vi "Beampointing_Multi_Pico2_upstairs02.vi"() -> ()   [LabVIEW 2013]
uses:
  GUI_Template/GUI_master/tcp_new_data_event.ctl
  GUI_Template/GUI_master/tcp new data cluster.ctl
  Ctrs/beam detection.ctl
  GUI_Beampointing_single_TRA/Ctrs/move.ctl
  <vilib>/Utility/error.llb/DialogType.ctl
  <vilib>/Utility/file.llb/Read From Spreadsheet File (string).vi
  <userlib>/_OpenG.lib/array/array.llb/Filter 1D Array with Scalar (String)__ogtk.vi
  <userlib>/_OpenG.lib/array/array.llb/Filter 1D Array (String)__ogtk.vi
  <vilib>/Utility/file.llb/Write To Spreadsheet File (string).vi
  <vilib>/Analysis/NI_AALBase.lvlib
panel:
  out "x-y*floor(x/y)":dbl
  out "error out":errorcluster
  out "config path":string
  out "Array 3":bool[](array[boolean])
  out "Array 2":u16[](array[numeric])
  out "Array":u16[](array[numeric])
  out "Moving Y":string
  out "Moving X":string
  out "particles":T1(array[cluster])
  out "millisecond timer value":u32
  out "appended path":path
  out "millisecond timer 2":u32
  in  "GUIdevice 98":string="PicoPad4"
  in  "Position.Axis 111::98":dbl=77.0 caption="Motor Axis 1" min=-30000.0 max=30000.0 format="%#_6f"
  in  "Position.Axis 112::98":dbl=77.0 caption="Motor Axis 1" min=-20000.0 max=20000.0 format="%#_6f"
  in  "Position.Axis 113::98":dbl=77.0 caption="Motor Axis 1" min=-20000.0 max=20000.0 format="%#_6f"
  in  "Position.Axis 121::98":dbl=77.0 caption="Motor Axis 1" min=-999999.0 max=999999.0 format="%#_6f"
  in  "Position.Axis 122::98":dbl=77.0 caption="Motor Axis 1" min=-999999.0 max=999999.0 format="%#_6f"
  in  "Position.Axis 123::98":dbl=77.0 caption="Motor Axis 1" min=-999999.0 max=999999.0 format="%#_6f"
  in  "Position.Axis 131::98":dbl=77.0 caption="Motor Axis 1" min=-999999.0 max=999999.0 format="%#_6f"
  in  "Position.Axis 132::98":dbl=77.0 caption="Motor Axis 1" min=-999999.0 max=999999.0 format="%#_6f"
  in  "Position.Axis 133::98":dbl=77.0 caption="Motor Axis 1" min=-999999.0 max=999999.0 format="%#_6f"
  in  "Position.Axis 141::98":dbl=77.0 caption="Motor Axis 1" min=-999999.0 max=999999.0 format="%#_6f"
  in  "Position.Axis 142::98":dbl=77.0 caption="Motor Axis 1" min=-999999.0 max=999999.0 format="%#_6f"
  in  "Position.Axis 143::98":dbl=77.0 caption="Motor Axis 1" min=-999999.0 max=999999.0 format="%#_6f"
  in  "Position.Axis 211::98":dbl=77.0 caption="Motor Axis 1" min=-999999.0 max=999999.0 format="%#_6f"
  in  "Position.Axis 212::98":dbl=77.0 caption="Motor Axis 1" min=-999999.0 max=999999.0 format="%#_6f"
  in  "Position.Axis 213::98":dbl=77.0 caption="Motor Axis 1" min=-999999.0 max=999999.0 format="%#_6f"
  in  "Position.Axis 221::98":dbl=77.0 caption="Motor Axis 1" min=-999999.0 max=999999.0 format="%#_6f"
  in  "Position.Axis 222::98":dbl=77.0 caption="Motor Axis 1" min=-999999.0 max=999999.0 format="%#_6f"
  in  "Position.Axis 223::98":dbl=77.0 caption="Motor Axis 1" min=-999999.0 max=999999.0 format="%#_6f"
  in  "Position.Axis 231::98":dbl=77.0 caption="Motor Axis 1" min=-999999.0 max=999999.0 format="%#_6f"
  in  "Position.Axis 232::98":dbl=77.0 caption="Motor Axis 1" min=-999999.0 max=999999.0 format="%#_6f"
  in  "Position.Axis 233::98":dbl=77.0 caption="Motor Axis 1" min=-999999.0 max=999999.0 format="%#_6f"
  in  "Position.Axis 241::98":dbl=77.0 caption="Motor Axis 1" min=-999999.0 max=999999.0 format="%#_6f"
  in  "Position.Axis 242::98":dbl=77.0 caption="Motor Axis 1" min=-999999.0 max=999999.0 format="%#_6f"
  in  "Position.Axis 243::98":dbl=77.0 caption="Motor Axis 1" min=-999999.0 max=999999.0 format="%#_6f"
  in  "Position.Axis 311::98":dbl=77.0 caption="Motor Axis 1" min=-999999.0 max=999999.0 format="%#_6f"
  in  "Position.Axis 312::98":dbl=77.0 caption="Motor Axis 1" min=-999999.0 max=999999.0 format="%#_6f"
  in  "Position.Axis 313::98":dbl=77.0 caption="Motor Axis 1" min=-999999.0 max=999999.0 format="%#_6f"
  in  "Position.Axis 321::98":dbl=77.0 caption="Motor Axis 1" min=-999999.0 max=999999.0 format="%#_6f"
  in  "Position.Axis 322::98":dbl=77.0 caption="Motor Axis 1" min=-999999.0 max=999999.0 format="%#_6f"
  in  "Position.Axis 323::98":dbl=77.0 caption="Motor Axis 1" min=-999999.0 max=999999.0 format="%#_6f"
  in  "Position.Axis 331::98":dbl=77.0 caption="Motor Axis 1" min=-999999.0 max=999999.0 format="%#_6f"
  in  "Position.Axis 332::98":dbl=77.0 caption="Motor Axis 1" min=-999999.0 max=999999.0 format="%#_6f"
  in  "Position.Axis 333::98":dbl=77.0 caption="Motor Axis 1" min=-999999.0 max=999999.0 format="%#_6f"
  in  "Position.Axis 341::98":dbl=77.0 caption="Motor Axis 1" min=-999999.0 max=999999.0 format="%#_6f"
  in  "Position.Axis 342::98":dbl=77.0 caption="Motor Axis 1" min=-999999.0 max=999999.0 format="%#_6f"
  in  "Position.Axis 343::98":dbl=77.0 caption="Motor Axis 1" min=-999999.0 max=999999.0 format="%#_6f"
  in  "Position.Axis 411::98":dbl=77.0 caption="Motor Axis 1" min=-999999.0 max=999999.0 format="%#_6f"
  in  "Position.Axis 412::98":dbl=77.0 caption="Motor Axis 1" min=-999999.0 max=999999.0 format="%#_6f"
  in  "Position.Axis 413::98":dbl=77.0 caption="Motor Axis 1" min=-999999.0 max=999999.0 format="%#_6f"
  in  "Position.Axis 421::98":dbl=77.0 caption="Motor Axis 1" min=-999999.0 max=999999.0 format="%#_6f"
  in  "Position.Axis 422::98":dbl=77.0 caption="Motor Axis 1" min=-999999.0 max=999999.0 format="%#_6f"
  in  "Position.Axis 423::98":dbl=77.0 caption="Motor Axis 1" min=-999999.0 max=999999.0 format="%#_6f"
  in  "Position.Axis 431::98":dbl=77.0 caption="Motor Axis 1" min=-999999.0 max=999999.0 format="%#_6f"
  in  "Position.Axis 432::98":dbl=77.0 caption="Motor Axis 1" min=-999999.0 max=999999.0 format="%#_6f"
  in  "Position.Axis 433::98":dbl=77.0 caption="Motor Axis 1" min=-999999.0 max=999999.0 format="%#_6f"
  in  "Position.Axis 441::98":dbl=77.0 caption="Motor Axis 1" min=-999999.0 max=999999.0 format="%#_6f"
  in  "Position.Axis 442::98":dbl=77.0 caption="Motor Axis 1" min=-999999.0 max=999999.0 format="%#_6f"
  in  "Position.Axis 443::98":dbl=77.0 caption="Motor Axis 1" min=-999999.0 max=999999.0 format="%#_6f"
  in  "Position.Axis 511::98":dbl=77.0 caption="Motor Axis 1" min=-999999.0 max=999999.0 format="%#_6f"
  in  "Position.Axis 512::98":dbl=77.0 caption="Motor Axis 1" min=-999999.0 max=999999.0 format="%#_6f"
  in  "Position.Axis 513::98":dbl=77.0 caption="Motor Axis 1" min=-999999.0 max=999999.0 format="%#_6f"
  in  "Position.Axis 521::98":dbl=77.0 caption="Motor Axis 1" min=-999999.0 max=999999.0 format="%#_6f"
  in  "Position.Axis 522::98":dbl=77.0 caption="Motor Axis 1" min=-999999.0 max=999999.0 format="%#_6f"
  in  "Position.Axis 523::98":dbl=77.0 caption="Motor Axis 1" min=-999999.0 max=999999.0 format="%#_6f"
  in  "Position.Axis 531::98":dbl=77.0 caption="Motor Axis 1" min=-999999.0 max=999999.0 format="%#_6f"
  in  "Position.Axis 532::98":dbl=77.0 caption="Motor Axis 1" min=-999999.0 max=999999.0 format="%#_6f"
  in  "Position.Axis 533::98":dbl=77.0 caption="Motor Axis 1" min=-999999.0 max=999999.0 format="%#_6f"
  in  "Position.Axis 541::98":dbl=77.0 caption="Motor Axis 1" min=-999999.0 max=999999.0 format="%#_6f"
  in  "Position.Axis 542::98":dbl=77.0 caption="Motor Axis 1" min=-999999.0 max=999999.0 format="%#_6f"
  in  "Position.Axis 543::98":dbl=77.0 caption="Motor Axis 1" min=-999999.0 max=999999.0 format="%#_6f"
  in  "Numeric":dbl
  out "Current State":string
  in  "output cluster 2":T5 {"detection para"."smal para"."Measurement Parameter" items=["Center of Mass X", "Center of Mass Y", "First Pixel X", "First Pixel Y", "Bounding Rect Left", "Bounding Rect Top", "Bounding Rect Right", "Bounding Rect Bottom", "Max Feret Diameter Start X", "Max Feret Diameter Start Y", "Max Feret Diameter End X", "Max Feret Diameter End Y", "Max Horiz. Segment Length Left", "Max Horiz. Segment Length Right", "Max Horiz. Segment Length Row", "-", "Bounding Rect Width", "Bounding Rect Height", "Bounding Rect Diagonal", "Perimeter", "Convex Hull Perimeter", "Holes' Perimeter", "Max Feret Diameter", "Equivalent Ellipse Major Axis", "Equivalent Ellipse Minor Axis", "Equivalent Ellipse Minor Axis (Feret)", "Equivalent Rect Long Side", "Equivalent Rect Short Side", "Equivalent Rect Diagonal", "Equivalent Rect Short Side (Feret)", "Average Horiz. Segment Length", "Average Vert. Segment Length", "Hydraulic Radius", "Waddel Disk Diameter", "-", "Area", "Holes' Area", "Particle & Holes' Area", "Convex Hull Area", "Image Area", "-", "Number of Holes", "Number of Horiz. Segments", "Number of Vert. Segments", "-", "Orientation", "Max Feret Diameter Orientation", "-", "% Area/Image Area", "% Area/(Particle & Holes' Area)", "Ratio of Equivalent Ellipse Axes", "Ratio of Equivalent Rect Sides", "-", "Elongation Factor", "Compactness Factor", "Heywood Circularity Factor", "Type Factor", "-", "Sum X", "Sum Y", "Sum XX", "Sum XY", "Sum YY", "Sum XXX", "Sum XXY", "Sum XYY", "Sum YYY", "-", "Moment of Inertia XX", "Moment of Inertia XY", "Moment of Inertia YY", "Moment of Inertia XXX", "Moment of Inertia XXY", "Moment of Inertia XYY", "Moment of Inertia YYY", "Norm. Moment of Inertia XX", "Norm. Moment of Inertia XY", "Norm. Moment of Inertia YY", "Norm. Moment of Inertia XXX", "Norm. Moment of Inertia XXY", "Norm. Moment of Inertia XYY", "Norm. Moment of Inertia YYY", "Hu Moment 1", "Hu Moment 2", "Hu Moment 3", "Hu Moment 4", "Hu Moment 5", "Hu Moment 6", "Hu Moment 7"]; "detection para"."smal para"."Range Lower Value" format="%.2f"; "detection para"."smal para"."Range Upper Value" format="%.2f"; "detection para"."detection method" items=["clustering", "entropy", "metric", "moments", "inter-class variance"]; "detection para"."Filter" items=["No Filter", "Median Filter", "Low Pass Filter"]}
  out "CCDs":string[](array[string])
  in  "GUIdevice 12":string
  in  "GUIdevice 11":string
  in  "GUIdevice 10":string
  in  "GUIdevice 9":string
  out "error out 2":errorcluster
  in  "active cams":string[](array[string])
  in  "Motor Y":dbl[][](array[numeric])
  in  "Motor X":dbl[][](array[numeric])
  out "Names":string[](array[string])
  in  "Offset X stats":dbl[][](array[numeric])
  in  "Offset Y stats":dbl[][](array[numeric])
  out "Box":T6(array[cluster])
  in  "Tab Control 2":enum32{"Config ", "Main", "History"}(tab)=enum."Main"
  out "Waveform Chart":u32(graph)
  in  "associated motors":T7
  out "Cameras":T8
  out "Status":cluster{i32, i32, "Centroid X":dbl[][]}(graph)
  in  "Exposure:12":dbl=0.095 min=0.0001 max=1.0 format="%#_6f"
  in  "Triggerdelay::12":dbl=0.003 min=0.0 max=0.09 format="%#_6f"
  in  "Exposure::11":dbl=0.095 min=0.0001 max=1.0 format="%#_6f"
  in  "Triggerdelay::11":dbl=0.003 min=0.0 max=0.09 format="%#_6f"
  in  "Exposure::10":dbl=0.095 min=0.0001 max=1.0 format="%#_6f"
  in  "Triggerdelay::10":dbl=0.003 min=0.0 max=0.09 format="%#_6f"
  in  "Exposure::9":dbl=0.095 min=0.0001 max=1.0 format="%#_6f"
  in  "Triggerdelay::9":dbl=0.003 min=0.0 max=0.09 format="%#_6f"
  in  "Trigger::9":bool
  in  "Trigger::10":bool caption="Trigger:10"
  in  "Trigger::11":bool
  in  "Trigger::12":bool
  in  "Target.Y::9":dbl=45.0 caption="T9y" min=0.0 max=2000.0 format="%#_6f"
  in  "Target.X::9":dbl=47.0 caption="Tx9" min=0.0 max=2000.0 format="%#_6f"
  in  "Target.Y::10":dbl=45.0 caption="T10y" min=0.0 max=2000.0 format="%#_6f"
  in  "Target.X::10":dbl=47.0 caption="T10x" min=0.0 max=2000.0 format="%#_6f"
  in  "Target.Y::11":dbl=45.0 caption="T11y" min=0.0 max=2000.0 format="%#_6f"
  in  "Target.X::11":dbl=47.0 caption="T11x" min=0.0 max=2000.0 format="%#_6f"
  in  "Target.Y::12":dbl=45.0 caption="T12y" min=0.0 max=2000.0 format="%#_6f"
  in  "Target.X::12":dbl=47.0 caption="T12x" min=0.0 max=2000.0 format="%#_6f"
  in  "Exposure::8":dbl=0.095 min=0.01 max=1.0 format="%#_6f"
  in  "Triggerdelay::8":dbl=0.003 min=0.0 max=0.09 format="%#_6f"
  in  "Trigger::8":bool
  in  "Target.Y::8":dbl=45.0 caption="T8y" min=0.0 max=2000.0 format="%#_6f"
  in  "Target.X::8":dbl=47.0 caption="T8x" min=0.0 max=2000.0 format="%#_6f"
  in  "Target.Y::7":dbl=45.0 caption="T7x" min=0.0 max=2000.0 format="%#_6f"
  in  "Target.X::7":dbl=47.0 caption="T7y" min=0.0 max=2000.0 format="%#_6f"
  in  "Target.Y::6":dbl=45.0 caption="T6y" min=0.0 max=2000.0 format="%#_6f"
  in  "Target.X::6":dbl=47.0 caption="T6x" min=0.0 max=2000.0 format="%#_6f"
  in  "Target.Y::5":dbl=45.0 caption="T5y" min=0.0 max=2000.0 format="%#_6f"
  in  "Target.X::5":dbl=47.0 caption="T5x" min=0.0 max=2000.0 format="%#_6f"
  in  "Target.Y::4":dbl=45.0 caption="T4y" min=0.0 max=2000.0 format="%#_6f"
  in  "Target.X::4":dbl=47.0 caption="T4x" min=0.0 max=2000.0 format="%#_6f"
  in  "Target.Y::3":dbl=163.0 caption="T3y" min=0.0 max=2000.0 format="%#_6f"
  in  "Target.X::3":dbl=152.0 caption="T3x" min=0.0 max=2000.0 format="%#_6f"
  in  "Target.Y::2":dbl=74.0 caption="T2y" min=0.0 max=2000.0 format="%#_6f"
  in  "Target.X::2":dbl=75.0 caption="T2x" min=0.0 max=2000.0 format="%#_6f"
  in  "Target.Y::1":dbl=61.0 caption="T1y" min=1.0 max=600.0 format="%#_6f"
  in  "Target.X::1":dbl=77.0 caption="T1x" min=1.0 max=800.0 format="%#_6f"
  in  "Exposure::7":dbl=0.095 min=0.0001 max=1.0 format="%#_6f"
  in  "Triggerdelay::7":dbl=0.003 min=0.0 max=0.09 format="%#_6f"
  in  "Trigger::7":bool
  in  "Exposure::6":dbl=0.095 min=0.0001 max=1.0 format="%#_6f"
  in  "Triggerdelay::6":dbl=0.003 min=0.0 max=0.09 format="%#_6f"
  in  "Trigger::6":bool
  in  "Exposure::5":dbl=0.095 min=0.0001 max=1.0 format="%#_6f"
  in  "Triggerdelay::5":dbl=0.003 min=0.0 max=0.09 format="%#_6f"
  in  "Trigger::5":bool
  in  "Exposure::4":dbl=0.095 min=0.0001 max=1.0 format="%#_6f"
  in  "Triggerdelay::4":dbl=0.003 min=0.0 max=0.09 format="%#_6f"
  in  "Trigger::4":bool
  in  "Exposure::3":dbl=0.095 min=0.0001 max=1.0 format="%#_6f"
  in  "Triggerdelay::3":dbl=0.003 min=0.0 max=0.09 format="%#_6f"
  in  "Trigger::3":bool
  in  "Exposure::2":dbl=0.095 min=0.0001 max=1.0 format="%#_6f"
  in  "Triggerdelay::2":dbl=0.003 min=0.0 max=0.09 format="%#_6f"
  in  "Trigger::2":bool
  out "image::1":T9(plugin-control) caption="XPW_cam"
  out "image::2":T9(plugin-control) caption="LM_Mirrorcam"
  out "image::3":T9(plugin-control) caption="LM_Focuscam"
  out "image::4":T9(plugin-control) caption="TS-253a_in"
  out "image::5":T9(plugin-control) caption="LM_Stagecam"
  out "image::6":T9(plugin-control)
  out "image::7":T9(plugin-control)
  out "image::8":T9(plugin-control)
  in  "Exposure::1":dbl=0.095 min=0.0001 max=1.0 format="%#_6f"
  in  "Triggerdelay::1":dbl=0.003 min=0.0 max=0.09 format="%#_6f"
  in  "Trigger::1":bool
  in  "UDP error message":string
  out "required Y":bool[](array[boolean])
  out "required X":bool[](array[boolean])
  out "detected":bool[](array[boolean])
  out "name array":string[](array[string])
  out "image::9":T9(plugin-control)
  out "image::10":T9(plugin-control)
  out "image::11":T9(plugin-control)
  out "image::12":T9(plugin-control)
  out "speedmode X":bool[](array[boolean])
  out "speedmode Y":bool[](array[boolean])
  out "CCD 9":cluster{timestamp[], dbl[]}[](graph)
  out "CCD 10":cluster{timestamp[], dbl[]}[](graph)
  out "CCD 11":cluster{timestamp[], dbl[]}[](graph)
  out "CCD 12":cluster{timestamp[], dbl[]}[](graph)
  out "CCD 5":cluster{timestamp[], dbl[]}[](graph)
  out "CCD 6":cluster{timestamp[], dbl[]}[](graph)
  out "CCD 7":cluster{timestamp[], dbl[]}[](graph)
  out "CCD 8":cluster{timestamp[], dbl[]}[](graph)
  out "CCD 2":cluster{timestamp[], dbl[]}[](graph)
  out "CCD 1":cluster{timestamp[], dbl[]}[](graph)
  out "CCD 3":cluster{timestamp[], dbl[]}[](graph)
  out "CCD 4":cluster{timestamp[], dbl[]}[](graph)
  out "History index":i32
  in  "History Size":i32=500
  out "Particle Reports (Pixels)":T10(array[cluster])
  in  "Feedback Global":bool
  in  "detection para":T3[](array[typedef])=[{"Filter"=1, "Filter Para"={"X Size"=5, "Y Size"=5, "% Tolerance"=1}, "detection method"=4, "smal para"=[{"Measurement Parameter"=35, "Range Lower Value"=0.0, "Range Upper Value"=0.0, "Range"=TRUE, "Measurement Type"=FALSE}], "Remove small Objects"=TRUE, "Restrict to round Objects"=FALSE}, {"Filter"=1, "Filter Para"={"X Size"=5, "Y Size"=5, "% Tolerance"=1}, "detection method"=4, "smal para"=[{"Measurement Parameter"=35, "Range Lower Value"=0.0, "Range Upper Value"=500.0, "Range"=FALSE, "Measurement Type"=FALSE}], "Remove small Objects"=TRUE, "Restrict to round Objects"=FALSE}, {"Filter"=1, "Filter Para"={"X Size"=5, "Y Size"=5, "% Tolerance"=1}, "detection method"=4, "smal para"=[{"Measurement Parameter"=35, "Range Lower Value"=0.0, "Range Upper Value"=500.0, "Range"=TRUE, "Measurement Type"=FALSE}], "Remove small Objects"=TRUE, "Restrict to round Objects"=FALSE}, {"Filter"=1, "Filter Para"={"X Size"=5, "Y Size"=5, "% Tolerance"=1}, "detection method"=4, "smal para"=[{"Measurement Parameter"=35, "Range Lower Value"=0.0, "Range Upper Value"=500.0, "Range"=TRUE, "Measurement Type"=FALSE}], "Remove small Objects"=TRUE, "Restrict to round Objects"=FALSE}, {"Filter"=1, "Filter Para"={"X Size"=5, "Y Size"=5, "% Tolerance"=1}, "detection method"=4, "smal para"=[{"Measurement Parameter"=35, "Range Lower Value"=0.0, "Range Upper Value"=500.0, "Range"=TRUE, "Measurement Type"=FALSE}], "Remove small Objects"=TRUE, "Restrict to round Objects"=FALSE}, {"Filter"=1, "Filter Para"={"X Size"=5, "Y Size"=5, "% Tolerance"=1}, "detection method"=4, "smal para"=[{"Measurement Parameter"=35, "Range Lower Value"=0.0, "Range Upper Value"=500.0, "Range"=TRUE, "Measurement Type"=FALSE}], "Remove small Objects"=TRUE, "Restrict to round Objects"=FALSE}, {"Filter"=1, "Filter Para"={"X Size"=5, "Y Size"=5, "% Tolerance"=1}, "detection method"=4, "smal para"=[{"Measurement Parameter"=35, "Range Lower Value"=0.0, "Range Upper Value"=500.0, "Range"=TRUE, "Measurement Type"=FALSE}], "Remove small Objects"=TRUE, "Restrict to round Objects"=FALSE}, {"Filter"=1, "Filter Para"={"X Size"=5, "Y Size"=5, "% Tolerance"=1}, "detection method"=3, "smal para"=[{"Measurement Parameter"=35, "Range Lower Value"=0.0, "Range Upper Value"=0.0, "Range"=FALSE, "Measurement Type"=FALSE}], "Remove small Objects"=TRUE, "Restrict to round Objects"=FALSE}, {"Filter"=1, "Filter Para"={"X Size"=5, "Y Size"=5, "% Tolerance"=1}, "detection method"=4, "smal para"=[{"Measurement Parameter"=35, "Range Lower Value"=0.0, "Range Upper Value"=0.0, "Range"=FALSE, "Measurement Type"=FALSE}], "Remove small Objects"=TRUE, "Restrict to round Objects"=FALSE}, {"Filter"=1, "Filter Para"={"X Size"=5, "Y Size"=5, "% Tolerance"=1}, "detection method"=4, "smal para"=[{"Measurement Parameter"=35, "Range Lower Value"=0.0, "Range Upper Value"=500.0, "Range"=TRUE, "Measurement Type"=FALSE}], "Remove small Objects"=TRUE, "Restrict to round Objects"=FALSE}, {"Filter"=1, "Filter Para"={"X Size"=5, "Y Size"=5, "% Tolerance"=1}, "detection method"=4, "smal para"=[{"Measurement Parameter"=35, "Range Lower Value"=0.0, "Range Upper Value"=500.0, "Range"=TRUE, "Measurement Type"=FALSE}], "Remove small Objects"=TRUE, "Restrict to round Objects"=FALSE}, {"Filter"=1, "Filter Para"={"X Size"=5, "Y Size"=5, "% Tolerance"=1}, "detection method"=4, "smal para"=[{"Measurement Parameter"=35, "Range Lower Value"=0.0, "Range Upper Value"=500.0, "Range"=TRUE, "Measurement Type"=FALSE}], "Remove small Objects"=TRUE, "Restrict to round Objects"=FALSE}] {"smal para"."Measurement Parameter" items=["Center of Mass X", "Center of Mass Y", "First Pixel X", "First Pixel Y", "Bounding Rect Left", "Bounding Rect Top", "Bounding Rect Right", "Bounding Rect Bottom", "Max Feret Diameter Start X", "Max Feret Diameter Start Y", "Max Feret Diameter End X", "Max Feret Diameter End Y", "Max Horiz. Segment Length Left", "Max Horiz. Segment Length Right", "Max Horiz. Segment Length Row", "-", "Bounding Rect Width", "Bounding Rect Height", "Bounding Rect Diagonal", "Perimeter", "Convex Hull Perimeter", "Holes' Perimeter", "Max Feret Diameter", "Equivalent Ellipse Major Axis", "Equivalent Ellipse Minor Axis", "Equivalent Ellipse Minor Axis (Feret)", "Equivalent Rect Long Side", "Equivalent Rect Short Side", "Equivalent Rect Diagonal", "Equivalent Rect Short Side (Feret)", "Average Horiz. Segment Length", "Average Vert. Segment Length", "Hydraulic Radius", "Waddel Disk Diameter", "-", "Area", "Holes' Area", "Particle & Holes' Area", "Convex Hull Area", "Image Area", "-", "Number of Holes", "Number of Horiz. Segments", "Number of Vert. Segments", "-", "Orientation", "Max Feret Diameter Orientation", "-", "% Area/Image Area", "% Area/(Particle & Holes' Area)", "Ratio of Equivalent Ellipse Axes", "Ratio of Equivalent Rect Sides", "-", "Elongation Factor", "Compactness Factor", "Heywood Circularity Factor", "Type Factor", "-", "Sum X", "Sum Y", "Sum XX", "Sum XY", "Sum YY", "Sum XXX", "Sum XXY", "Sum XYY", "Sum YYY", "-", "Moment of Inertia XX", "Moment of Inertia XY", "Moment of Inertia YY", "Moment of Inertia XXX", "Moment of Inertia XXY", "Moment of Inertia XYY", "Moment of Inertia YYY", "Norm. Moment of Inertia XX", "Norm. Moment of Inertia XY", "Norm. Moment of Inertia YY", "Norm. Moment of Inertia XXX", "Norm. Moment of Inertia XXY", "Norm. Moment of Inertia XYY", "Norm. Moment of Inertia YYY", "Hu Moment 1", "Hu Moment 2", "Hu Moment 3", "Hu Moment 4", "Hu Moment 5", "Hu Moment 6", "Hu Moment 7"]; "smal para"."Range Lower Value" format="%.2f"; "smal para"."Range Upper Value" format="%.2f"; "detection method" items=["clustering", "entropy", "metric", "moments", "inter-class variance"]; "Filter" items=["No Filter", "Median Filter", "Low Pass Filter"]}
  in  "GUIdevice 8":string="B5_CompressorOut"
  in  "Tab Control":T11(tab)
  in  "Center":bool
  in  "Save Stats":bool
  in  "Save Config":bool
  in  "Load Config":bool
  in  "update speed [ms]":i32=200
  in  "Img to avg":i32=20 min=3 max=200
  in  "Reset History":bool
  in  "save path":path=path "W:/BP_DATA"
  in  "autodetect":bool
  in  "Detection Rate":dbl=0.8 min=0.001 max=1.0
  in  "new tdms":bool
  in  "Speedmode @":dbl=3.0 min=1.0 max=20.0
  in  "Align":bool
  in  "deivice ini":bool
  in  "beam detection para":T3={"Filter"=1, "Filter Para"={"X Size"=5, "Y Size"=5, "% Tolerance"=1}, "detection method"=4, "smal para"=[{"Measurement Parameter"=35, "Range Lower Value"=0.0, "Range Upper Value"=500.0, "Range"=FALSE, "Measurement Type"=FALSE}], "Remove small Objects"=TRUE, "Restrict to round Objects"=FALSE} {"smal para"."Measurement Parameter" items=["Center of Mass X", "Center of Mass Y", "First Pixel X", "First Pixel Y", "Bounding Rect Left", "Bounding Rect Top", "Bounding Rect Right", "Bounding Rect Bottom", "Max Feret Diameter Start X", "Max Feret Diameter Start Y", "Max Feret Diameter End X", "Max Feret Diameter End Y", "Max Horiz. Segment Length Left", "Max Horiz. Segment Length Right", "Max Horiz. Segment Length Row", "-", "Bounding Rect Width", "Bounding Rect Height", "Bounding Rect Diagonal", "Perimeter", "Convex Hull Perimeter", "Holes' Perimeter", "Max Feret Diameter", "Equivalent Ellipse Major Axis", "Equivalent Ellipse Minor Axis", "Equivalent Ellipse Minor Axis (Feret)", "Equivalent Rect Long Side", "Equivalent Rect Short Side", "Equivalent Rect Diagonal", "Equivalent Rect Short Side (Feret)", "Average Horiz. Segment Length", "Average Vert. Segment Length", "Hydraulic Radius", "Waddel Disk Diameter", "-", "Area", "Holes' Area", "Particle & Holes' Area", "Convex Hull Area", "Image Area", "-", "Number of Holes", "Number of Horiz. Segments", "Number of Vert. Segments", "-", "Orientation", "Max Feret Diameter Orientation", "-", "% Area/Image Area", "% Area/(Particle & Holes' Area)", "Ratio of Equivalent Ellipse Axes", "Ratio of Equivalent Rect Sides", "-", "Elongation Factor", "Compactness Factor", "Heywood Circularity Factor", "Type Factor", "-", "Sum X", "Sum Y", "Sum XX", "Sum XY", "Sum YY", "Sum XXX", "Sum XXY", "Sum XYY", "Sum YYY", "-", "Moment of Inertia XX", "Moment of Inertia XY", "Moment of Inertia YY", "Moment of Inertia XXX", "Moment of Inertia XXY", "Moment of Inertia XYY", "Moment of Inertia YYY", "Norm. Moment of Inertia XX", "Norm. Moment of Inertia XY", "Norm. Moment of Inertia YY", "Norm. Moment of Inertia XXX", "Norm. Moment of Inertia XXY", "Norm. Moment of Inertia XYY", "Norm. Moment of Inertia YYY", "Hu Moment 1", "Hu Moment 2", "Hu Moment 3", "Hu Moment 4", "Hu Moment 5", "Hu Moment 6", "Hu Moment 7"]; "smal para"."Range Lower Value" format="%.2f"; "smal para"."Range Upper Value" format="%.2f"; "detection method" items=["clustering", "entropy", "metric", "moments", "inter-class variance"]; "Filter" items=["No Filter", "Median Filter", "Low Pass Filter"]}
  in  "move config":T2={"Tolerance [%]"=0.1, "Stepsize"=0.0001, "Invert Axis"=TRUE, "Invert Direction X"=FALSE, "Invert Direction Y"=TRUE, "enable feedback"=FALSE, "Set Centriod Target"=FALSE}
  in  "ActiveMotor":u16(ring)=7 items=["XPW OUT SAL", "Pre-IN-SAL", "XPW_cam", "L1_TelInpNear", "A", "B", "a", "D", "PRE-3RD-OUT", "TSa", "", "", "Focuscam", "Mirrorcam", "", "", "", "", "", ""]
  in  "ActiveMotorName::99":string
  in  "RelativeMove.Axis 1.CCW::99":bool caption="RelativeMove.Axis 1.CCW::1"
  in  "RelativeMove.Axis 1.CW::99":bool caption="RelativeMove.Axis 1.CW::1"
  in  "RelativeMove.Axis 2.CCW::99":bool caption="RelativeMove.Axis. 2.CCW::1"
  in  "RelativeMove.Axis 2.CW::99":bool caption="RelativeMove.Axis 2.CW::1"
  in  "RelativeSettings.Axis 1.Position::99":dbl caption="Axis 1 Position" min=-999999.0 max=999999.0 format="%_4p"
  in  "RelativeSettings.Axis 2.Position::99":dbl caption="Axis 2 Position" min=-999999.0 max=999999.0 format="%_4p"
  in  "RelativeSettings.Axis 2.StepSize::99":dbl=50.0 caption="Axis 2 StepSize" min=0.0 max=999999.0 format="%_4p"
  in  "RelativeSettings.Axis 1.StepSize::99":dbl=50.0 caption="Axis 1 Stepsize" min=0.0 max=999999.0 format="%_4p"
  out "Arguments Y":string
  in  "active axis refs 2":T12(array[cluster])
  in  "active Axis ref":cluster{"Ref X":refnum<vi>, "Ref Y":refnum<vi>}
  in  "CCDs":u16(ring) items=["XPW_cam", "LM_Mirrorcam", "LM_Focuscam", "TS-253a_in", "LM_Stagecam", "", "", "", "", "", "", ""]
  out "motor refs":refnum<vi>[](array[refnum])
  in  "Position.Axis 511::99":dbl=77.0 caption="Motor Axis 1" min=-999999.0 max=999999.0 format="%#_6f"
  in  "Position.Axis 512::99":dbl=77.0 caption="Motor Axis 1" min=-999999.0 max=999999.0 format="%#_6f"
  in  "Position.Axis 513::99":dbl=77.0 caption="Motor Axis 1" min=-999999.0 max=999999.0 format="%#_6f"
  in  "Position.Axis 521::99":dbl=77.0 caption="Motor Axis 1" min=-999999.0 max=999999.0 format="%#_6f"
  in  "Position.Axis 522::99":dbl=77.0 caption="Motor Axis 1" min=-999999.0 max=999999.0 format="%#_6f"
  in  "Position.Axis 523::99":dbl=77.0 caption="Motor Axis 1" min=-999999.0 max=999999.0 format="%#_6f"
  in  "Position.Axis 531::99":dbl=77.0 caption="Motor Axis 1" min=-999999.0 max=999999.0 format="%#_6f"
  in  "Position.Axis 532::99":dbl=77.0 caption="Motor Axis 1" min=-999999.0 max=999999.0 format="%#_6f"
  in  "Position.Axis 533::99":dbl=77.0 caption="Motor Axis 1" min=-999999.0 max=999999.0 format="%#_6f"
  in  "Position.Axis 541::99":dbl=77.0 caption="Motor Axis 1" min=-999999.0 max=999999.0 format="%#_6f"
  in  "Position.Axis 542::99":dbl=77.0 caption="Motor Axis 1" min=-999999.0 max=999999.0 format="%#_6f"
  in  "Position.Axis 543::99":dbl=77.0 caption="Motor Axis 1" min=-999999.0 max=999999.0 format="%#_6f"
  in  "Position.Axis 411::99":dbl=77.0 caption="Motor Axis 1" min=-999999.0 max=999999.0 format="%#_6f"
  in  "Position.Axis 412::99":dbl=77.0 caption="Motor Axis 1" min=-999999.0 max=999999.0 format="%#_6f"
  in  "Position.Axis 413::99":dbl=77.0 caption="Motor Axis 1" min=-999999.0 max=999999.0 format="%#_6f"
  in  "Position.Axis 421::99":dbl=77.0 caption="Motor Axis 1" min=-999999.0 max=999999.0 format="%#_6f"
  in  "Position.Axis 422::99":dbl=77.0 caption="Motor Axis 1" min=-999999.0 max=999999.0 format="%#_6f"
  in  "Position.Axis 423::99":dbl=77.0 caption="Motor Axis 1" min=-999999.0 max=999999.0 format="%#_6f"
  in  "Position.Axis 431::99":dbl=77.0 caption="Motor Axis 1" min=-999999.0 max=999999.0 format="%#_6f"
  in  "Position.Axis 432::99":dbl=77.0 caption="Motor Axis 1" min=-999999.0 max=999999.0 format="%#_6f"
  in  "Position.Axis 433::99":dbl=77.0 caption="Motor Axis 1" min=-999999.0 max=999999.0 format="%#_6f"
  in  "Position.Axis 441::99":dbl=77.0 caption="Motor Axis 1" min=-999999.0 max=999999.0 format="%#_6f"
  in  "Position.Axis 442::99":dbl=77.0 caption="Motor Axis 1" min=-999999.0 max=999999.0 format="%#_6f"
  in  "Position.Axis 443::99":dbl=77.0 caption="Motor Axis 1" min=-999999.0 max=999999.0 format="%#_6f"
  in  "Position.Axis 311::99":dbl=77.0 caption="Motor Axis 1" min=-999999.0 max=999999.0 format="%#_6f"
  in  "Position.Axis 312::99":dbl=77.0 caption="Motor Axis 1" min=-999999.0 max=999999.0 format="%#_6f"
  in  "Position.Axis 313::99":dbl=77.0 caption="Motor Axis 1" min=-999999.0 max=999999.0 format="%#_6f"
  in  "Position.Axis 321::99":dbl=77.0 caption="Motor Axis 1" min=-999999.0 max=999999.0 format="%#_6f"
  in  "Position.Axis 322::99":dbl=77.0 caption="Motor Axis 1" min=-999999.0 max=999999.0 format="%#_6f"
  in  "Position.Axis 323::99":dbl=77.0 caption="Motor Axis 1" min=-999999.0 max=999999.0 format="%#_6f"
  in  "Position.Axis 331::99":dbl=77.0 caption="Motor Axis 1" min=-999999.0 max=999999.0 format="%#_6f"
  in  "Position.Axis 332::99":dbl=77.0 caption="Motor Axis 1" min=-999999.0 max=999999.0 format="%#_6f"
  in  "Position.Axis 333::99":dbl=77.0 caption="Motor Axis 1" min=-999999.0 max=999999.0 format="%#_6f"
  in  "Position.Axis 341::99":dbl=77.0 caption="Motor Axis 1" min=-999999.0 max=999999.0 format="%#_6f"
  in  "Position.Axis 342::99":dbl=77.0 caption="Motor Axis 1" min=-999999.0 max=999999.0 format="%#_6f"
  in  "Position.Axis 343::99":dbl=77.0 caption="Motor Axis 1" min=-999999.0 max=999999.0 format="%#_6f"
  in  "Position.Axis 241::99":dbl=77.0 caption="Motor Axis 1" min=-999999.0 max=999999.0 format="%#_6f"
  in  "Position.Axis 242::99":dbl=77.0 caption="Motor Axis 1" min=-999999.0 max=999999.0 format="%#_6f"
  in  "Position.Axis 243::99":dbl=77.0 caption="Motor Axis 1" min=-999999.0 max=999999.0 format="%#_6f"
  in  "Position.Axis 231::99":dbl=77.0 caption="Motor Axis 1" min=-999999.0 max=999999.0 format="%#_6f"
  in  "Position.Axis 232::99":dbl=77.0 caption="Motor Axis 1" min=-999999.0 max=999999.0 format="%#_6f"
  in  "Position.Axis 233::99":dbl=77.0 caption="Motor Axis 1" min=-999999.0 max=999999.0 format="%#_6f"
  in  "Position.Axis 221::99":dbl=77.0 caption="Motor Axis 1" min=-999999.0 max=999999.0 format="%#_6f"
  in  "Position.Axis 222::99":dbl=77.0 caption="Motor Axis 1" min=-999999.0 max=999999.0 format="%#_6f"
  in  "Position.Axis 223::99":dbl=77.0 caption="Motor Axis 1" min=-999999.0 max=999999.0 format="%#_6f"
  in  "Position.Axis 211::99":dbl=77.0 caption="Motor Axis 1" min=-999999.0 max=999999.0 format="%#_6f"
  in  "Position.Axis 212::99":dbl=77.0 caption="Motor Axis 1" min=-999999.0 max=999999.0 format="%#_6f"
  in  "Position.Axis 213::99":dbl=77.0 caption="Motor Axis 1" min=-999999.0 max=999999.0 format="%#_6f"
  in  "Position.Axis 141::99":dbl=77.0 caption="Motor Axis 1" min=-999999.0 max=999999.0 format="%#_6f"
  in  "Position.Axis 142::99":dbl=77.0 caption="Motor Axis 1" min=-999999.0 max=999999.0 format="%#_6f"
  in  "Position.Axis 143::99":dbl=77.0 caption="Motor Axis 1" min=-999999.0 max=999999.0 format="%#_6f"
  in  "Position.Axis 131::99":dbl=77.0 caption="Motor Axis 1" min=-999999.0 max=999999.0 format="%#_6f"
  in  "Position.Axis 132::99":dbl=77.0 caption="Motor Axis 1" min=-999999.0 max=999999.0 format="%#_6f"
  in  "Position.Axis 133::99":dbl=77.0 caption="Motor Axis 1" min=-999999.0 max=999999.0 format="%#_6f"
  in  "Position.Axis 121::99":dbl=77.0 caption="Motor Axis 1" min=-999999.0 max=999999.0 format="%#_6f"
  in  "Position.Axis 122::99":dbl=77.0 caption="Motor Axis 1" min=-999999.0 max=999999.0 format="%#_6f"
  in  "Position.Axis 123::99":dbl=77.0 caption="Motor Axis 1" min=-999999.0 max=999999.0 format="%#_6f"
  in  "Position.Axis 113::99":dbl=77.0 caption="Motor Axis 1" min=-999999.0 max=999999.0 format="%#_6f"
  in  "Position.Axis 112::99":dbl=77.0 caption="Motor Axis 1" min=-999999.0 max=999999.0 format="%#_6f"
  in  "Position.Axis 111::99":dbl=77.0 caption="Motor Axis 1" min=-999999.0 max=999999.0 format="%#_6f"
  out "Arguments X":string
  in  "GUIdevice 99":string="Picopad23"
  in  "move properties":T2[](array[typedef])=[{"Tolerance [%]"=0.1, "Stepsize"=0.0001, "Invert Axis"=TRUE, "Invert Direction X"=FALSE, "Invert Direction Y"=TRUE, "enable feedback"=FALSE, "Set Centriod Target"=FALSE}, {"Tolerance [%]"=0.1, "Stepsize"=0.0001, "Invert Axis"=TRUE, "Invert Direction X"=FALSE, "Invert Direction Y"=TRUE, "enable feedback"=FALSE, "Set Centriod Target"=FALSE}, {"Tolerance [%]"=0.1, "Stepsize"=0.0001, "Invert Axis"=TRUE, "Invert Direction X"=FALSE, "Invert Direction Y"=TRUE, "enable feedback"=FALSE, "Set Centriod Target"=FALSE}, {"Tolerance [%]"=0.1, "Stepsize"=0.0001, "Invert Axis"=TRUE, "Invert Direction X"=FALSE, "Invert Direction Y"=TRUE, "enable feedback"=FALSE, "Set Centriod Target"=FALSE}, {"Tolerance [%]"=0.1, "Stepsize"=0.0001, "Invert Axis"=TRUE, "Invert Direction X"=FALSE, "Invert Direction Y"=TRUE, "enable feedback"=FALSE, "Set Centriod Target"=FALSE}, {"Tolerance [%]"=0.1, "Stepsize"=0.0001, "Invert Axis"=TRUE, "Invert Direction X"=FALSE, "Invert Direction Y"=TRUE, "enable feedback"=FALSE, "Set Centriod Target"=FALSE}, {"Tolerance [%]"=0.1, "Stepsize"=0.0001, "Invert Axis"=TRUE, "Invert Direction X"=FALSE, "Invert Direction Y"=TRUE, "enable feedback"=FALSE, "Set Centriod Target"=FALSE}, {"Tolerance [%]"=0.1, "Stepsize"=0.0001, "Invert Axis"=TRUE, "Invert Direction X"=FALSE, "Invert Direction Y"=TRUE, "enable feedback"=FALSE, "Set Centriod Target"=FALSE}, {"Tolerance [%]"=0.1, "Stepsize"=0.0001, "Invert Axis"=TRUE, "Invert Direction X"=FALSE, "Invert Direction Y"=TRUE, "enable feedback"=FALSE, "Set Centriod Target"=FALSE}, {"Tolerance [%]"=0.1, "Stepsize"=0.0001, "Invert Axis"=TRUE, "Invert Direction X"=FALSE, "Invert Direction Y"=TRUE, "enable feedback"=FALSE, "Set Centriod Target"=FALSE}, {"Tolerance [%]"=0.1, "Stepsize"=0.0001, "Invert Axis"=TRUE, "Invert Direction X"=FALSE, "Invert Direction Y"=TRUE, "enable feedback"=FALSE, "Set Centriod Target"=FALSE}, {"Tolerance [%]"=0.1, "Stepsize"=0.0001, "Invert Axis"=TRUE, "Invert Direction X"=FALSE, "Invert Direction Y"=TRUE, "enable feedback"=FALSE, "Set Centriod Target"=FALSE}, {"Tolerance [%]"=0.1, "Stepsize"=0.0001, "Invert Axis"=TRUE, "Invert Direction X"=FALSE, "Invert Direction Y"=TRUE, "enable feedback"=FALSE, "Set Centriod Target"=FALSE}]
  in  "Time":timestamp[][](array[timestamp])
  in  "Mean Size":dbl[][](array[numeric])
  in  "Size":dbl[][](array[numeric])
  in  "active CCDs":i32(listbox)=1
  in  "Offset Y":dbl[][](array[numeric])
  in  "Offset X":dbl[][](array[numeric])
  in  "Mean Centroid X":dbl[][](array[numeric])
  in  "Mean Centroid Y":dbl[][](array[numeric])
  in  "Centroid Y":dbl[][](array[numeric])
  in  "Centroid X":dbl[][](array[numeric])
  in  "GUIdevice 7":string="B2_TelLens1"
  in  "GUIdevice 6":string="B1_TelInput"
  in  "GUIdevice 5":string="L8_M10Leak"
  in  "GUIdevice 4":string="L7_TREXPass4"
  in  "GUIdevice 3":string="L6_TREXpass3"
  in  "GUIdevice 2":string="L5_TREXPass2"
  in  "insert tag":bool=TRUE
  in  "stop":bool
  in  "GUIdevice 1":string="L4_TREXpass1"
  out "tcp data event":T13
  out "error IO 2":errorcluster
  # "x [Tolerance]"
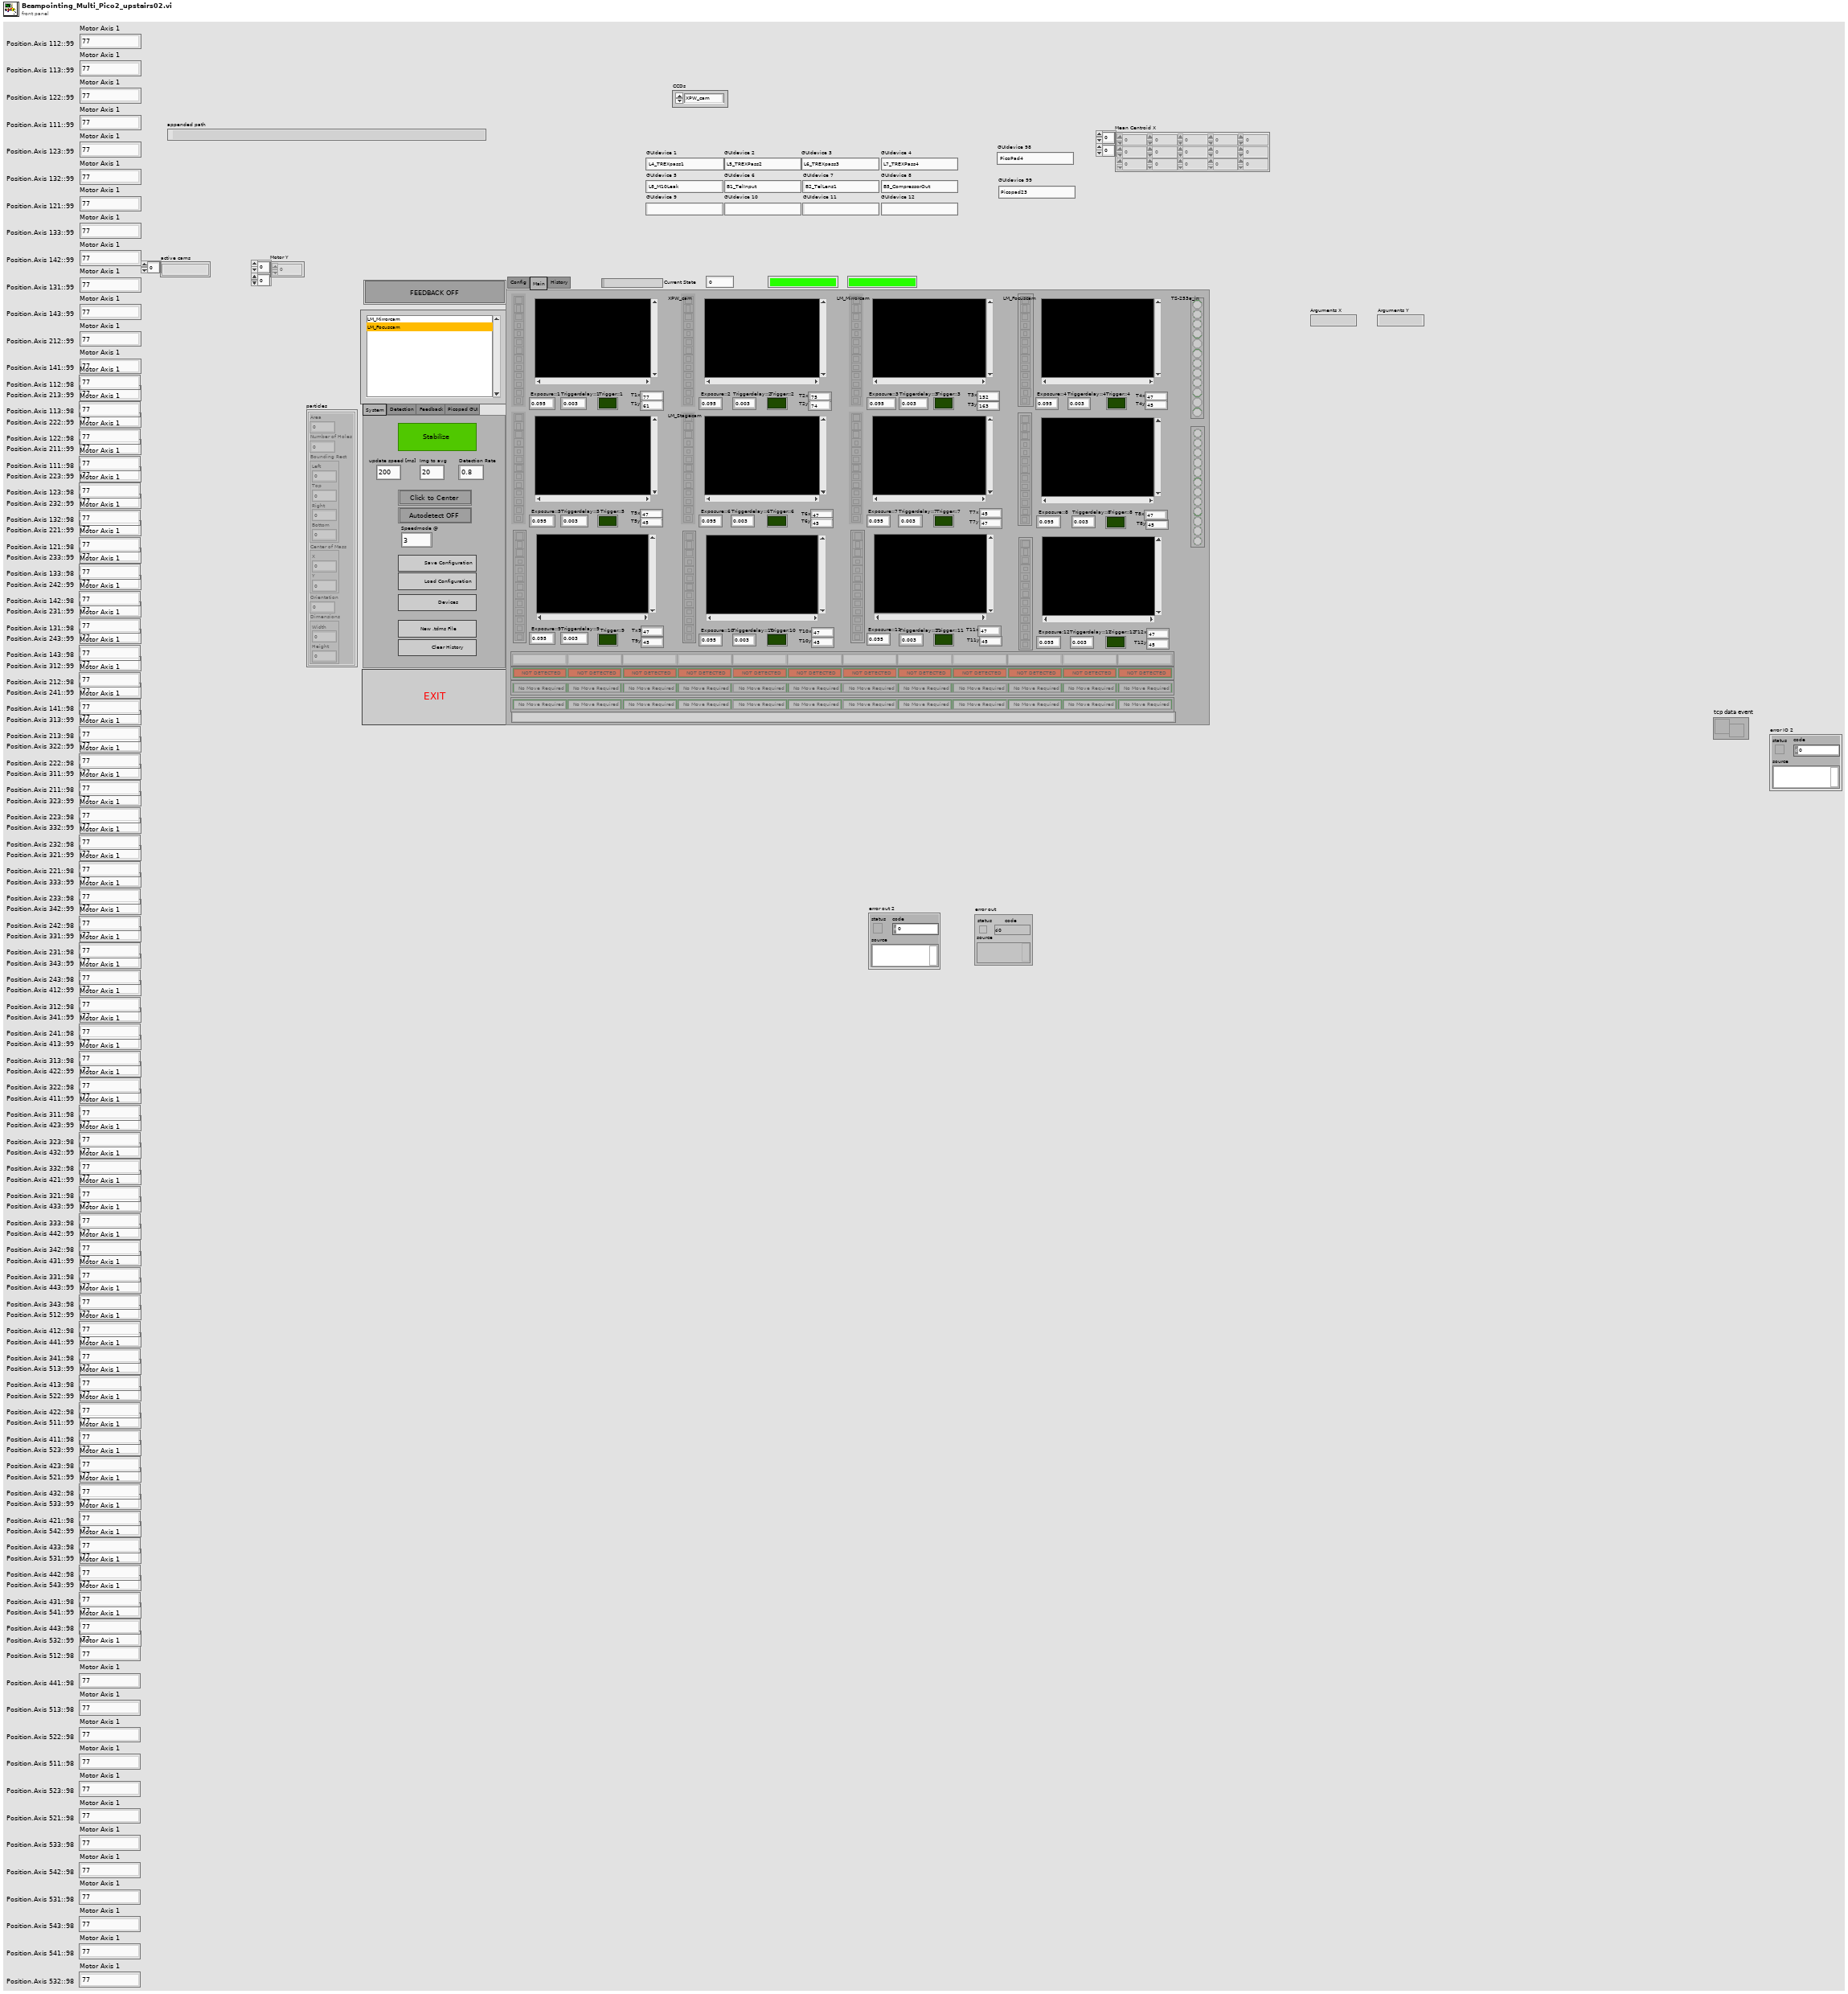
[diagram p1: front panel]
types:
  T1 = cluster{"Area":dbl, "Number of Holes":dbl, "Bounding Rect":cluster{"Left":dbl, "Top":dbl, "Right":dbl, "Bottom":dbl}, "Center of Mass":cluster{"X":dbl, "Y":dbl}, "Orientation":dbl, "Dimensions":cluster{"Width":dbl, "Height":dbl}}[]
  T2 = typedef "move.ctl" = cluster{"Tolerance [%]":dbl, "Stepsize":dbl, "Invert Axis":bool, "Invert Direction X":bool, "Invert Direction Y":bool, "enable feedback":bool, "Set Centriod Target":bool}
  T3 = typedef "beam detection.ctl" = cluster{"Filter":u16, "Filter Para":cluster{"X Size":i32, "Y Size":i32, "% Tolerance":i32}, "detection method":i32, "smal para":cluster{"Measurement Parameter":T4, "Range Lower Value":dbl, "Range Upper Value":dbl, "Range":bool, "Measurement Type":bool}[], "Remove small Objects":bool, "Restrict to round Objects":bool}
  T4 = typedef "Particle Parameters" = i32
  T5 = cluster{"CCDs":string[], "move properties":T2[], "detection para":T3[], "thresholds":cluster{"Lower value":sgl, "Upper value":sgl}[], "Value":cluster{"Motor CCD 1":u16, "Motor CCD 2":u16, "Motor CCD 3":u16, "Motor CCD 4":u16, "Motor CCD 5":u16, "Motor CCD 6":u16, "Motor CCD 7":u16, "Motor CCD 8":u16, "Motor CCD 9":u16, "Motor CCD 10":u16, "Motor CCD 11":u16, "Motor CCD 12":u16}}
  T6 = cluster{"Left":dbl, "Top":dbl, "Right":dbl, "Bottom":dbl}[]
  T7 = cluster{"Motor CCD 1":u16, "Motor CCD 2":u16, "Motor CCD 3":u16, "Motor CCD 4":u16, "Motor CCD 5":u16, "Motor CCD 6":u16, "Motor CCD 7":u16, "Motor CCD 8":u16, "Motor CCD 9":u16, "Motor CCD 10":u16, "Motor CCD 11":u16, "Motor CCD 12":u16}
  T8 = cluster{"[0]":string, "[1]":string, "[2]":string, "[3]":string, "[4]":string, "[5]":string, "[6]":string, "[7]":string, "[8]":string, "[8] 2":string, "[8] 3":string, "[8] 4":string}
  T9 = typedef "IMAQ Image.ctl" = refnum<image>
  T10 = cluster{"Area":dbl, "Number of Holes":dbl, "Bounding Rect":cluster{"Left":dbl, "Top":dbl, "Right":dbl, "Bottom":dbl}, "Center of Mass":cluster{"X":dbl, "Y":dbl}, "Orientation":dbl, "Dimensions":cluster{"Width":dbl, "Height":dbl}}[][]
  T11 = enum32{"System", "Detection", "Feedback", "Picopad GUI"}
  T12 = cluster{"Ref X":refnum<vi>, "Ref Y":refnum<vi>}[]
  T13 = typedef "tcp_new_data_event.ctl" = refnum<user-event>
  T14 = typedef "tcp new data cluster.ctl" = cluster{"EventEnum":enum16{"new data", "connection status update"}, "Device name":string}
  T15 = cluster{"Left":i32, "Top":i32, "Right":i32, "Bottom":i32}
  T16 = enum32{"invalid app kind", "Development System", "Run Time System", "Student Edition", "Embedded LabVIEW", "Evaluation", "Custom"}
  T17 = enum16{"open", "open or create", "create or replace", "create", "open (read-only)"}
  T18 = enum32{"Invalid", "Standard", "Closed", "Hidden", "Minimized", "Maximized"}
  T19 = enum16{"open", "replace", "create", "open or create", "replace or create", "replace or create with confirmation"}
  T20 = typedef "Image Type" = u32
  T21 = cluster{"[0]":string, "[1]":string, "[2]":string, "[3]":string, "[4]":string, "[5]":string, "[6]":string, "[7]":string, "[8]":string, "[9]":string, "[10]":string, "[11]":string}
  T22 = cluster{"Target.X::1":refnum<vi>, "Target.Y::1":refnum<vi>}
  T23 = cluster{"Target.X::2":refnum<vi>, "Target.Y::2":refnum<vi>}
  T24 = cluster{"Target.X::3":refnum<vi>, "Target.Y::3":refnum<vi>}
  T25 = cluster{"Target.X::4":refnum<vi>, "Target.Y::4":refnum<vi>}
  T26 = cluster{"Target.X::5":refnum<vi>, "Target.Y::5":refnum<vi>}
  T27 = cluster{"Target.X::6":refnum<vi>, "Target.Y::6":refnum<vi>}
  T28 = cluster{"Target.X::7":refnum<vi>, "Target.Y::7":refnum<vi>}
  T29 = cluster{"Target.X::8":refnum<vi>, "Target.Y::8":refnum<vi>}
  T30 = cluster{"Target.X::12":refnum<vi>, "Target.Y::12":refnum<vi>}
  T31 = cluster{"Target.X::9":refnum<vi>, "Target.Y::9":refnum<vi>}
  T32 = cluster{"Target.X::10":refnum<vi>, "Target.Y::10":refnum<vi>}
  T33 = cluster{"Target.X::11":refnum<vi>, "Target.Y::11":refnum<vi>}
  T34 = cluster{"Target.X::12":refnum<vi>, "Target.Y::12":refnum<vi>}[]
  T35 = cluster{"Left":dbl, "Top":dbl, "Right":dbl, "Bottom":dbl}
  T36 = cluster{"Core":cluster{"Current VI Reference":refnum<vi>, "Close Panel on Exit?":bool}, "detection para":T3[], "thresholds":cluster{"Lower value":sgl, "Upper value":sgl}[], "Centroid X":dbl[][], "Centroid Y":dbl[][], "img to avg":i32, "Mean Centroid X":dbl[][], "Mean Centroid Y":dbl[][], "Offset X":dbl[][], "Offset Y":dbl[][], "Offset X stats ":dbl[][], "Offset Y stats ":dbl[][], "Size":dbl[][], "Mean Size":dbl[][], "Time":timestamp[][], "move properties":T2[], "active axis refs 2":cluster{"Ref X":refnum<vi>, "Ref Y":refnum<vi>}[], "active ccd":i32, "Feedback global":bool, "Motor X":dbl[][], "Motor Y":dbl[][], "active cams":string[], "Data Value Reference out":refnum<k34>, "detected":bool[], "speedmode X":bool[], "speedmode Y":bool[]}
  T37 = typedef "DialogType.ctl" = u16
  T38 = cluster{"Current VI Reference":refnum<vi>, "Close Panel on Exit?":bool}
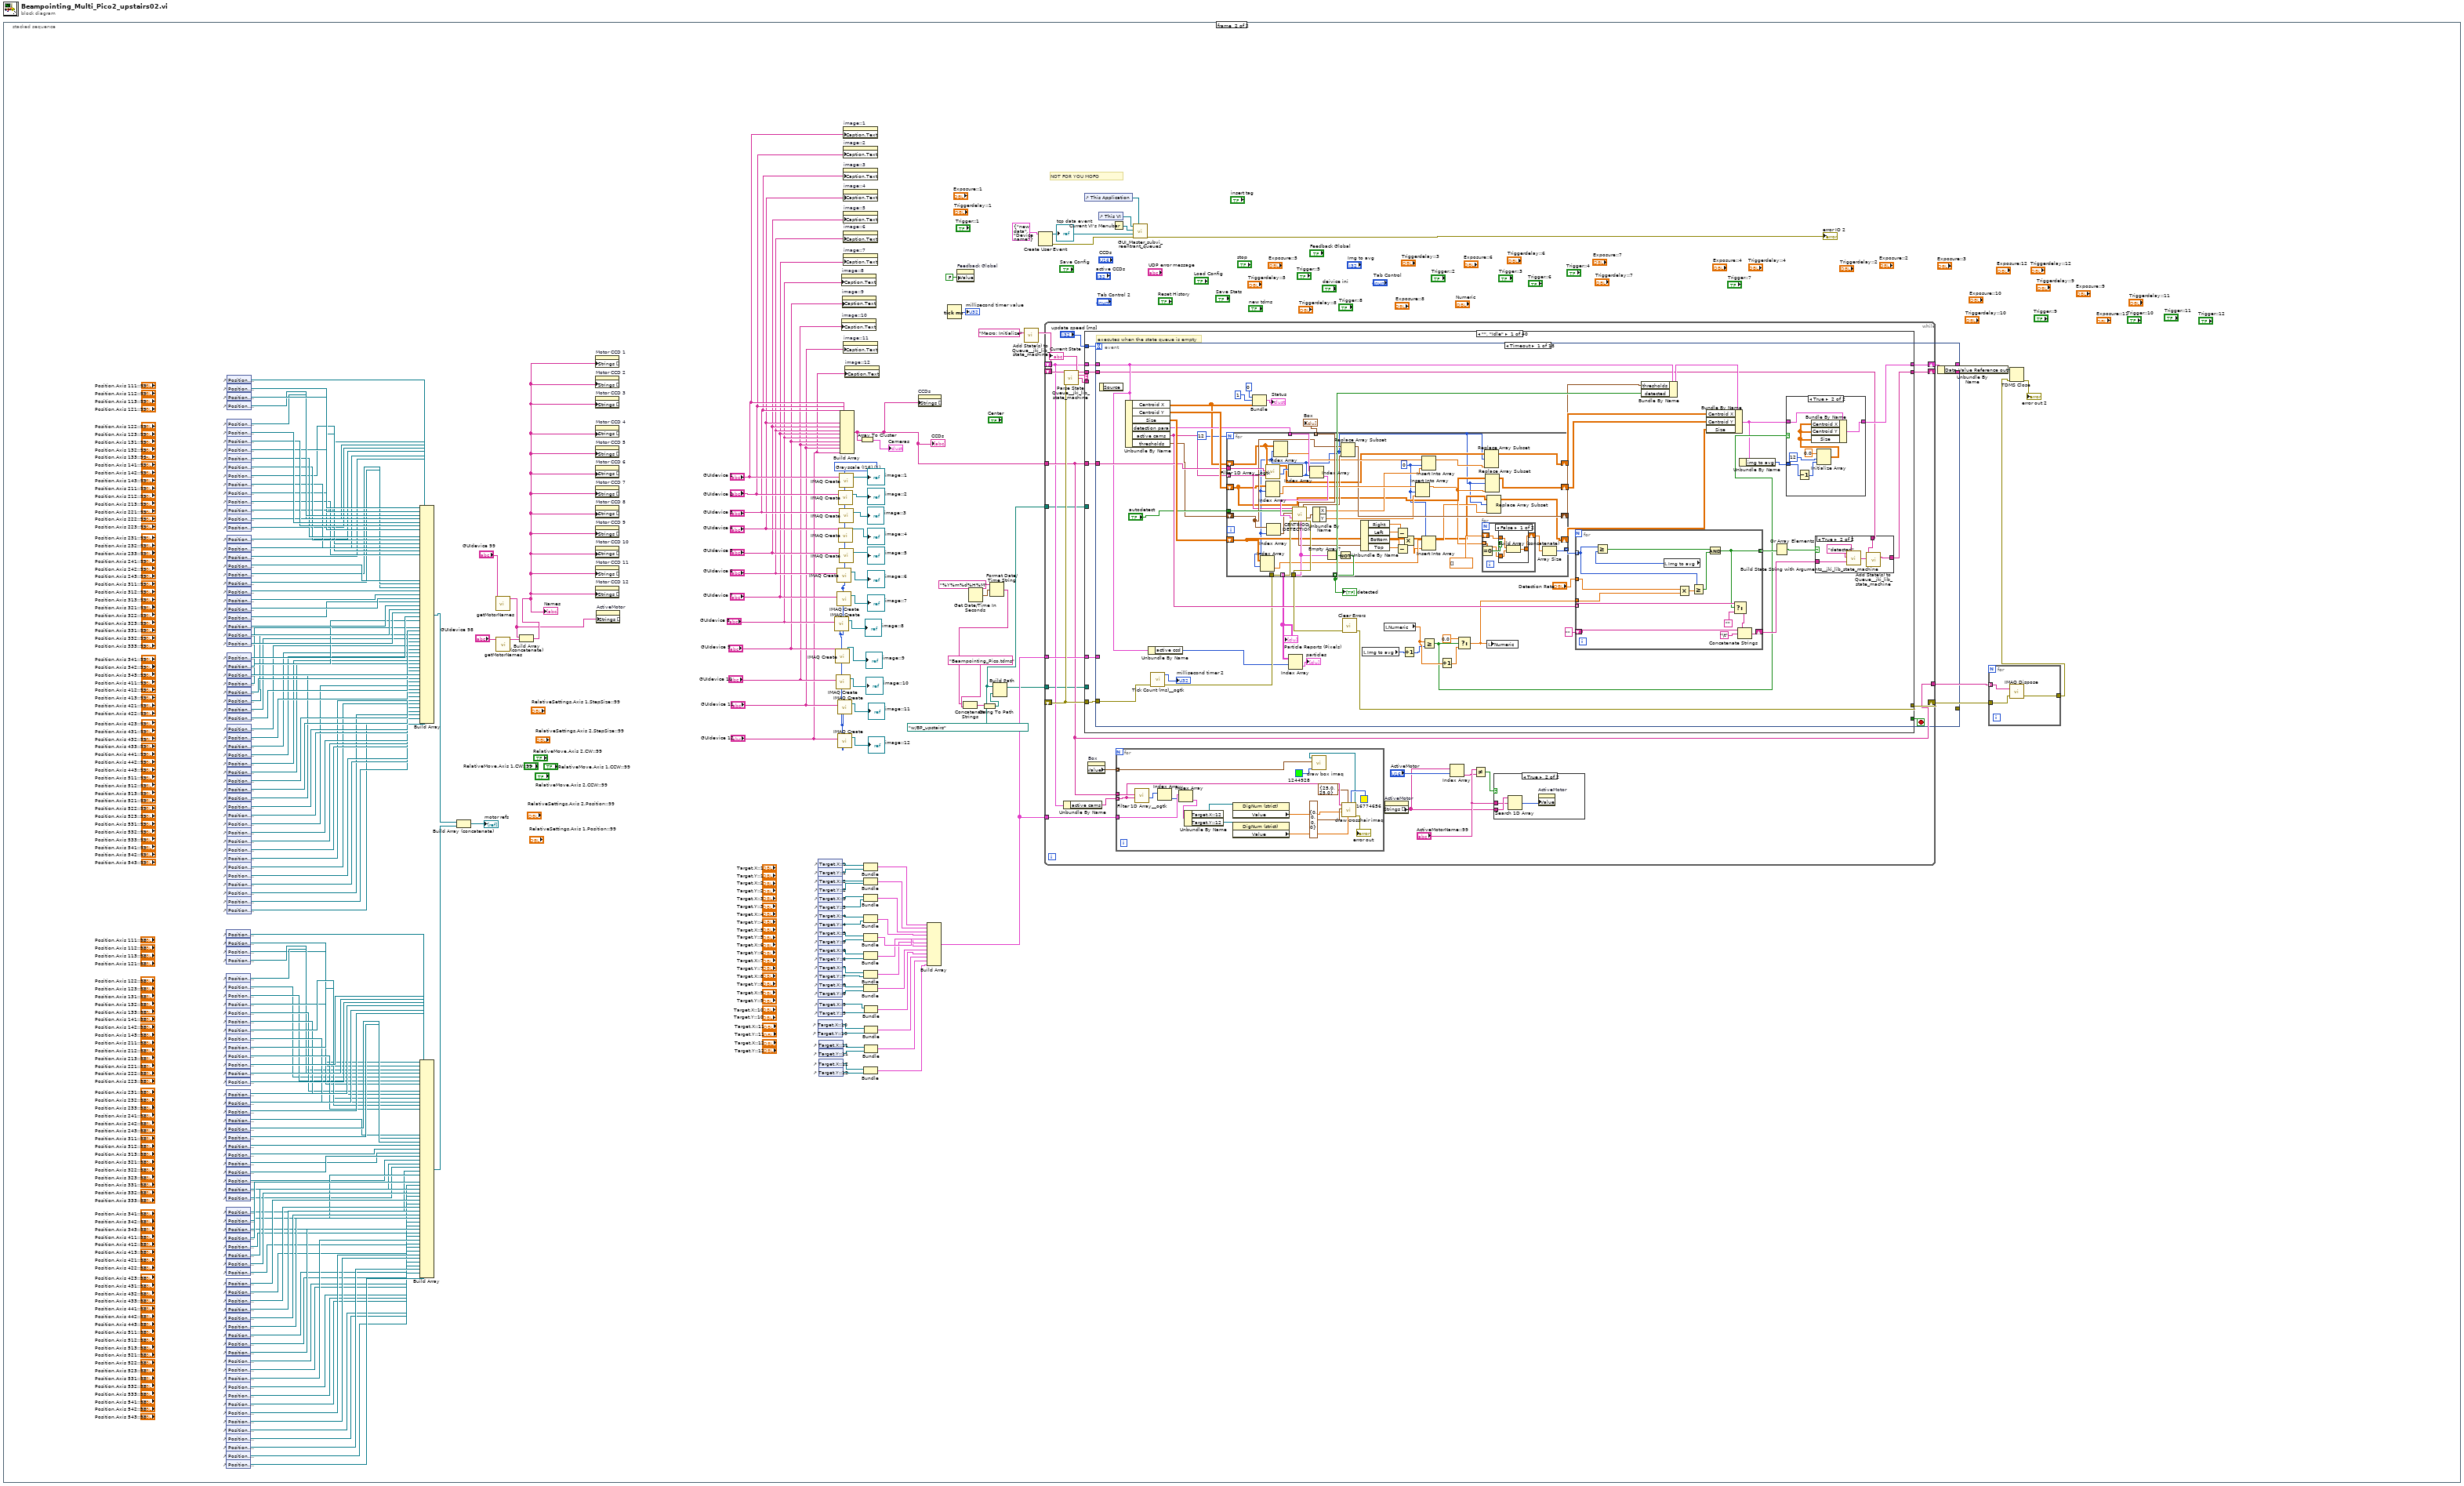
[diagram p0: block diagram]
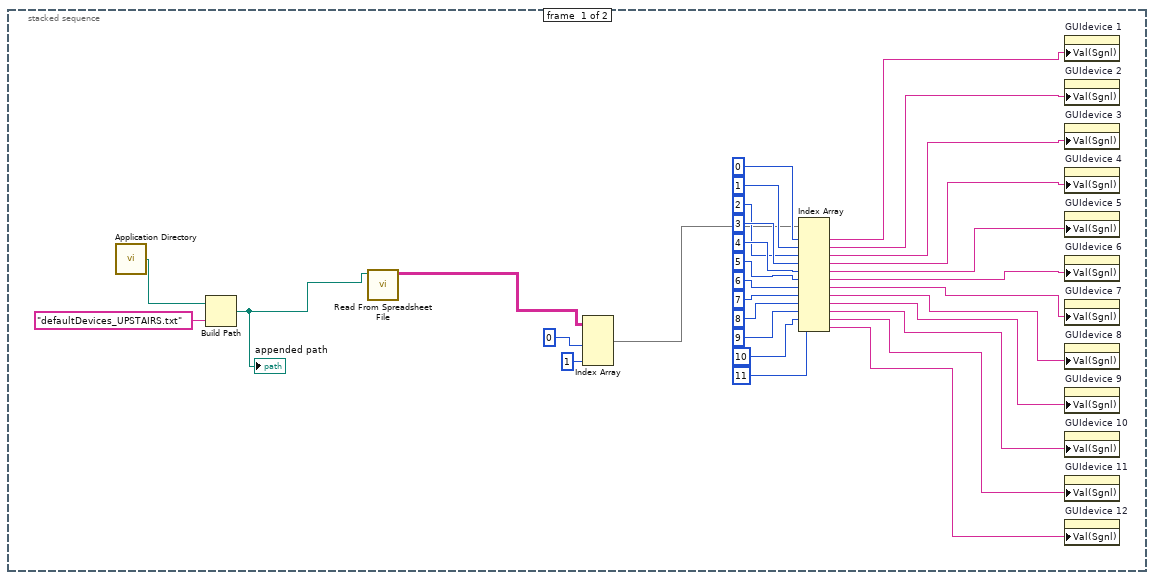
[diagram p2: hidden frame]
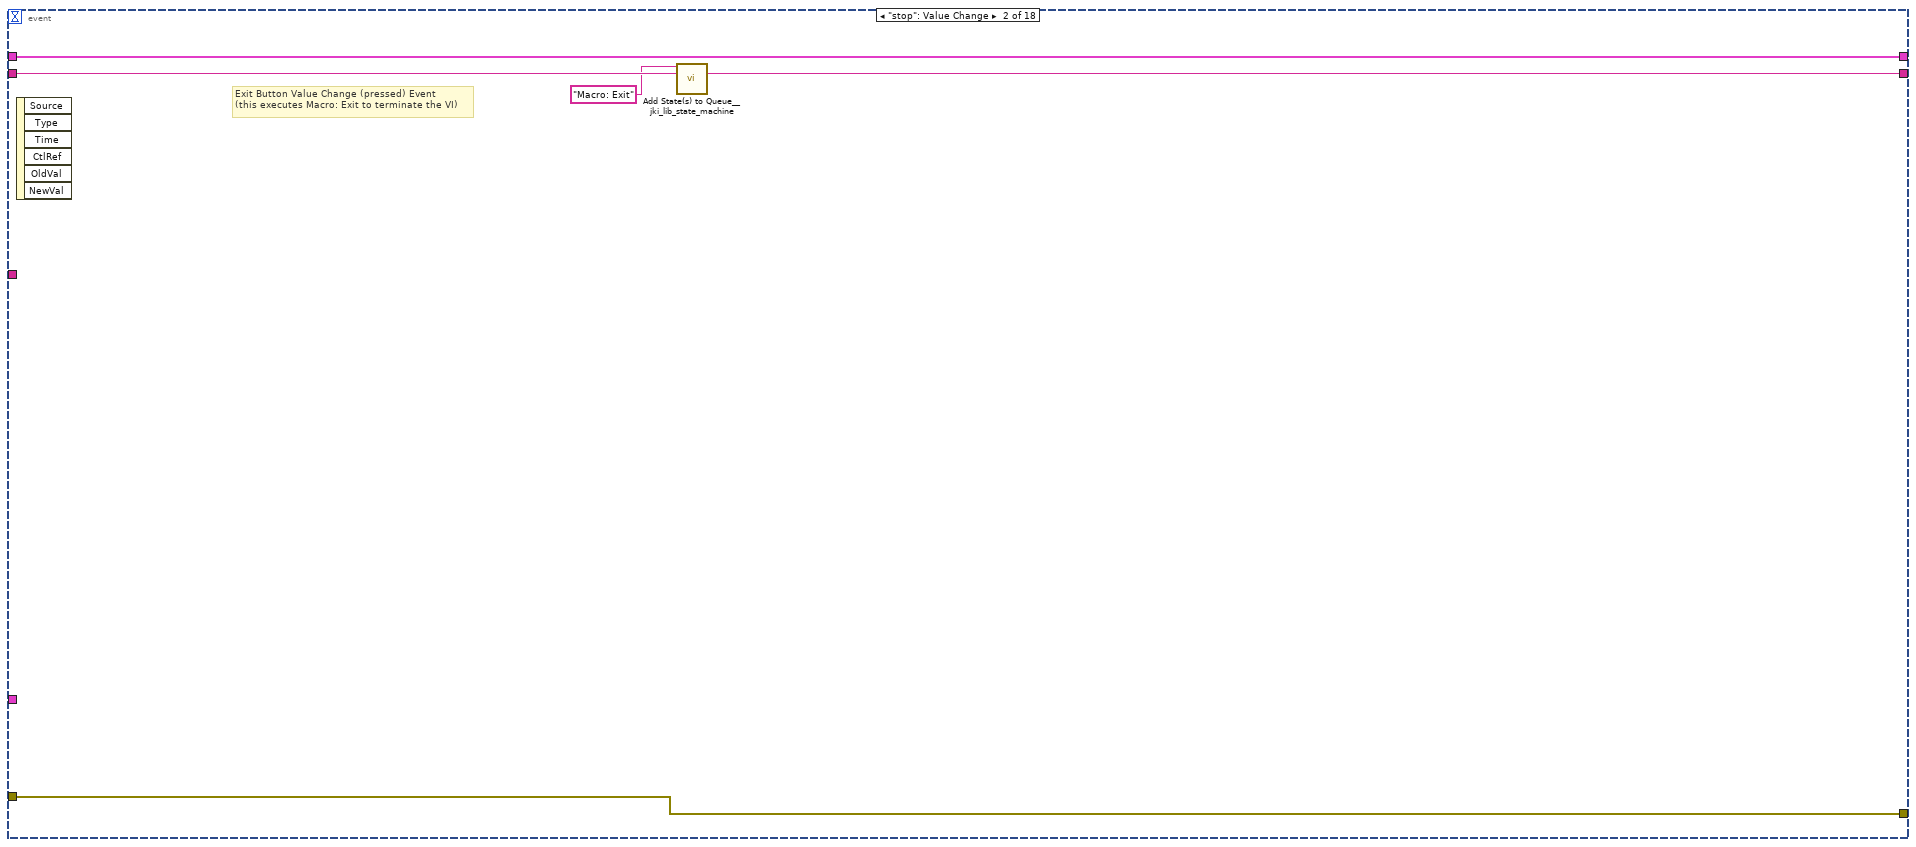
[diagram p7: hidden frame]
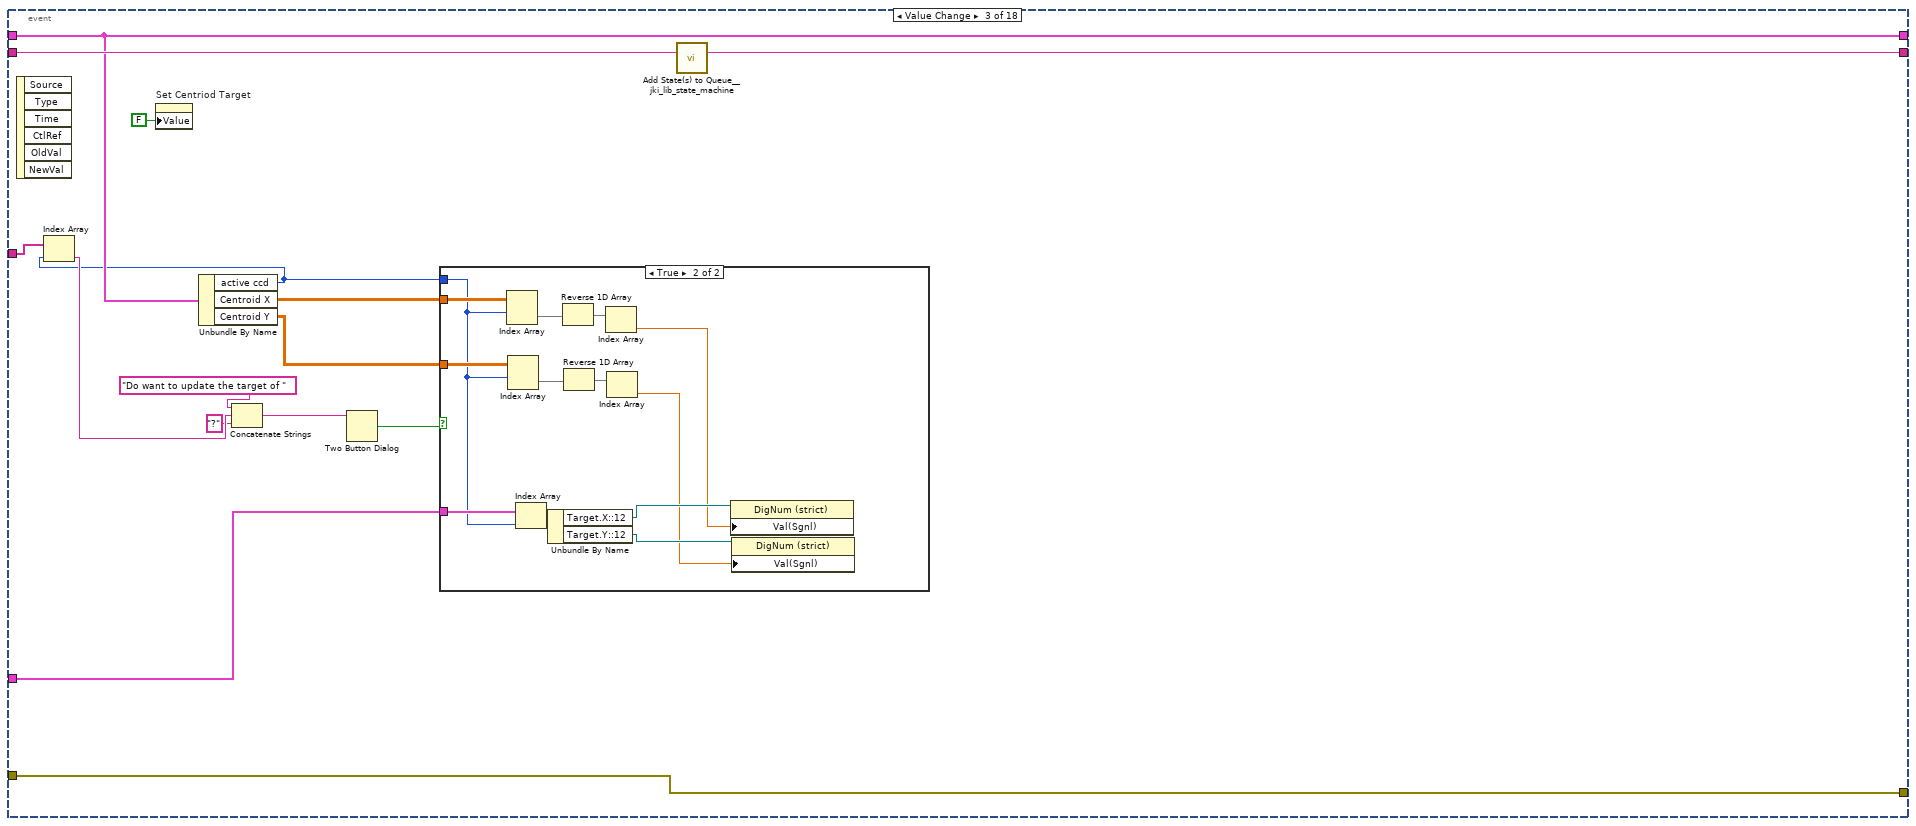
[diagram p8: hidden frame]
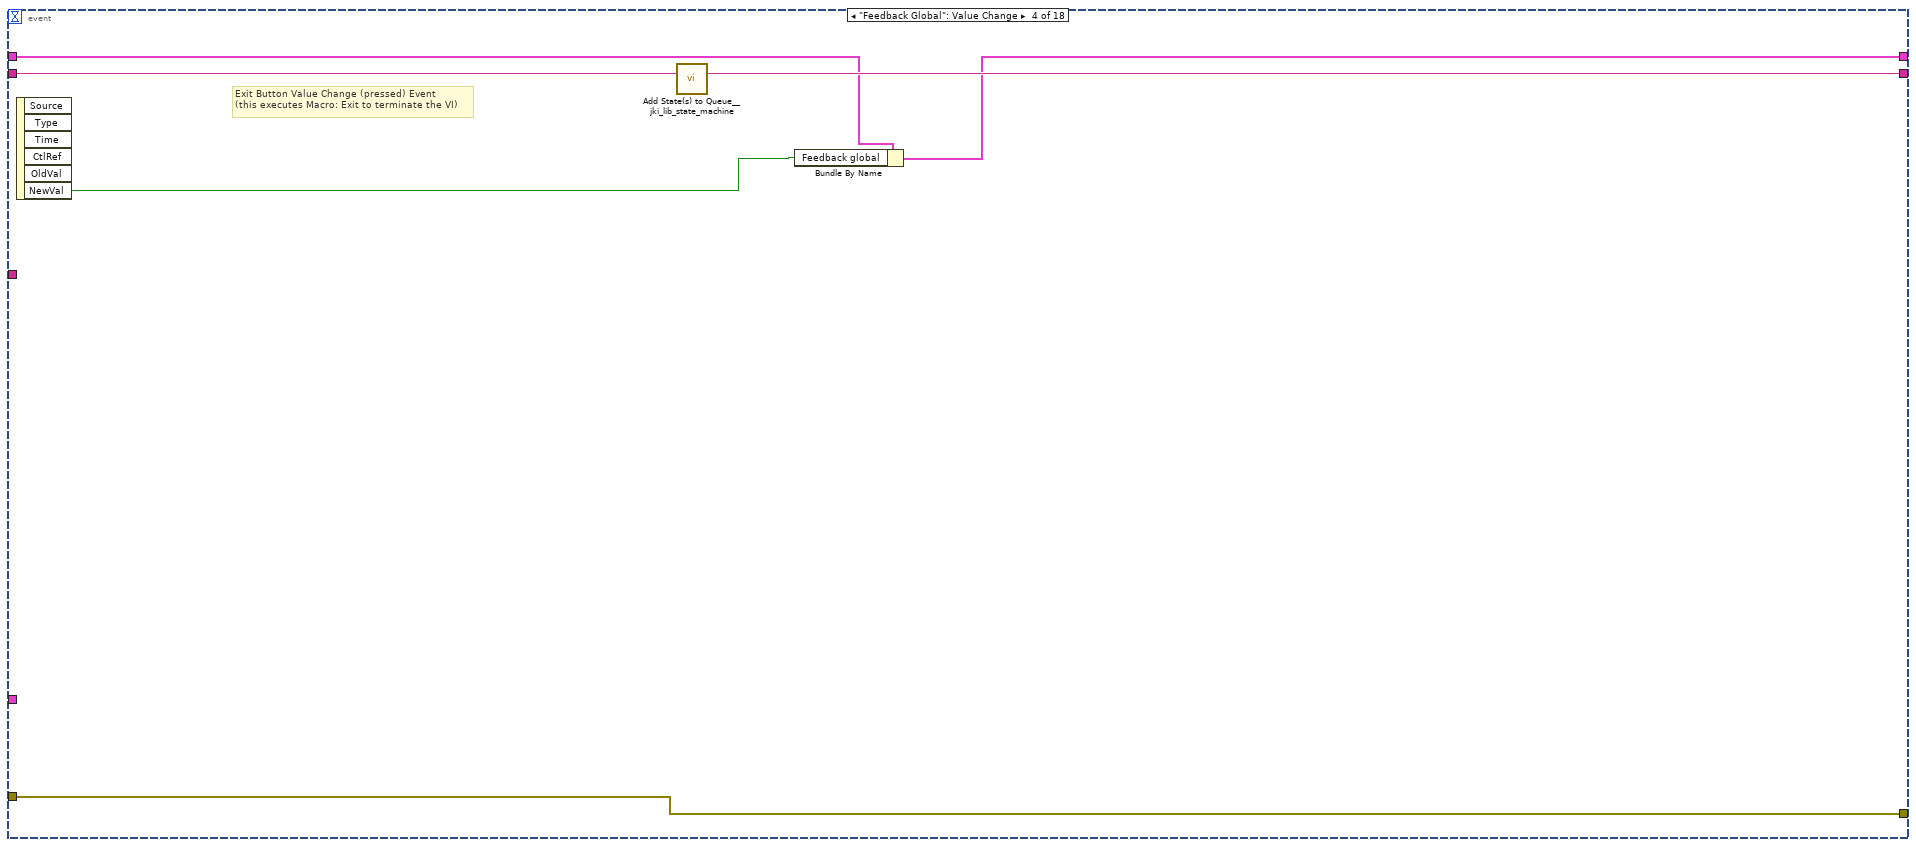
[diagram p10: hidden frame]
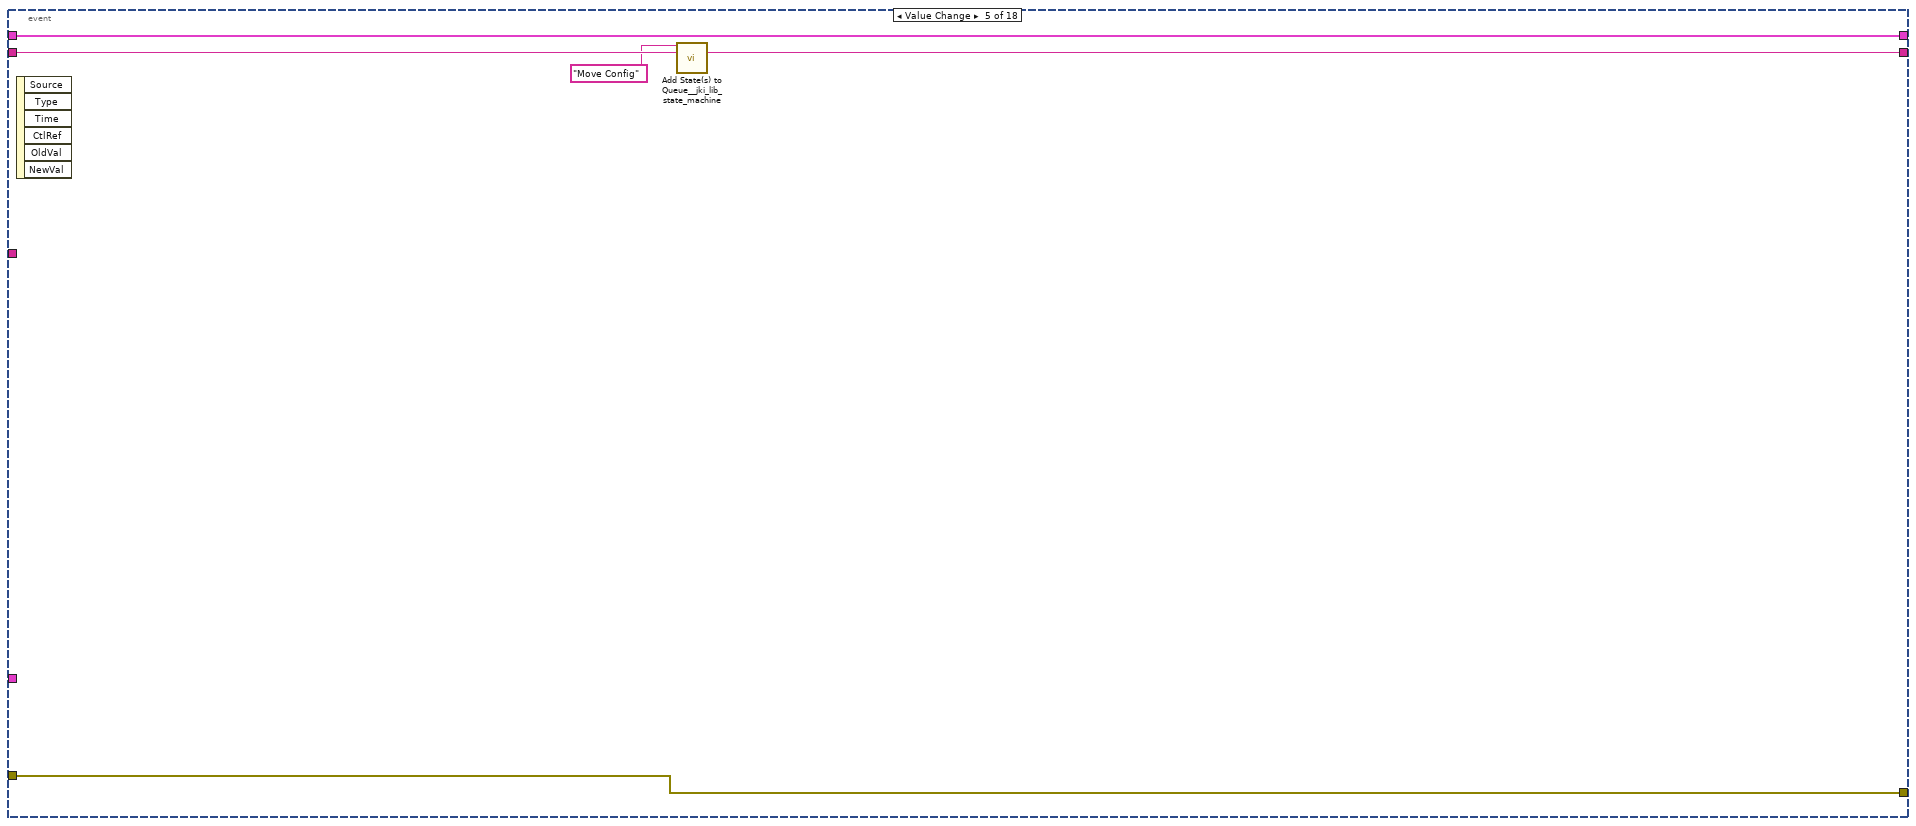
[diagram p11: hidden frame]
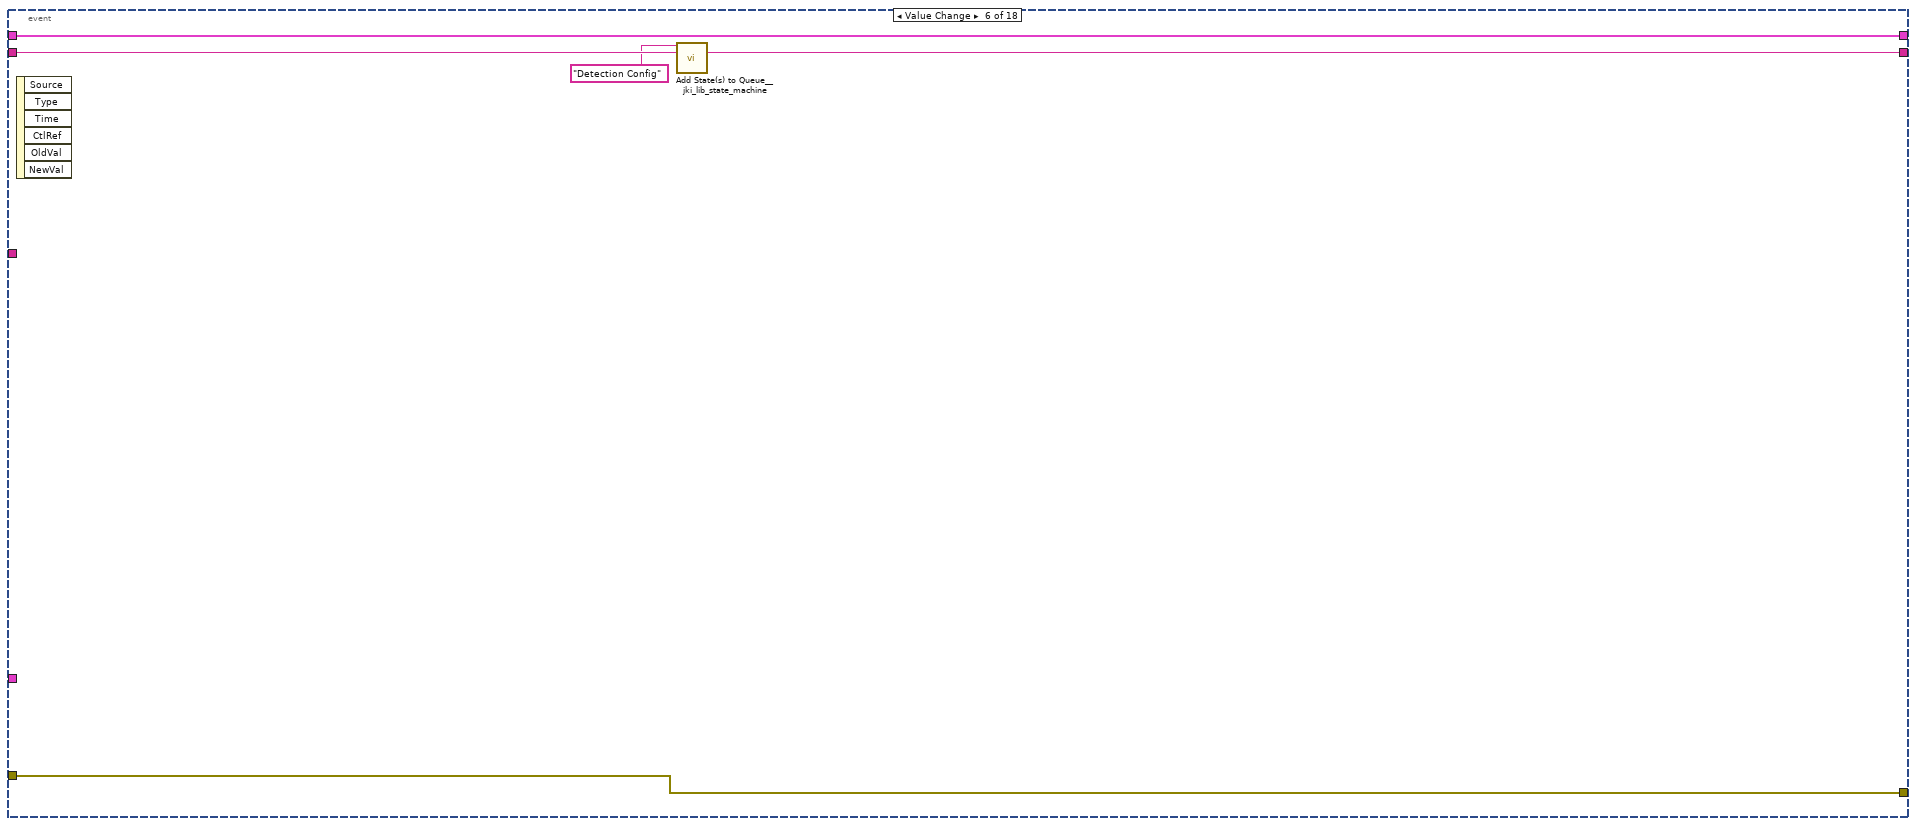
[diagram p12: hidden frame]
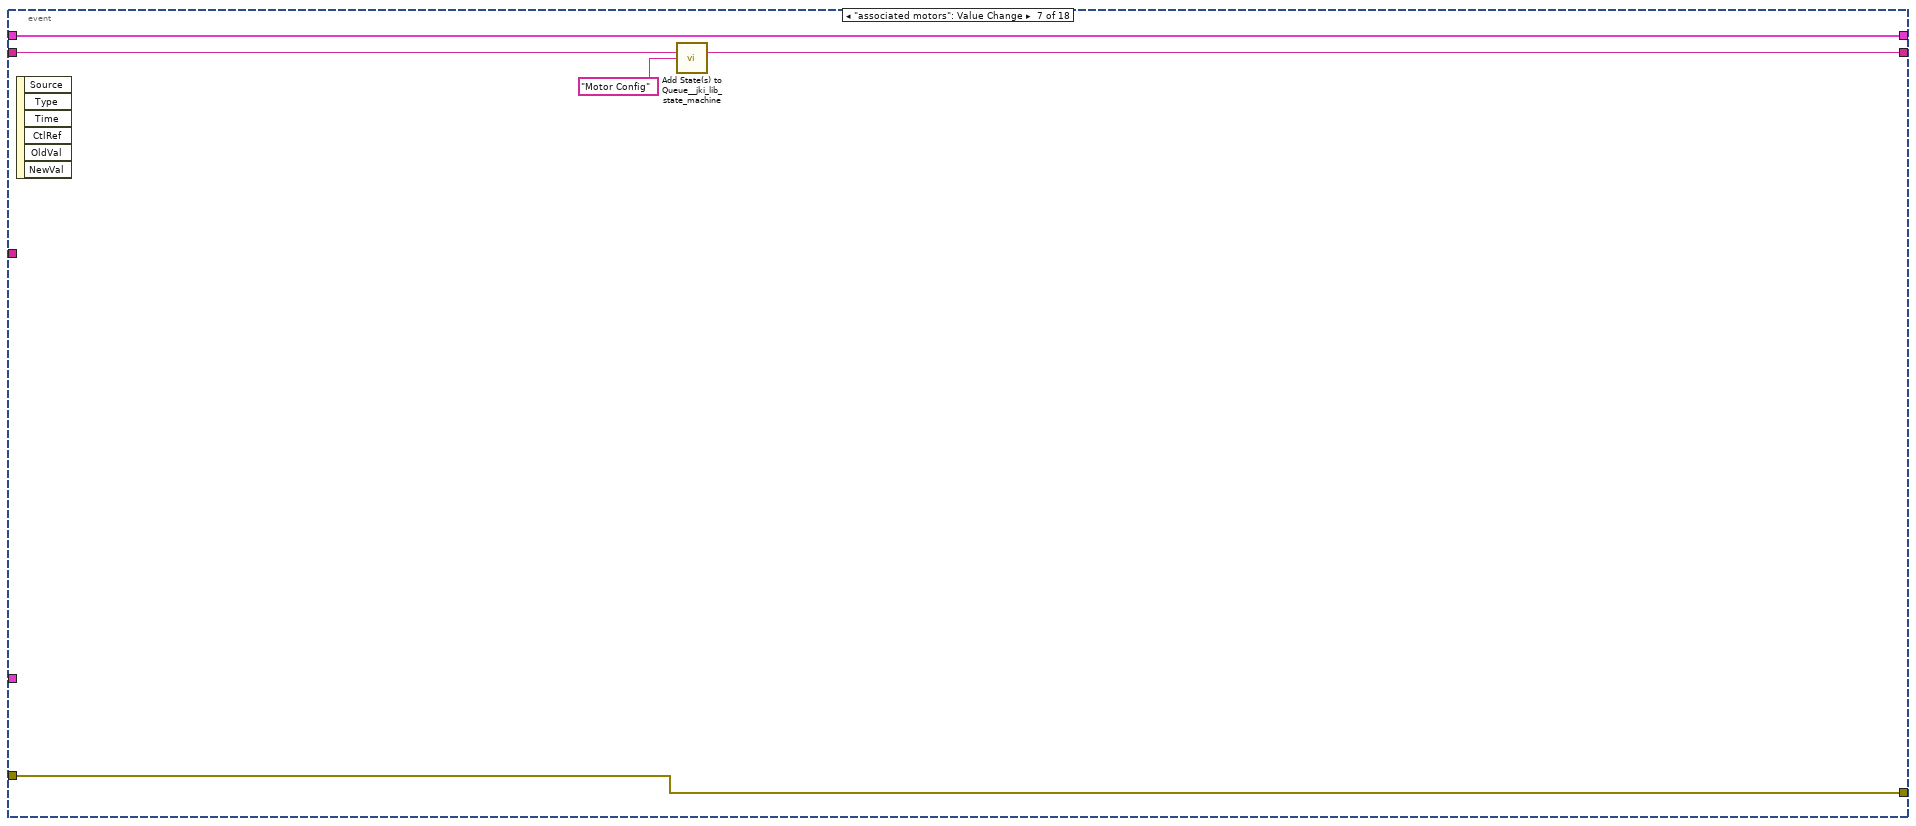
[diagram p13: hidden frame]
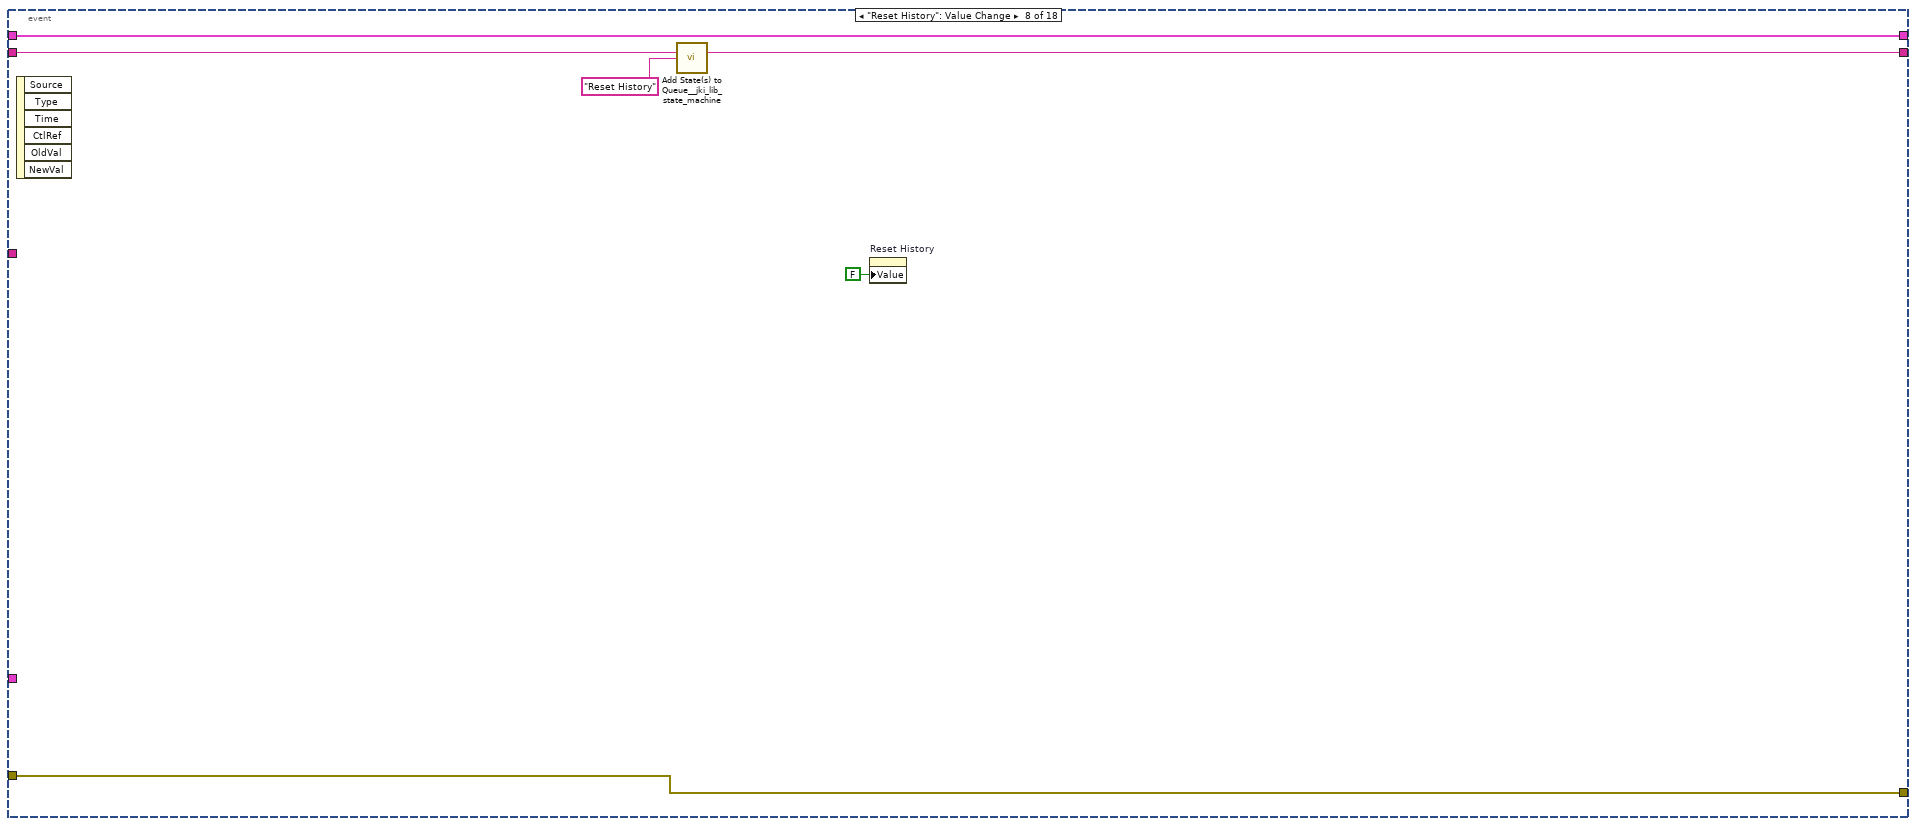
[diagram p14: hidden frame]
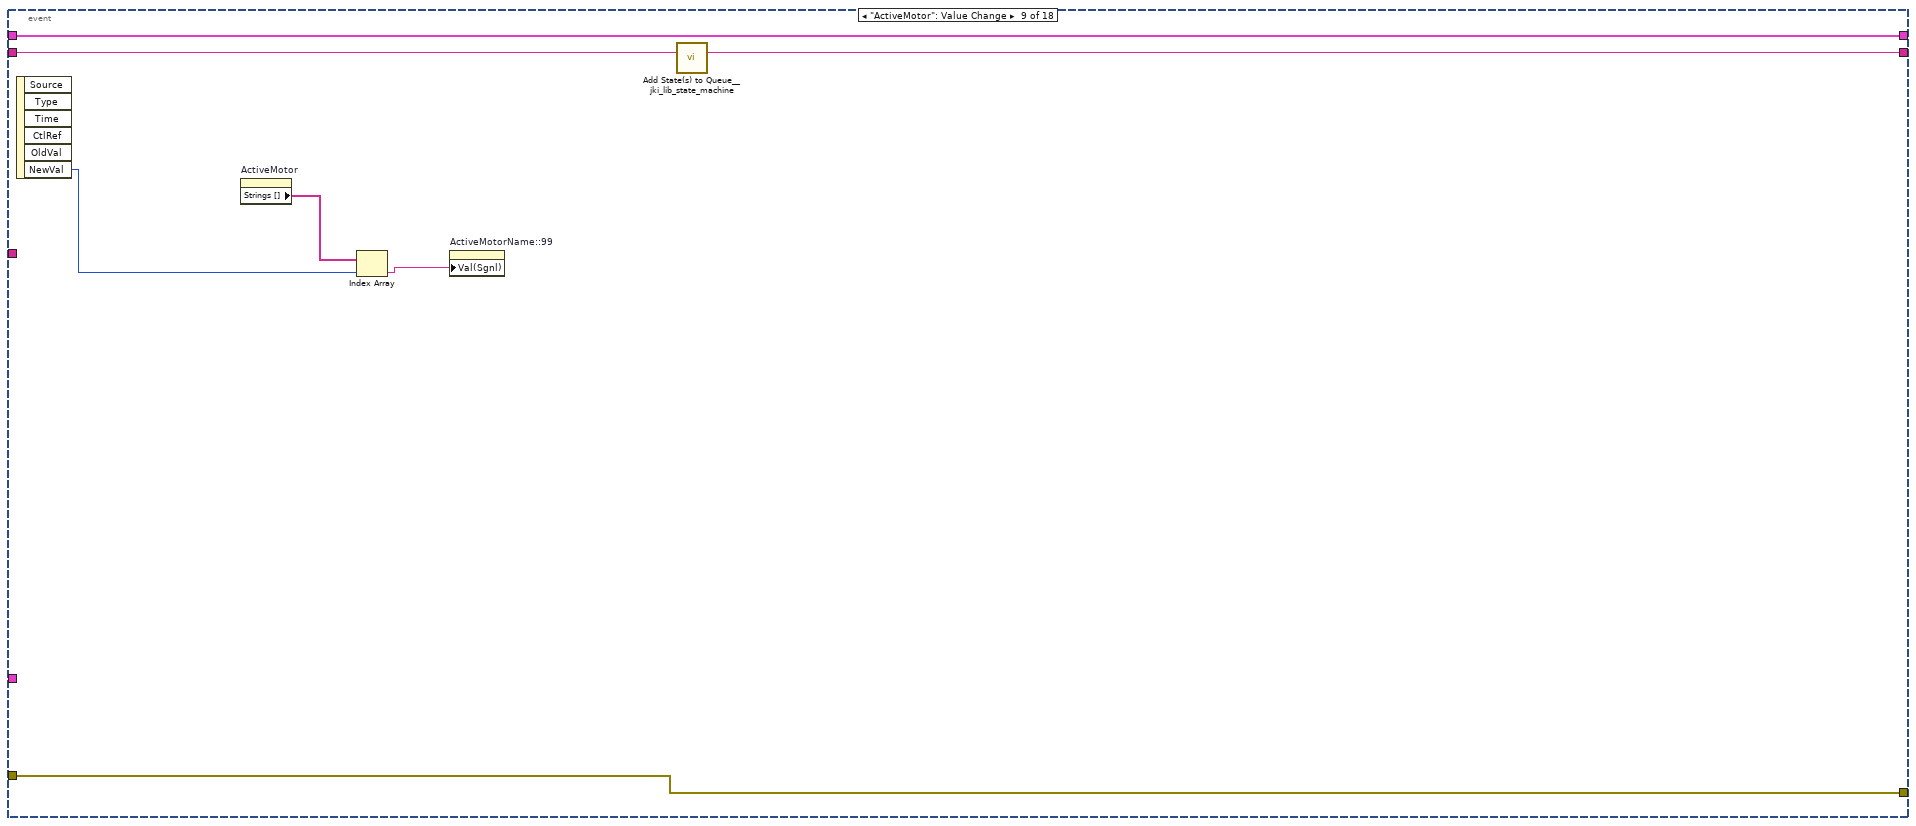
[diagram p15: hidden frame]
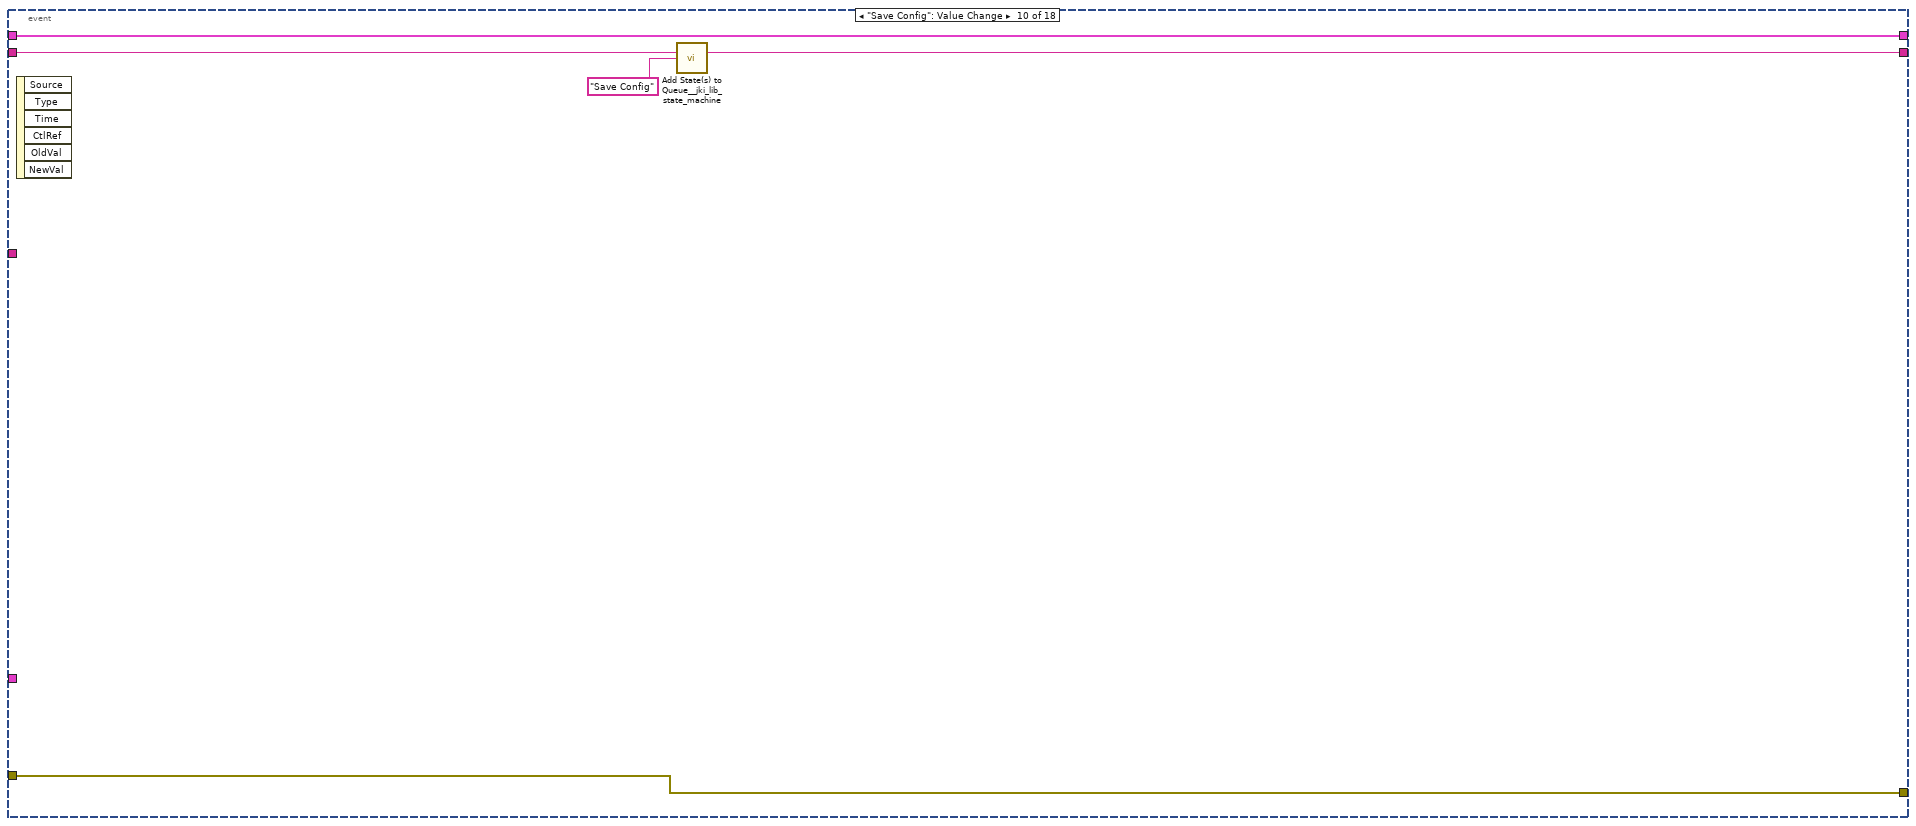
[diagram p16: hidden frame]
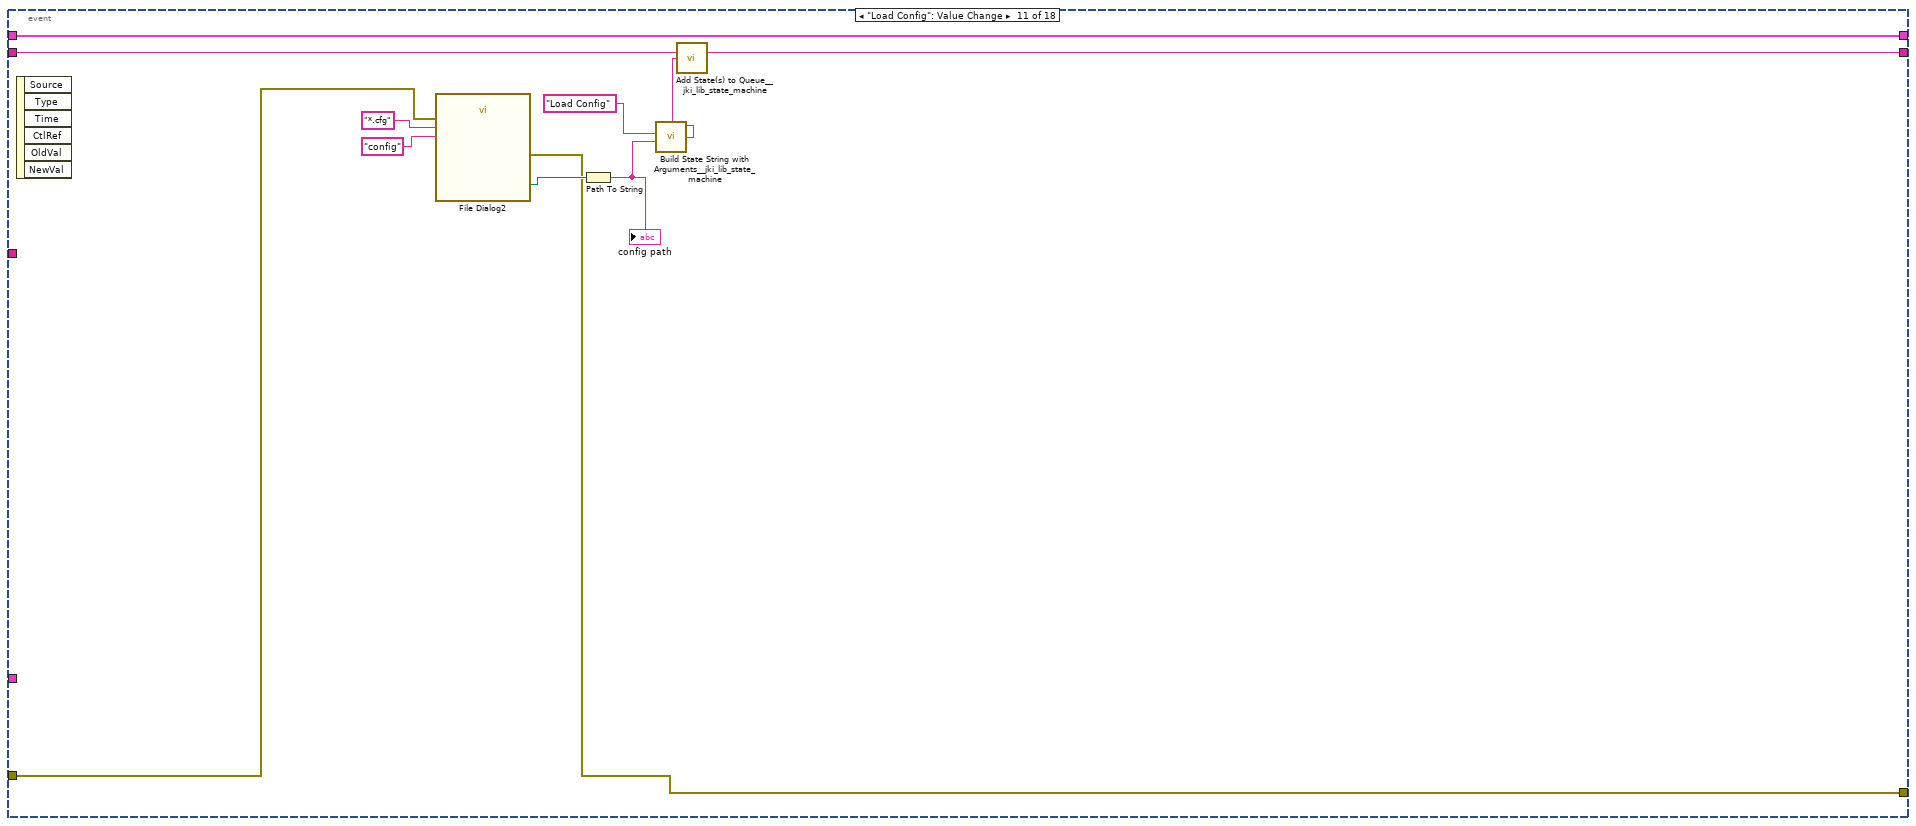
[diagram p17: hidden frame]
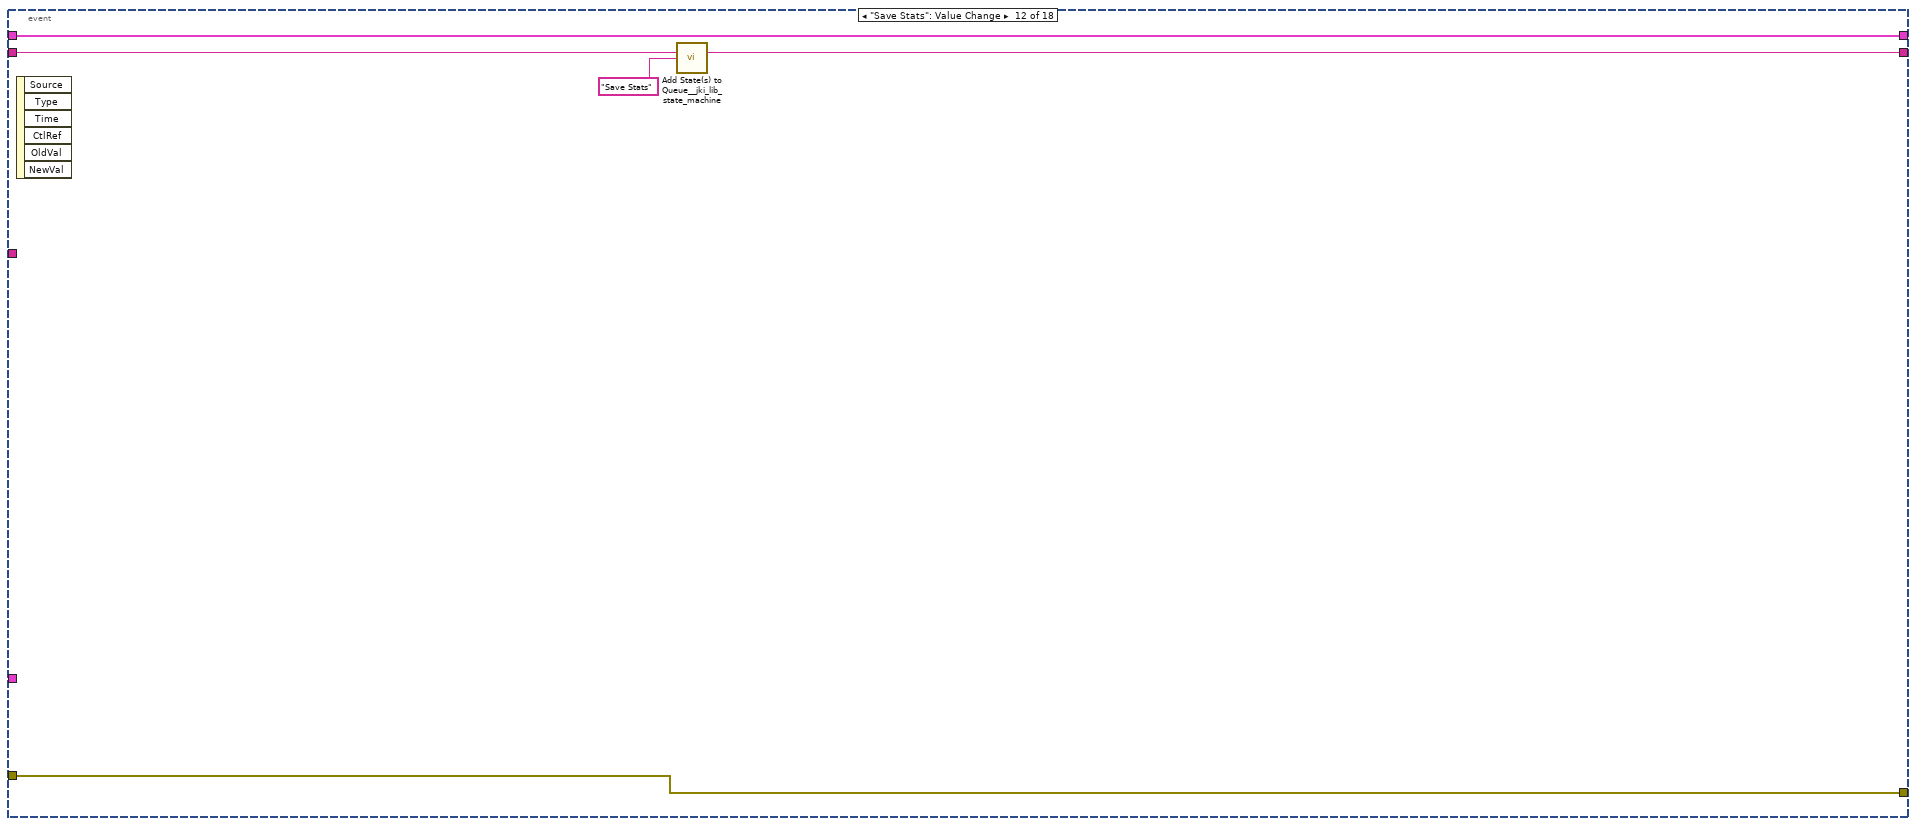
[diagram p18: hidden frame]
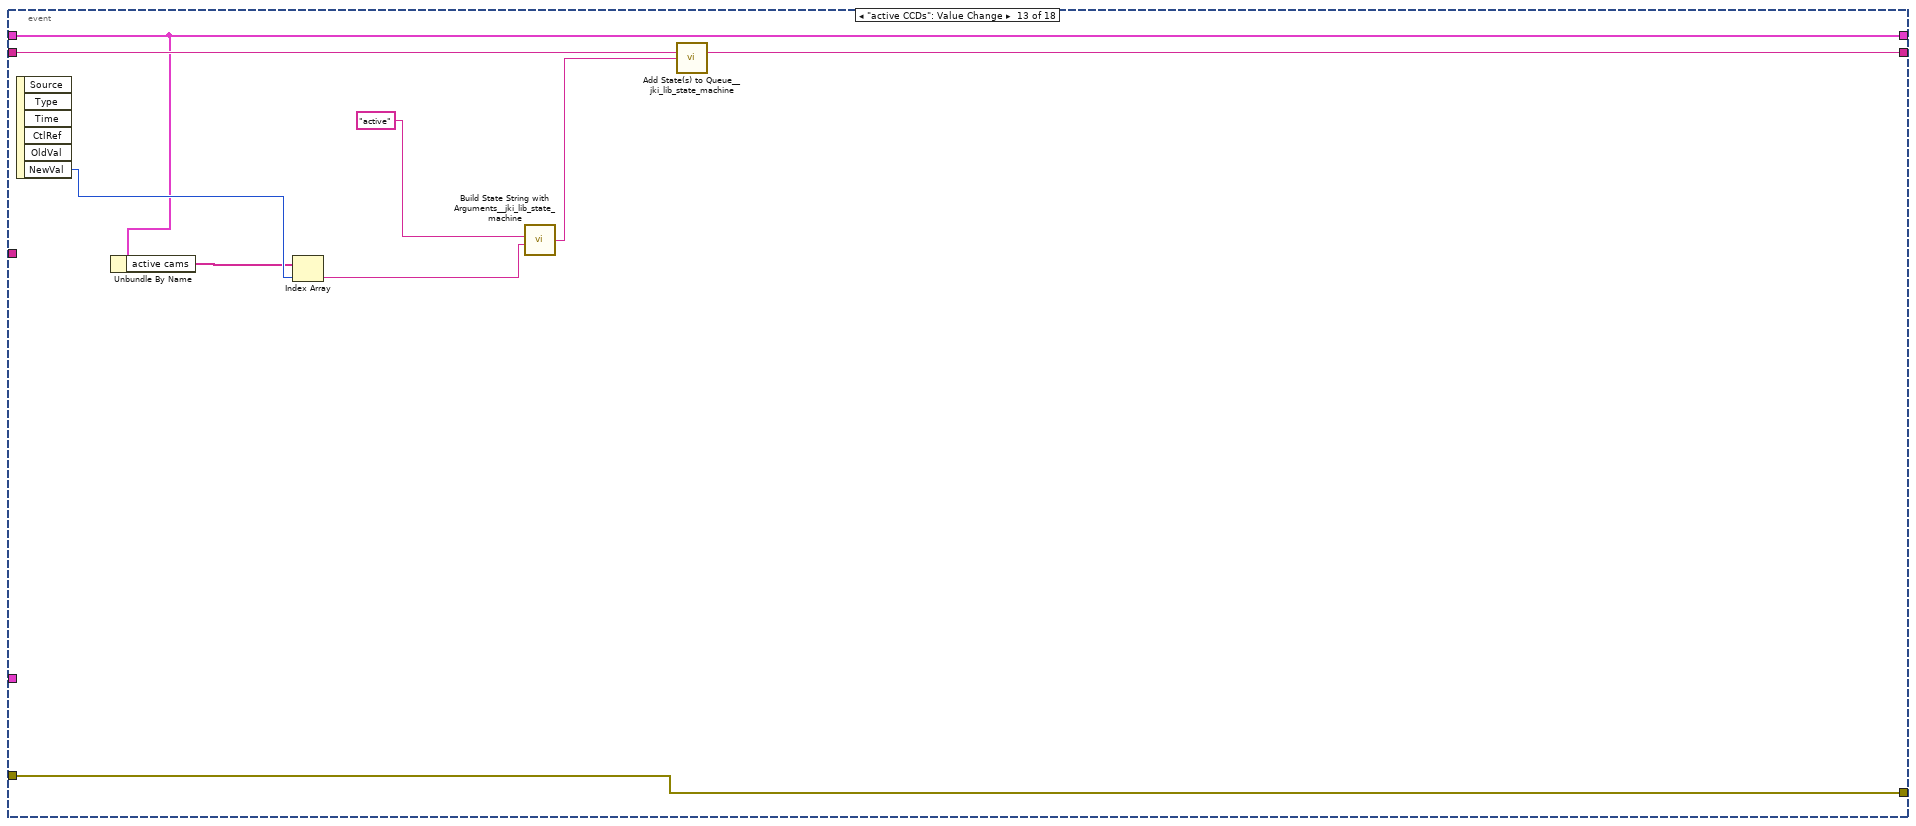
[diagram p19: hidden frame]
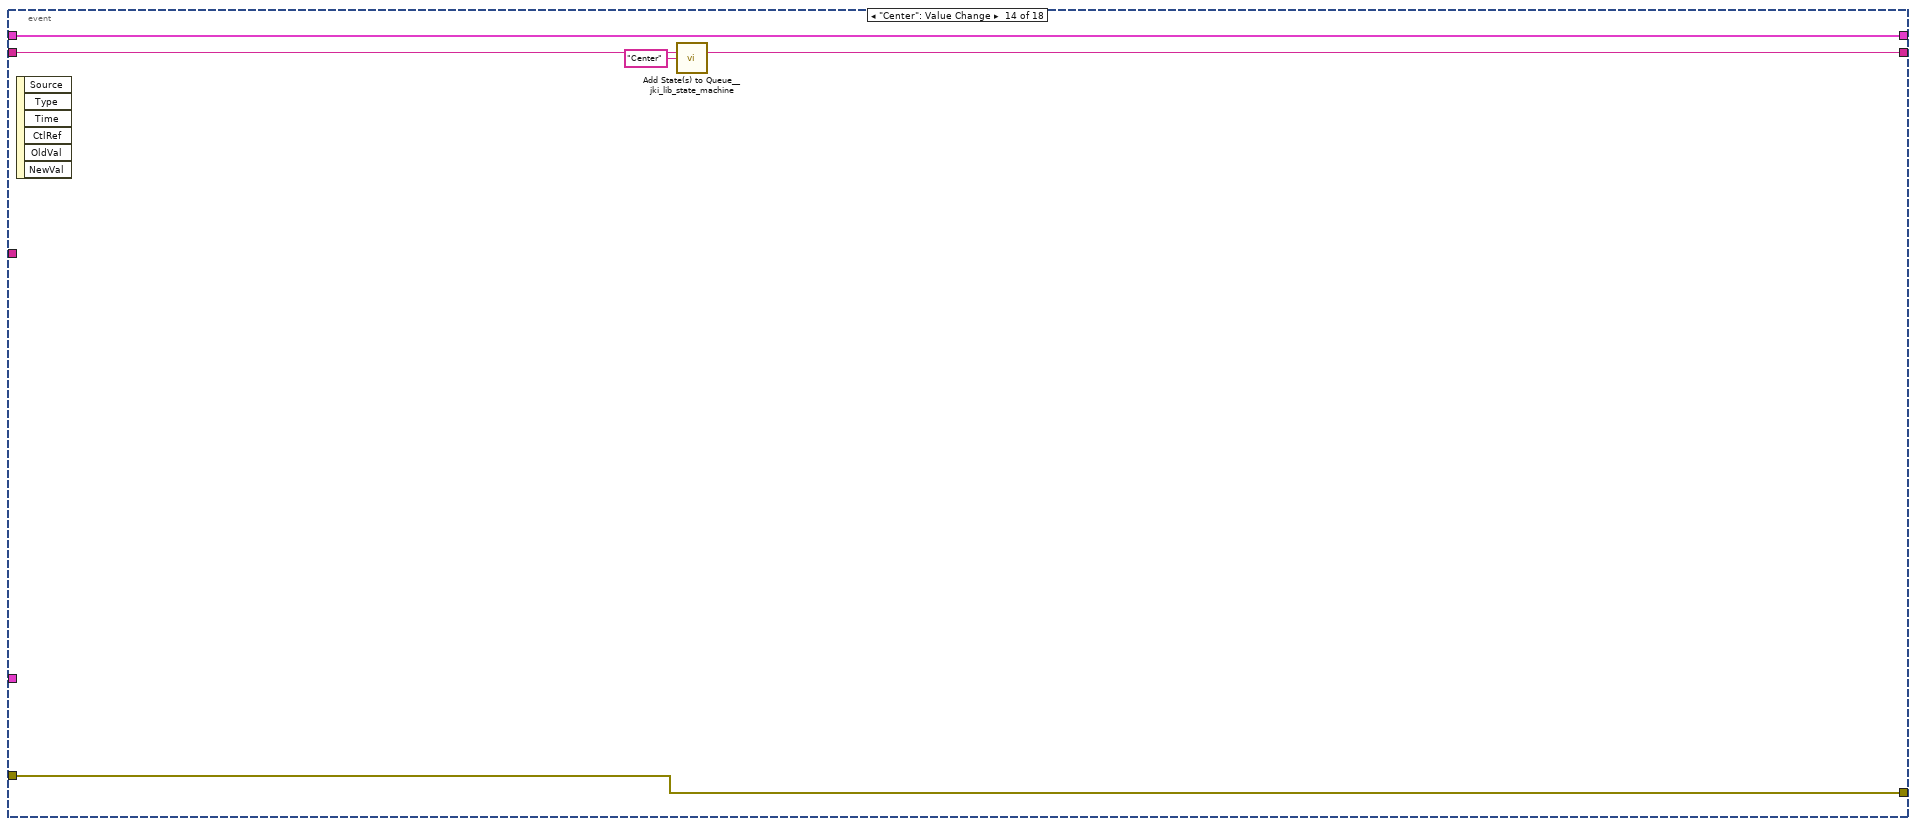
[diagram p20: hidden frame]
diagram:
  n1 = stacked-sequence {
    frame #0 {
      n2 = call <vilib>:"Application Directory.vi"() -> ("Application Directory"=w13:path)
      n3 = Build Path(base path=w13, name or relative path="defaultDevices_UPSTAIRS.txt") -> (appended path=w15:path)
      "appended path" <- w15
      n4 = call-poly <vilib>:"Read From Spreadsheet File.vi"("file path (dialog if empty)"=w15) -> ("all rows"=w16:string[][])  [unwired: 6 in, 4 out]
      n5 = Index Array(array=w16, index (col) #1=0 ("disabled index (col)"), index (col) #2=1 ("index (col)")) -> (element #1=w19:string[])  [unwired: 2 in, 1 out]
      n6 = Index Array(array=w19, index #1=0 ("index"), index #2=1 ("index"), index #3=2 ("index"), index #4=3 ("index"), index #5=4 ("index"), index #6=5 ("index"), index #7=6 ("index"), index #8=7 ("index"), index #9=8 ("index"), index #10=9 ("index"), index #11=10 ("index"), index #12=11 ("index")) -> (element #1=w12:string, element #2=w11:string, element #3=w10:string, element #4=w9:string, element #5=w8:string, element #6=w7:string, element #7=w6:string, element #8=w5:string, element #9=w4:string, element #10=w3:string, element #11=w2:string, element #12=w1:string)
      n7 = property on="GUIdevice 1" class="Str"("Val(Sgnl)"=w12) -> ()  [unwired: 2 in, 2 out]
      n8 = property on="GUIdevice 2" class="Str"("Val(Sgnl)"=w11) -> ()  [unwired: 2 in, 2 out]
      n9 = property on="GUIdevice 3" class="Str"("Val(Sgnl)"=w10) -> ()  [unwired: 2 in, 2 out]
      n10 = property on="GUIdevice 4" class="Str"("Val(Sgnl)"=w9) -> ()  [unwired: 2 in, 2 out]
      n11 = property on="GUIdevice 5" class="Str"("Val(Sgnl)"=w8) -> ()  [unwired: 2 in, 2 out]
      n12 = property on="GUIdevice 6" class="Str"("Val(Sgnl)"=w7) -> ()  [unwired: 2 in, 2 out]
      n13 = property on="GUIdevice 7" class="Str"("Val(Sgnl)"=w6) -> ()  [unwired: 2 in, 2 out]
      n14 = property on="GUIdevice 8" class="Str"("Val(Sgnl)"=w5) -> ()  [unwired: 2 in, 2 out]
      n15 = property on="GUIdevice 9" class="Str"("Val(Sgnl)"=w4) -> ()  [unwired: 2 in, 2 out]
      n16 = property on="GUIdevice 10" class="Str"("Val(Sgnl)"=w3) -> ()  [unwired: 2 in, 2 out]
      n17 = property on="GUIdevice 11" class="Str"("Val(Sgnl)"=w2) -> ()  [unwired: 2 in, 2 out]
      n18 = property on="GUIdevice 12" class="Str"("Val(Sgnl)"=w1) -> ()  [unwired: 2 in, 2 out]
    }
    frame #1 {
      w32 = path "w:/BP_upstairs" ("base path")
      w104 = T20 1 items=["Grayscale (U8)", "Grayscale (I16)", "Grayscale (SGL)", "Complex (CSG)", "RGB (U32)", "HSL (U32)", "RGB (U64)", "Grayscale (U16)"] ("Image Type")
      # "NOT FOR YOU MOFO"
      n19 = control-ref of="Position.Axis 111::98"() -> (w41:refnum<vi>)
      n20 = control-ref of="Position.Axis 112::98"() -> (w42:refnum<vi>)
      n21 = control-ref of="Position.Axis 113::98"() -> (w43:refnum<vi>)
      n22 = control-ref of="Position.Axis 121::98"() -> (w44:refnum<vi>)
      n23 = control-ref of="Position.Axis 122::98"() -> (w45:refnum<vi>)
      n24 = control-ref of="Position.Axis 123::98"() -> (w46:refnum<vi>)
      n25 = control-ref of="Position.Axis 131::98"() -> (w47:refnum<vi>)
      n26 = control-ref of="Position.Axis 132::98"() -> (w48:refnum<vi>)
      n27 = control-ref of="Position.Axis 133::98"() -> (w49:refnum<vi>)
      n28 = control-ref of="Position.Axis 141::98"() -> (w50:refnum<vi>)
      n29 = control-ref of="Position.Axis 142::98"() -> (w51:refnum<vi>)
      n30 = control-ref of="Position.Axis 143::98"() -> (w52:refnum<vi>)
      n31 = control-ref of="Position.Axis 211::98"() -> (w53:refnum<vi>)
      n32 = control-ref of="Position.Axis 212::98"() -> (w54:refnum<vi>)
      n33 = control-ref of="Position.Axis 213::98"() -> (w55:refnum<vi>)
      n34 = control-ref of="Position.Axis 221::98"() -> (w56:refnum<vi>)
      n35 = control-ref of="Position.Axis 222::98"() -> (w57:refnum<vi>)
      n36 = control-ref of="Position.Axis 223::98"() -> (w58:refnum<vi>)
      n37 = control-ref of="Position.Axis 231::98"() -> (w59:refnum<vi>)
      n38 = control-ref of="Position.Axis 232::98"() -> (w60:refnum<vi>)
      n39 = control-ref of="Position.Axis 233::98"() -> (w61:refnum<vi>)
      n40 = control-ref of="Position.Axis 241::98"() -> (w62:refnum<vi>)
      n41 = control-ref of="Position.Axis 242::98"() -> (w63:refnum<vi>)
      n42 = control-ref of="Position.Axis 243::98"() -> (w64:refnum<vi>)
      n43 = control-ref of="Position.Axis 311::98"() -> (w65:refnum<vi>)
      n44 = control-ref of="Position.Axis 312::98"() -> (w66:refnum<vi>)
      n45 = control-ref of="Position.Axis 313::98"() -> (w67:refnum<vi>)
      n46 = control-ref of="Position.Axis 321::98"() -> (w68:refnum<vi>)
      n47 = control-ref of="Position.Axis 322::98"() -> (w69:refnum<vi>)
      n48 = control-ref of="Position.Axis 323::98"() -> (w70:refnum<vi>)
      n49 = control-ref of="Position.Axis 331::98"() -> (w71:refnum<vi>)
      n50 = control-ref of="Position.Axis 332::98"() -> (w72:refnum<vi>)
      n51 = control-ref of="Position.Axis 333::98"() -> (w73:refnum<vi>)
      n52 = control-ref of="Position.Axis 341::98"() -> (w74:refnum<vi>)
      n53 = control-ref of="Position.Axis 342::98"() -> (w75:refnum<vi>)
      n54 = control-ref of="Position.Axis 343::98"() -> (w76:refnum<vi>)
      n55 = control-ref of="Position.Axis 411::98"() -> (w77:refnum<vi>)
      n56 = control-ref of="Position.Axis 412::98"() -> (w78:refnum<vi>)
      n57 = control-ref of="Position.Axis 413::98"() -> (w79:refnum<vi>)
      n58 = control-ref of="Position.Axis 421::98"() -> (w80:refnum<vi>)
      n59 = control-ref of="Position.Axis 422::98"() -> (w81:refnum<vi>)
      n60 = control-ref of="Position.Axis 423::98"() -> (w82:refnum<vi>)
      n61 = control-ref of="Position.Axis 431::98"() -> (w83:refnum<vi>)
      n62 = control-ref of="Position.Axis 432::98"() -> (w84:refnum<vi>)
      n63 = control-ref of="Position.Axis 433::98"() -> (w85:refnum<vi>)
      n64 = control-ref of="Position.Axis 441::98"() -> (w86:refnum<vi>)
      n65 = control-ref of="Position.Axis 442::98"() -> (w87:refnum<vi>)
      n66 = control-ref of="Position.Axis 443::98"() -> (w88:refnum<vi>)
      n67 = control-ref of="Position.Axis 511::98"() -> (w89:refnum<vi>)
      n68 = control-ref of="Position.Axis 512::98"() -> (w90:refnum<vi>)
      n69 = control-ref of="Position.Axis 513::98"() -> (w91:refnum<vi>)
      n70 = control-ref of="Position.Axis 521::98"() -> (w92:refnum<vi>)
      n71 = control-ref of="Position.Axis 522::98"() -> (w93:refnum<vi>)
      n72 = control-ref of="Position.Axis 523::98"() -> (w94:refnum<vi>)
      n73 = control-ref of="Position.Axis 531::98"() -> (w95:refnum<vi>)
      n74 = control-ref of="Position.Axis 532::98"() -> (w96:refnum<vi>)
      n75 = control-ref of="Position.Axis 533::98"() -> (w97:refnum<vi>)
      n76 = control-ref of="Position.Axis 541::98"() -> (w98:refnum<vi>)
      n77 = control-ref of="Position.Axis 542::98"() -> (w99:refnum<vi>)
      n78 = control-ref of="Position.Axis 543::98"() -> (w100:refnum<vi>)
      n79 = control-ref of="Position.Axis 111::99"() -> (w232:refnum<vi>)
      n80 = control-ref of="Position.Axis 112::99"() -> (w231:refnum<vi>)
      n81 = control-ref of="Position.Axis 113::99"() -> (w230:refnum<vi>)
      n82 = control-ref of="Position.Axis 121::99"() -> (w229:refnum<vi>)
      n83 = control-ref of="Position.Axis 122::99"() -> (w228:refnum<vi>)
      n84 = control-ref of="Position.Axis 123::99"() -> (w227:refnum<vi>)
      n85 = control-ref of="Position.Axis 131::99"() -> (w226:refnum<vi>)
      n86 = control-ref of="Position.Axis 132::99"() -> (w225:refnum<vi>)
      n87 = control-ref of="Position.Axis 133::99"() -> (w224:refnum<vi>)
      n88 = control-ref of="Position.Axis 141::99"() -> (w223:refnum<vi>)
      n89 = control-ref of="Position.Axis 142::99"() -> (w222:refnum<vi>)
      n90 = control-ref of="Position.Axis 143::99"() -> (w221:refnum<vi>)
      n91 = control-ref of="Position.Axis 211::99"() -> (w220:refnum<vi>)
      n92 = control-ref of="Position.Axis 212::99"() -> (w219:refnum<vi>)
      n93 = control-ref of="Position.Axis 213::99"() -> (w218:refnum<vi>)
      n94 = control-ref of="Position.Axis 221::99"() -> (w217:refnum<vi>)
      n95 = control-ref of="Position.Axis 222::99"() -> (w216:refnum<vi>)
      n96 = control-ref of="Position.Axis 223::99"() -> (w215:refnum<vi>)
      n97 = control-ref of="Position.Axis 231::99"() -> (w214:refnum<vi>)
      n98 = control-ref of="Position.Axis 232::99"() -> (w213:refnum<vi>)
      n99 = control-ref of="Position.Axis 233::99"() -> (w212:refnum<vi>)
      n100 = control-ref of="Position.Axis 241::99"() -> (w211:refnum<vi>)
      n101 = control-ref of="Position.Axis 242::99"() -> (w210:refnum<vi>)
      n102 = control-ref of="Position.Axis 243::99"() -> (w209:refnum<vi>)
      n103 = control-ref of="Position.Axis 311::99"() -> (w208:refnum<vi>)
      n104 = control-ref of="Position.Axis 312::99"() -> (w207:refnum<vi>)
      n105 = control-ref of="Position.Axis 313::99"() -> (w206:refnum<vi>)
      n106 = control-ref of="Position.Axis 321::99"() -> (w205:refnum<vi>)
      n107 = control-ref of="Position.Axis 322::99"() -> (w204:refnum<vi>)
      n108 = control-ref of="Position.Axis 323::99"() -> (w203:refnum<vi>)
      n109 = control-ref of="Position.Axis 331::99"() -> (w202:refnum<vi>)
      n110 = control-ref of="Position.Axis 332::99"() -> (w201:refnum<vi>)
      n111 = control-ref of="Position.Axis 333::99"() -> (w200:refnum<vi>)
      n112 = control-ref of="Position.Axis 341::99"() -> (w199:refnum<vi>)
      n113 = control-ref of="Position.Axis 342::99"() -> (w198:refnum<vi>)
      n114 = control-ref of="Position.Axis 343::99"() -> (w197:refnum<vi>)
      n115 = control-ref of="Position.Axis 411::99"() -> (w196:refnum<vi>)
      n116 = control-ref of="Position.Axis 412::99"() -> (w195:refnum<vi>)
      n117 = control-ref of="Position.Axis 413::99"() -> (w194:refnum<vi>)
      n118 = control-ref of="Position.Axis 421::99"() -> (w193:refnum<vi>)
      n119 = control-ref of="Position.Axis 422::99"() -> (w192:refnum<vi>)
      n120 = control-ref of="Position.Axis 423::99"() -> (w191:refnum<vi>)
      n121 = control-ref of="Position.Axis 431::99"() -> (w190:refnum<vi>)
      n122 = control-ref of="Position.Axis 432::99"() -> (w189:refnum<vi>)
      n123 = control-ref of="Position.Axis 433::99"() -> (w188:refnum<vi>)
      n124 = control-ref of="Position.Axis 441::99"() -> (w187:refnum<vi>)
      n125 = control-ref of="Position.Axis 442::99"() -> (w186:refnum<vi>)
      n126 = control-ref of="Position.Axis 443::99"() -> (w185:refnum<vi>)
      n127 = control-ref of="Position.Axis 511::99"() -> (w184:refnum<vi>)
      n128 = control-ref of="Position.Axis 512::99"() -> (w183:refnum<vi>)
      n129 = control-ref of="Position.Axis 513::99"() -> (w182:refnum<vi>)
      n130 = control-ref of="Position.Axis 521::99"() -> (w181:refnum<vi>)
      n131 = control-ref of="Position.Axis 522::99"() -> (w180:refnum<vi>)
      n132 = control-ref of="Position.Axis 523::99"() -> (w179:refnum<vi>)
      n133 = control-ref of="Position.Axis 531::99"() -> (w178:refnum<vi>)
      n134 = control-ref of="Position.Axis 532::99"() -> (w177:refnum<vi>)
      n135 = control-ref of="Position.Axis 533::99"() -> (w176:refnum<vi>)
      n136 = control-ref of="Position.Axis 541::99"() -> (w175:refnum<vi>)
      n137 = control-ref of="Position.Axis 542::99"() -> (w174:refnum<vi>)
      n138 = control-ref of="Position.Axis 543::99"() -> (w173:refnum<vi>)
      n139 = Build Array(w41, w42, w43, w44, w45, w46, w47, w48, w49, w50, w51, w52, w53, w54, w55, w56, w57, w58, w59, w60, w61, w62, w63, w64, w65, w66, w67, w68, w69, w70, w71, w72, w73, w74, w75, w76, w77, w78, w79, w80, w81, w82, w83, w84, w85, w86, w87, w88, w89, w90, w91, w92, w93, w94, w95, w96, w97, w98, w99, w100) -> (w38:refnum<vi>[])
      n140 = Build Array(w232, w231, w230, w229, w228, w227, w226, w225, w224, w223, w222, w221, w220, w219, w218, w217, w216, w215, w214, w213, w212, w211, w210, w209, w208, w207, w206, w205, w204, w203, w202, w201, w200, w199, w198, w197, w196, w195, w194, w193, w192, w191, w190, w189, w188, w187, w186, w185, w184, w183, w182, w181, w180, w179, w178, w177, w176, w175, w174, w173) -> (w37:refnum<vi>[])
      n141 = Build Array (concatenate)(w37, w38) -> (→"motor refs":refnum<vi>[])
      n142 = call "getMotorNames.vi"("DeviceName"="GUIdevice 99") -> ("elements"=w35:string[])  [unwired: 10 in]
      n143 = call "getMotorNames.vi"("DeviceName"="GUIdevice 98") -> ("elements"=w34:string[])  [unwired: 10 in]
      n144 = Build Array (concatenate)(w35, w34) -> (w39:string[])
      "Names" <- w39
      n145 = property on="Motor CCD 1" class="Ring (strict)"("Strings []"=w39) -> ()  [unwired: 2 in, 2 out]
      n146 = property on="Motor CCD 2" class="Ring (strict)"("Strings []"=w39) -> ()  [unwired: 2 in, 2 out]
      n147 = property on="Motor CCD 3" class="Ring (strict)"("Strings []"=w39) -> ()  [unwired: 2 in, 2 out]
      n148 = property on="Motor CCD 4" class="Ring (strict)"("Strings []"=w39) -> ()  [unwired: 2 in, 2 out]
      n149 = property on="Motor CCD 5" class="Ring (strict)"("Strings []"=w39) -> ()  [unwired: 2 in, 2 out]
      n150 = property on="Motor CCD 6" class="Ring (strict)"("Strings []"=w39) -> ()  [unwired: 2 in, 2 out]
      n151 = property on="Motor CCD 7" class="Ring (strict)"("Strings []"=w39) -> ()  [unwired: 2 in, 2 out]
      n152 = property on="Motor CCD 8" class="Ring (strict)"("Strings []"=w39) -> ()  [unwired: 2 in, 2 out]
      n153 = property on="Motor CCD 9" class="Ring (strict)"("Strings []"=w39) -> ()  [unwired: 2 in, 2 out]
      n154 = property on="Motor CCD 10" class="Ring (strict)"("Strings []"=w39) -> ()  [unwired: 2 in, 2 out]
      n155 = property on="Motor CCD 11" class="Ring (strict)"("Strings []"=w39) -> ()  [unwired: 2 in, 2 out]
      n156 = property on="Motor CCD 12" class="Ring (strict)"("Strings []"=w39) -> ()  [unwired: 2 in, 2 out]
      n157 = property on="ActiveMotor" class="Ring (strict)"("Strings []"=w35) -> ()  [unwired: 2 in, 2 out]
      n158 = control-ref of="Target.X::1"() -> (w159:refnum<vi>)
      n159 = control-ref of="Target.Y::1"() -> (w158:refnum<vi>)
      n160 = control-ref of="Target.X::2"() -> (w157:refnum<vi>)
      n161 = control-ref of="Target.Y::2"() -> (w156:refnum<vi>)
      n162 = control-ref of="Target.X::3"() -> (w155:refnum<vi>)
      n163 = control-ref of="Target.Y::3"() -> (w154:refnum<vi>)
      n164 = control-ref of="Target.X::4"() -> (w153:refnum<vi>)
      n165 = control-ref of="Target.Y::4"() -> (w152:refnum<vi>)
      n166 = control-ref of="Target.X::5"() -> (w151:refnum<vi>)
      n167 = control-ref of="Target.Y::5"() -> (w150:refnum<vi>)
      n168 = control-ref of="Target.X::6"() -> (w149:refnum<vi>)
      n169 = control-ref of="Target.Y::6"() -> (w148:refnum<vi>)
      n170 = control-ref of="Target.X::7"() -> (w147:refnum<vi>)
      n171 = control-ref of="Target.Y::7"() -> (w146:refnum<vi>)
      n172 = control-ref of="Target.X::8"() -> (w145:refnum<vi>)
      n173 = control-ref of="Target.Y::8"() -> (w144:refnum<vi>)
      n174 = control-ref of="Target.X::9"() -> (w121:refnum<vi>)
      n175 = control-ref of="Target.Y::9"() -> (w120:refnum<vi>)
      n176 = control-ref of="Target.X::10"() -> (w119:refnum<vi>)
      n177 = control-ref of="Target.Y::10"() -> (w118:refnum<vi>)
      n178 = control-ref of="Target.X::11"() -> (w117:refnum<vi>)
      n179 = control-ref of="Target.Y::11"() -> (w116:refnum<vi>)
      n180 = control-ref of="Target.X::12"() -> (w115:refnum<vi>)
      n181 = control-ref of="Target.Y::12"() -> (w114:refnum<vi>)
      n182 = call "IMAQ Create"("Image Name"="GUIdevice 8", "Image Type"=w104) -> ("New Image"=→"image::8":T9)  [unwired: 3 in, 1 out]
      n183 = call "IMAQ Create"("Image Name"="GUIdevice 9", "Image Type"=w104) -> ("New Image"=→"image::9":T9)  [unwired: 3 in, 1 out]
      n184 = call "IMAQ Create"("Image Name"="GUIdevice 10", "Image Type"=w104) -> ("New Image"=→"image::10":T9)  [unwired: 3 in, 1 out]
      n185 = call "IMAQ Create"("Image Name"="GUIdevice 6", "Image Type"=w104) -> ("New Image"=→"image::6":T9)  [unwired: 3 in, 1 out]
      n186 = call "IMAQ Create"("Image Name"="GUIdevice 7", "Image Type"=w104) -> ("New Image"=→"image::7":T9)  [unwired: 3 in, 1 out]
      n187 = call "IMAQ Create"("Image Name"="GUIdevice 11", "Image Type"=w104) -> ("New Image"=→"image::11":T9)  [unwired: 3 in, 1 out]
      n188 = call "IMAQ Create"("Image Name"="GUIdevice 12", "Image Type"=w104) -> ("New Image"=→"image::12":T9)  [unwired: 3 in, 1 out]
      n189 = call "IMAQ Create"("Image Name"="GUIdevice 2") -> ("New Image"=→"image::2":T9)  [unwired: 4 in, 1 out]
      n190 = call "IMAQ Create"("Image Name"="GUIdevice 4", "Image Type"=w104) -> ("New Image"=→"image::4":T9)  [unwired: 3 in, 1 out]
      n191 = call "IMAQ Create"("Image Name"="GUIdevice 1", "Image Type"=w104) -> ("New Image"=→"image::1":T9)  [unwired: 3 in, 1 out]
      n192 = call "IMAQ Create"("Image Name"="GUIdevice 3", "Image Type"=w104) -> ("New Image"=→"image::3":T9)  [unwired: 3 in, 1 out]
      n193 = call "IMAQ Create"("Image Name"="GUIdevice 5", "Image Type"=w104) -> ("New Image"=→"image::5":T9)  [unwired: 3 in, 1 out]
      n194 = Build Array("GUIdevice 1", "GUIdevice 2", "GUIdevice 3", "GUIdevice 4", "GUIdevice 5", "GUIdevice 6", "GUIdevice 7", "GUIdevice 8", "GUIdevice 9", "GUIdevice 10", "GUIdevice 11", "GUIdevice 12") -> (w133:string[])
      "CCDs" <- w133
      n195 = property on="image::8" class="ImageControl"("Caption.Text"="GUIdevice 8") -> ()  [unwired: 2 in, 2 out]
      n196 = property on="image::10" class="ImageControl"("Caption.Text"="GUIdevice 10") -> ()  [unwired: 2 in, 2 out]
      n197 = property on="image::9" class="ImageControl"("Caption.Text"="GUIdevice 9") -> ()  [unwired: 2 in, 2 out]
      n198 = property on="image::1" class="ImageControl"("Caption.Text"="GUIdevice 1") -> ()  [unwired: 2 in, 2 out]
      n199 = property on="image::2" class="ImageControl"("Caption.Text"="GUIdevice 2") -> ()  [unwired: 2 in, 2 out]
      n200 = property on="image::3" class="ImageControl"("Caption.Text"="GUIdevice 3") -> ()  [unwired: 2 in, 2 out]
      n201 = property on="image::4" class="ImageControl"("Caption.Text"="GUIdevice 4") -> ()  [unwired: 2 in, 2 out]
      n202 = property on="image::5" class="ImageControl"("Caption.Text"="GUIdevice 5") -> ()  [unwired: 2 in, 2 out]
      n203 = property on="image::6" class="ImageControl"("Caption.Text"="GUIdevice 6") -> ()  [unwired: 2 in, 2 out]
      n204 = property on="image::7" class="ImageControl"("Caption.Text"="GUIdevice 7") -> ()  [unwired: 2 in, 2 out]
      n205 = property on="image::11" class="ImageControl"("Caption.Text"="GUIdevice 11") -> ()  [unwired: 2 in, 2 out]
      n206 = property on="image::12" class="ImageControl"("Caption.Text"="GUIdevice 12") -> ()  [unwired: 2 in, 2 out]
      n207 = Array To Cluster(array=w133) -> (cluster=→"Cameras":T21)
      n208 = Bundle("Target.X::1"=w159, "Target.Y::1"=w158) -> (w143:T22)  [unwired: 1 in]
      n209 = Bundle("Target.X::2"=w157, "Target.Y::2"=w156) -> (w142:T23)  [unwired: 1 in]
      n210 = Bundle("Target.X::3"=w155, "Target.Y::3"=w154) -> (w141:T24)  [unwired: 1 in]
      n211 = Bundle("Target.X::4"=w153, "Target.Y::4"=w152) -> (w134:T25)  [unwired: 1 in]
      n212 = Bundle("Target.X::5"=w151, "Target.Y::5"=w150) -> (w140:T26)  [unwired: 1 in]
      n213 = Bundle("Target.X::6"=w149, "Target.Y::6"=w148) -> (w139:T27)  [unwired: 1 in]
      n214 = Bundle("Target.X::7"=w147, "Target.Y::7"=w146) -> (w138:T28)  [unwired: 1 in]
      n215 = Bundle("Target.X::8"=w145, "Target.Y::8"=w144) -> (w137:T29)  [unwired: 1 in]
      n216 = Bundle("Target.X::12"=w115, "Target.Y::12"=w114) -> (w110:T30)  [unwired: 1 in]
      n217 = Bundle("Target.X::9"=w121, "Target.Y::9"=w120) -> (w113:T31)  [unwired: 1 in]
      n218 = Bundle("Target.X::10"=w119, "Target.Y::10"=w118) -> (w112:T32)  [unwired: 1 in]
      n219 = Bundle("Target.X::11"=w117, "Target.Y::11"=w116) -> (w111:T33)  [unwired: 1 in]
      n220 = property on="CCDs" class="Ring (strict)"("Strings []"=w133) -> ()  [unwired: 2 in, 2 out]
      n221 = Build Array(w143, w142, w141, w134, w140, w139, w138, w137, w113, w112, w111, w110) -> (w136:T34)
      n222 = Tick Count (ms)() -> (millisecond timer value=→"millisecond timer value":u32)
      n223 = property on="Feedback Global" class="Bool (strict)"("Value"=FALSE ("Feedback Global")) -> ()  [unwired: 2 in, 2 out]
      n224 = Get Date/Time In Seconds() -> (seconds since 1Jan1904=w123:timestamp)
      n225 = Format Date/Time String(time format string (%c)="%Y%m%d%H%M", seconds (now)=w123) -> (date/time string=w122:string)  [unwired: 1 in]
      n226 = Concatenate Strings(w122, "Beampointing_Pico.tdms" ("string")) -> (w126:string)
      n227 = String To Path(string=w126) -> (path=w125:path)
      n228 = Build Path(base path=w32, name or relative path=w125) -> (appended path=w128:path)
      n229 = call <vilib>:"Add State(s) to Queue__jki_lib_state_machine.vi"("State(s) in (\"\")"="Macro: Initialize") -> ("States Out"=w234:string)  [unwired: 14 in]
      n230 = Create User Event(user event datatype=T14 {"EventEnum"=enum."new data", "Device name"="Device name"} ("New Event")) -> (user event=w242:refnum<user-event>, error out=w244:errorcluster)  [unwired: 1 in]
      "tcp data event" <- w242
      n231 = while "JKI - String-Based Queued State Machine (Basic) v1.0" {
        shift-right: [w267] -> w132
        shift-left: _ -> [w255]
        shift-right: [w270] -> w160
        shift-left: _ -> [w266]
        shift-right: [w269] -> _
        shift-left: w234 -> [w271]
        tunnel: w136 -> [w264]
        tunnel: w133 -> [w262]
        tunnel: [w262] -> w161
        tunnel: w136 -> [w263]
        tunnel: w128 -> [w253]
        tunnel: w32 -> [w252]
        stop <- w268 stop-if-true
        n232 = Unbundle By Name(w255) -> ("active cams"=w254:string[])
        n233 = call <vilib>:"Parse State Queue__jki_lib_state_machine.vi"("State Queue"=w271, "Error In (no error)"=w266) -> ("Remaining States"=w273:string, "Current State"=w274:string, "Arguments"=w272:string)  [unwired: 11 in]
        "Current State" <- w274
        n234 = case shown="\"\", \"Idle\"" w274 {
          selector: w274 -> [_ _ w561 _ _ _ _ _ _ _ _ _ _ _ _ _ _ _ _ _ _ _ _ _ _ _ _ _ _ _ _ _ _ _ _ _ _ _ _ _]
          tunnel: w273 -> [w303 w560 w565 w583 w590 w595 w599 w641 w649 w653 w657 w663 w674 w698 w708 w718 w722 w744 w846 w899 w912 w921 w948 w969 w973 w992 w1131 w1285 w1376 w1442 w1480 w1500 w1515 w1604 w1656 w1666 w1673 w1705 w1731 w1758]
          tunnel: w272 -> [_ _ _ _ _ _ _ _ _ _ _ w658 w669 _ _ _ _ w739 w797 _ w909 _ _ _ _ w994 _ w1263 w1353 _ _ _ _ _ _ _ w1670 _ _ _]
          tunnel: w255 -> [w301 w557 w563 w573 w587 w593 w596 _ w645 w650 w655 w661 w668 w695 w706 w710 w719 w736 w798 w897 w904 w917 w940 w962 w970 w976 w1125 w1278 w1369 w1439 w1451 w1497 w1512 w1578 w1653 w1663 w1669 w1693 w1728 w1749]
          tunnel: [w300 w558 w567 w581 errorcluster {"status"=FALSE, "code"=0, "source"=""} ("error out") w592 w597 w609 w642 w651 w654 w659 w671 w696 w707 w716 w720 w740 w802 w889 w910 w919 w946 w967 w971 w996 w1155 w1283 w1374 w1440 w1478 w1498 w1513 w1563 w1654 w1664 w1671 w1674 w1729 w1756] -> w270
          tunnel: w266 -> [w299 w558 w566 w581 w586 w592 w597 w616 w647 w651 w654 w660 w672 w696 w707 w716 w720 w740 w800 w880 w910 w919 w946 w967 w971 w996 w1155 w1283 w1374 w1440 w1478 w1498 w1513 w1599 w1654 w1664 w1671 w1691 w1729 w1756]
          tunnel: [w302 w559 w564 w582 w589 w594 w598 w640 w648 w652 w656 w662 w673 w697 w699 w717 w721 w730 w845 w898 w911 w920 w947 w968 w972 w999 w1156 w1284 w1375 w1441 w1479 w1499 w1514 w1566 w1655 w1665 w1672 w1704 w1730 w1757] -> w269
          tunnel: [_ _ _ _ _ TRUE _ _ _ _ _ _ _ _ _ _ _ _ _ _ _ _ _ _ _ _ _ _ _ _ _ _ _ _ _ _ _ _ _ _] -> w268
          tunnel: [w296 w557 w563 w572 w587 w593 w596 w601 w645 w650 w655 w661 w668 w695 w706 w710 w719 w741 w835 w897 w903 w916 w939 w961 w970 w1021 w1124 w1278 w1369 w1438 w1451 w1497 w1512 w1578 w1652 w1663 w1668 w1694 w1728 w1748] -> w267
          tunnel: "update speed [ms]" -> [w298 _ _ _ _ _ _ _ _ _ _ _ _ _ _ _ _ _ _ _ _ _ _ _ _ _ _ _ _ _ _ _ _ _ _ _ _ _ _ _]
          tunnel: w264 -> [w295 _ _ _ _ _ _ _ _ _ _ _ _ _ _ _ _ _ _ _ _ _ _ _ _ w1019 _ _ _ _ _ _ _ _ _ _ _ _ w1712 _]
          tunnel: w262 -> [w297 _ _ _ _ _ _ w607 _ _ _ _ _ _ _ _ _ w743 w799 _ w905 _ _ _ _ w984 w1121 w1282 w1373 _ w1452 _ w1501 w1602 _ _ _ _ _ _]
          tunnel: w253 -> [_ _ _ _ _ _ _ w614 _ _ _ _ _ _ _ _ _ _ _ _ _ _ _ _ _ _ _ _ _ _ _ _ _ _ _ _ _ _ _ _]
          tunnel: w252 -> [_ _ _ _ _ _ _ _ _ _ _ _ _ _ _ _ _ _ _ _ _ _ _ _ _ _ _ _ _ _ _ _ _ _ _ _ _ w1684 _ _]
          frame "", "Idle" {
            # "executes when the state queue is empty"
            n235 = event shown="[0] Timeout" {
              selector: _ -> [_ _ _ _ _ _ _ _ _ _ _ _ _ _ _ _ _ _]
              dyn-events: _ -> [_ _ _ _ _ _ _ _ _ _ _ _ _ _ _ _ _ _]
              timeout: w298 -> [_ _ _ _ _ _ _ _ _ _ _ _ _ _ _ _ _ _]
              tunnel: w303 -> [w306 w433 w448 w467 w472 w477 w482 w488 w495 w500 w511 w516 w525 w530 w536 w542 w550 w556]
              tunnel: [w321 w432 w447 w466 w471 w476 w481 w487 w494 w499 w510 w515 w524 w529 w535 w541 w549 w555] -> w302
              tunnel: w301 -> [w311 w430 w444 w463 w469 w474 w479 w485 w492 w497 w509 w513 w518 w527 w533 w539 w547 w553]
              tunnel: [w315 w431 w446 w465 w470 w475 w480 w486 w493 w498 w501 w514 w523 w528 w534 w540 w548 w554] -> w300
              tunnel: w299 -> [w318 w431 w446 w465 w470 w475 w480 w486 w493 w498 w502 w514 w523 w528 w534 w540 w548 w554]
              tunnel: [w320 w430 w444 w462 w469 w474 w479 w485 w492 w497 w509 w513 w518 w527 w533 w539 w547 w553] -> w296
              tunnel: w297 -> [w338 _ w440 _ _ _ _ _ _ _ _ _ _ _ _ _ _ _]
              tunnel: w295 -> [_ _ w442 _ _ _ _ _ _ _ _ _ _ _ _ _ _ _]
              event Timeout {
                n236 = event-data() -> ()  [unwired: 1 in, 1 out]
                n237 = Unbundle By Name(w311) -> ("Centroid X"=w308:dbl[][], "Centroid Y"=w348:dbl[][], "Size"=w341:dbl[][], "detection para"=w337:T3[], "active cams"=w332:string[], "thresholds"=w329:cluster{"Lower value":sgl, "Upper value":sgl}[])
                n238 = Unbundle By Name(w311) -> ("active ccd"=w310:i32)
                n239 = call <userlib>:"Tick Count (ms)__ogtk.vi"("error in (no error)"=w318) -> ("error out"=w317:errorcluster, "millisecond timer value"=→"millisecond timer 2":u32)  [unwired: 9 in]
                n240 = for {
                  N: 12 ("Numeric 2") -> [_]
                  tunnel: w332 -> [w393] mode=indexing
                  tunnel: [w394] -> w346 mode=indexing
                  tunnel: w338 -> [w417]
                  tunnel: w337 -> [w415]
                  tunnel: [w413] -> w314 mode=indexing
                  tunnel: [w412] -> w312 mode=indexing
                  tunnel: [w410] -> w333 mode=indexing
                  tunnel: "autodetect" -> [w404]
                  tunnel: w317 -> [w418]
                  tunnel: [w419] -> w339
                  shift-right: [w401] -> w309
                  shift-left: w329 -> [w403]
                  shift-right: [w388] -> w347
                  shift-left: w308 -> [w390]
                  shift-right: [w384] -> w349
                  shift-left: w348 -> [w386]
                  shift-right: [w378] -> w340
                  shift-left: w341 -> [w380]
                  w382 = 0 ("index")
                  n241 = call-poly <userlib>:"Filter 1D Array__ogtk.vi"("items to filter"=w393, "array"=w417) -> ("filtered item indices"=w416:i32[])  [unwired: 4 in, 1 out]
                  n242 = Index Array(array=w416) -> (element=w379:i32)  [unwired: 1 in]
                  n243 = Index Array(array=w380, index (row)=w379) -> (element=w408:dbl[])  [unwired: 1 in]
                  n244 = Index Array(array=w386, index (row)=w379) -> (element=w409:dbl[])  [unwired: 1 in]
                  n245 = Index Array(array=w403, index=w379) -> (element=w407:cluster{"Lower value":sgl, "Upper value":sgl})
                  n246 = Index Array(array=w390, index (row)=w379) -> (element=w392:dbl[])  [unwired: 1 in]
                  n247 = Index Array(array=w415, index=w379) -> (element=w411:T3)
                  n248 = call "CENTRIOD DETECTION.vi"("Refnum in"=w393, "auto threshold"=w404, "Threshold Range In"=w407, "beam detection para"=w411, "error in (no error)"=w418) -> ("Bounding Rect"=w410:T35, "Particle Reports (Pixels)"=w412:T1, "Threshold Range Out"=w402:cluster{"Lower value":sgl, "Upper value":sgl}, "Centriod"=w420:cluster{"X":dbl, "Y":dbl}, "error out"=w419:errorcluster)  [unwired: 7 in, 3 out]
                  n249 = Unbundle By Name(w420) -> ("X"=w391:dbl, "Y"=w387:dbl)
                  n250 = Empty Array?(array=w412) -> (empty?=w414:bool)
                  n251 = Not(x=w414) -> (.not. x?=w413:bool)
                  n252 = Replace Array Subset(array=w403, new element=w402, index=w379) -> (w401:cluster{"Lower value":sgl, "Upper value":sgl}[])
                  n253 = Unbundle By Name(w410) -> ("Right"=w400:dbl, "Left"=w399:dbl, "Bottom"=w398:dbl, "Top"=w397:dbl)
                  n254 = Subtract(x=w400, y=w399) -> (x-y=w395:dbl)
                  n255 = Subtract(x=w398, y=w397) -> (x-y=w396:dbl)
                  n256 = Multiply(x=w395, y=w396) -> (x*y=w383:dbl)
                  n257 = Insert Into Array(array=w409, index=w382, new element=w387) -> (w385:dbl[])
                  n258 = Insert Into Array(array=w408, index=w382, new element=w383) -> (w381:dbl[])
                  n259 = Insert Into Array(array=w392, index=w382, new element=w391) -> (w389:dbl[])
                  n260 = for {
                    shift-right: [w421] -> w405
                    shift-left: dbl[] [] ("Array 4") -> [w424]
                    tunnel: w385 -> [w422] mode=indexing
                    n261 = Equal To 0?(x=w422) -> (x = 0?=w423:bool)
                    n262 = case shown="False" w423 {
                      tunnel: w424 -> [w427 w428]
                      tunnel: w422 -> [w426 _]
                      tunnel: [w425 w428] -> w421
                      frame False {
                        n263 = Build Array (concatenate)(w427, w426) -> (w425:dbl[])
                      }
                      frame True {
                      }
                    }
                  }
                  n264 = Replace Array Subset(array=w390, new element=w389, index (row)=w379) -> (w388:dbl[][])  [unwired: 1 in]
                  n265 = Replace Array Subset(array=w386, new element=w385, index (row)=w379) -> (w384:dbl[][])  [unwired: 1 in]
                  n266 = Replace Array Subset(array=w380, new element=w381, index (row)=w379) -> (w378:dbl[][])  [unwired: 1 in]
                  n267 = Array Size(array=w405) -> (size(s)=w394:i32)
                }
                "detected" <- w314
                "Particle Reports (Pixels)" <- w312
                "Box" <- w333
                n268 = Bundle(0, 1, "Centroid X"=w308) -> (→"Status":cluster{i32, i32, "Centroid X":dbl[][]})  [unwired: 1 in]
                n269 = Index Array(array=w312, index (row)=w310) -> (element=→"particles":T1)  [unwired: 1 in]
                n270 = call <vilib>:"Clear Errors.vi"("error in (no error)"=w339) -> ("error out"=w315:errorcluster)  [unwired: 6 in]
                n271 = local read "Img to avg"() -> (w323:i32)
                n272 = local read "Numeric"() -> (w326:dbl)
                n273 = Increment(x=w323) -> (x+1=w322:i32)
                n274 = Greater Or Equal?(x=w326, y=w322) -> (x >= y?=w319:bool)
                n275 = Increment(x=w326) -> (x+1=w325:dbl)
                n276 = Select(t=0.0, s=w319, f=w325) -> (s? t:f=w324:dbl)
                n277 = local write "Numeric"(w324) -> ()
                n278 = for {
                  tunnel: w346 -> [w370] mode=indexing
                  tunnel: w332 -> [w377] mode=indexing
                  shift-right: [w372] -> w342
                  shift-left: "" ("GUIdevice 7") -> [w375]
                  tunnel: [w365] -> w344 mode=indexing
                  tunnel: "Detection Rate" -> [w369]
                  tunnel: w324 -> [w367]
                  n279 = local read "Img to avg"() -> (w371:i32)
                  n280 = Greater Or Equal?(x=w370, y=w371) -> (x >= y?=w366:bool)
                  n281 = Multiply(x=w369, y=w367) -> (x*y=w368:dbl)
                  n282 = Greater Or Equal?(x=w370, y=w368) -> (x >= y?=w364:bool)
                  n283 = And(x=w366, y=w364) -> (x .and. y?=w365:bool)
                  n284 = Select(t=w377, s=w365, f="") -> (s? t:f=w373:string)
                  n285 = Concatenate Strings(w375, "\t", w373) -> (w372:string)
                }
                n286 = Bundle By Name(cluster=w311, "thresholds"=w309, "detected"=w314) -> (w330:T36)
                n287 = Bundle By Name(cluster=w330, "Centroid X"=w347, "Centroid Y"=w349, "Size"=w340) -> (w305:T36)
                n288 = Unbundle By Name(w305) -> ("img to avg"=w304:i32)
                n289 = Or Array Elements(Boolean array=w344) -> (logical OR=w343:bool)
                n290 = case shown="True" w319 {
                  tunnel: w305 -> [w350 w357]
                  tunnel: [w350 w356] -> w320
                  tunnel: w304 -> [_ w352]
                  frame False {
                  }
                  frame True {
                    n291 = Decrement(x=w352) -> (x-1=w351:i32)
                    n292 = Initialize Array(0.0 ("element"), 12 ("dimension size"), w351) -> (w353:dbl[][])
                    n293 = Bundle By Name(cluster=w357, "Centroid X"=w353, "Centroid Y"=w353, "Size"=w353) -> (w356:T36)
                  }
                }
                n294 = case shown="True" w343 {
                  tunnel: w342 -> [_ w362]
                  tunnel: w306 -> [w358 w360]
                  tunnel: [w358 w359] -> w321
                  frame False {
                  }
                  frame True {
                    n295 = call <vilib>:"Build State String with Arguments__jki_lib_state_machine.vi"("Arguments (\"\")"=w362, "State"="detected") -> ("State with Arguments"=w361:string)  [unwired: 4 in]
                    n296 = call <vilib>:"Add State(s) to Queue__jki_lib_state_machine.vi"("State(s) in (\"\")"=w360, "State(s) at Back (\"\")"=w361) -> ("States Out"=w359:string)  [unwired: 13 in]
                  }
                }
              }
              event "stop": Value Change {
                # "Exit Button Value Change (pressed) Event\n(this executes Macro: Exit to terminate the VI)"
                n297 = event-data() -> ()  [unwired: 1 in, 6 out]
                n298 = call <vilib>:"Add State(s) to Queue__jki_lib_state_machine.vi"("State(s) in Front (\"\")"="Macro: Exit", "State(s) in (\"\")"=w433) -> ("States Out"=w432:string)  [unwired: 13 in]
              }
              event Value Change {
                n299 = event-data() -> ()  [unwired: 1 in, 6 out]
                n300 = property on="Set Centriod Target" class="Bool (strict)"("Value"=FALSE) -> ()  [unwired: 2 in, 2 out]
                n301 = Unbundle By Name(w444) -> ("active ccd"=w436:i32, "Centroid X"=w435:dbl[][], "Centroid Y"=w434:dbl[][])
                n302 = Index Array(array=w440, index=w436) -> (element=w439:string)
                n303 = Concatenate Strings("Do want to update the target of " ("message"), w439, "?" ("string")) -> (w437:string)
                n304 = Two Button Dialog(message=w437) -> (T button?=w443:bool)  [unwired: 2 in]
                n305 = case shown="True" w443 {
                  tunnel: w442 -> [_ w455]
                  tunnel: w436 -> [_ w454]
                  tunnel: w435 -> [_ w461]
                  tunnel: w434 -> [_ w456]
                  frame False {
                  }
                  frame True {
                    n306 = Index Array(array=w461, index (row)=w454) -> (element=w460:dbl[])  [unwired: 1 in]
                    n307 = Index Array(array=w456, index (row)=w454) -> (element=w457:dbl[])  [unwired: 1 in]
                    n308 = Index Array(array=w455, index=w454) -> (element=w453:T30)
                    n309 = Unbundle By Name(w453) -> ("Target.X::12"=w452:refnum<vi>, "Target.Y::12"=w450:refnum<vi>)
                    n310 = Reverse 1D Array(array=w460) -> (reversed array=w459:dbl[])
                    n311 = Reverse 1D Array(array=w457) -> (reversed array=w458:dbl[])
                    n312 = Index Array(array=w459) -> (element=w451:dbl)  [unwired: 1 in]
                    n313 = Index Array(array=w458) -> (element=w449:dbl)  [unwired: 1 in]
                    n314 = property class="DigNum (strict)"(reference=w452, "Val(Sgnl)"=w451) -> ()  [unwired: 1 in, 2 out]
                    n315 = property class="DigNum (strict)"(reference=w450, "Val(Sgnl)"=w449) -> ()  [unwired: 1 in, 2 out]
                  }
                }
                n316 = call <vilib>:"Add State(s) to Queue__jki_lib_state_machine.vi"("State(s) in (\"\")"=w448) -> ("States Out"=w447:string)  [unwired: 14 in]
              }
              event "Feedback Global": Value Change {
                # "Exit Button Value Change (pressed) Event\n(this executes Macro: Exit to terminate the VI)"
                n317 = event-data() -> ("NewVal"=w464:bool)  [unwired: 1 in, 5 out]
                n318 = call <vilib>:"Add State(s) to Queue__jki_lib_state_machine.vi"("State(s) in (\"\")"=w467) -> ("States Out"=w466:string)  [unwired: 14 in]
                n319 = Bundle By Name(cluster=w463, "Feedback global"=w464) -> (w462:T36)
              }
              event Value Change {
                n320 = event-data() -> ()  [unwired: 1 in, 6 out]
                n321 = call <vilib>:"Add State(s) to Queue__jki_lib_state_machine.vi"("State(s) in Front (\"\")"="Move Config", "State(s) in (\"\")"=w472) -> ("States Out"=w471:string)  [unwired: 13 in]
              }
              event Value Change {
                n322 = event-data() -> ()  [unwired: 1 in, 6 out]
                n323 = call <vilib>:"Add State(s) to Queue__jki_lib_state_machine.vi"("State(s) in Front (\"\")"="Detection Config", "State(s) in (\"\")"=w477) -> ("States Out"=w476:string)  [unwired: 13 in]
              }
              event "associated motors": Value Change {
                n324 = event-data() -> ()  [unwired: 1 in, 6 out]
                n325 = call <vilib>:"Add State(s) to Queue__jki_lib_state_machine.vi"("State(s) in (\"\")"=w482, "State(s) at Back (\"\")"="Motor Config" ("State(s) at Back (\"\")")) -> ("States Out"=w481:string)  [unwired: 13 in]
              }
              event "Reset History": Value Change {
                n326 = event-data() -> ()  [unwired: 1 in, 6 out]
                n327 = call <vilib>:"Add State(s) to Queue__jki_lib_state_machine.vi"("State(s) in (\"\")"=w488, "State(s) at Back (\"\")"="Reset History" ("State(s) at Back (\"\")")) -> ("States Out"=w487:string)  [unwired: 13 in]
                n328 = property on="Reset History" class="Bool (strict)"("Value"=FALSE ("Reset History")) -> ()  [unwired: 2 in, 2 out]
              }
              event "ActiveMotor": Value Change {
                n329 = event-data() -> ("NewVal"=w490:u16)  [unwired: 1 in, 5 out]
                n330 = property on="ActiveMotor" class="Ring (strict)"() -> ("Strings []"=w491:string[])  [unwired: 2 in, 2 out]
                n331 = Index Array(array=w491, index=w490) -> (element=w489:string)
                n332 = property on="ActiveMotorName::99" class="Str"("Val(Sgnl)"=w489) -> ()  [unwired: 2 in, 2 out]
                n333 = call <vilib>:"Add State(s) to Queue__jki_lib_state_machine.vi"("State(s) in (\"\")"=w495) -> ("States Out"=w494:string)  [unwired: 14 in]
              }
              event "Save Config": Value Change {
                n334 = event-data() -> ()  [unwired: 1 in, 6 out]
                n335 = call <vilib>:"Add State(s) to Queue__jki_lib_state_machine.vi"("State(s) in (\"\")"=w500, "State(s) at Back (\"\")"="Save Config" ("State(s) at Back (\"\")")) -> ("States Out"=w499:string)  [unwired: 13 in]
              }
              event "Load Config": Value Change {
                n336 = event-data() -> ()  [unwired: 1 in, 6 out]
                n337 = call "File Dialog2"("error in"=w502, "pattern (all files)"="*.cfg", "pattern label"="config") -> ("selected path"=w506:path, "error out"=w501:errorcluster)  [unwired: 9 in, 2 out]
                n338 = Path To String(path=w506) -> (string=w504:string)
                "config path" <- w504
                n339 = call <vilib>:"Build State String with Arguments__jki_lib_state_machine.vi"("Arguments (\"\")"=w504, "State"="Load Config" ("State(s) at Back (\"\")")) -> ("State with Arguments"=w503:string)  [unwired: 4 in]
                n340 = call <vilib>:"Add State(s) to Queue__jki_lib_state_machine.vi"("State(s) in (\"\")"=w511, "State(s) at Back (\"\")"=w503) -> ("States Out"=w510:string)  [unwired: 13 in]
              }
              event "Save Stats": Value Change {
                n341 = event-data() -> ()  [unwired: 1 in, 6 out]
                n342 = call <vilib>:"Add State(s) to Queue__jki_lib_state_machine.vi"("State(s) in (\"\")"=w516, "State(s) at Back (\"\")"="Save Stats" ("State(s) at Back (\"\")")) -> ("States Out"=w515:string)  [unwired: 13 in]
              }
              event "active CCDs": Value Change {
                n343 = event-data() -> ("NewVal"=w522:i32)  [unwired: 1 in, 5 out]
                n344 = Unbundle By Name(w518) -> ("active cams"=w517:string[])
                n345 = Index Array(array=w517, index=w522) -> (element=w520:string)
                n346 = call <vilib>:"Build State String with Arguments__jki_lib_state_machine.vi"("Arguments (\"\")"=w520, "State"="active" ("State(s) at Back (\"\")")) -> ("State with Arguments"=w519:string)  [unwired: 4 in]
                n347 = call <vilib>:"Add State(s) to Queue__jki_lib_state_machine.vi"("State(s) in (\"\")"=w525, "State(s) at Back (\"\")"=w519) -> ("States Out"=w524:string)  [unwired: 13 in]
              }
              event "Center": Value Change {
                n348 = event-data() -> ()  [unwired: 1 in, 6 out]
                n349 = call <vilib>:"Add State(s) to Queue__jki_lib_state_machine.vi"("State(s) in (\"\")"=w530, "State(s) at Back (\"\")"="Center" ("State(s) at Back (\"\")")) -> ("States Out"=w529:string)  [unwired: 13 in]
              }
              event "new tdms": Value Change {
                n350 = event-data() -> ()  [unwired: 1 in, 6 out]
                n351 = property on="new tdms" class="Bool (strict)"("Value"=FALSE ("new tdms")) -> ()  [unwired: 2 in, 2 out]
                n352 = call <vilib>:"Add State(s) to Queue__jki_lib_state_machine.vi"("State(s) in (\"\")"=w536, "State(s) at Back (\"\")"="newtdms" ("State(s) at Back (\"\")")) -> ("States Out"=w535:string)  [unwired: 13 in]
              }
              event "deivice ini": Value Change {
                n353 = event-data() -> ()  [unwired: 1 in, 6 out]
                n354 = property on="deivice ini" class="Bool (strict)"("Value"=FALSE ("new tdms")) -> ()  [unwired: 2 in, 2 out]
                n355 = call <vilib>:"Add State(s) to Queue__jki_lib_state_machine.vi"("State(s) in (\"\")"=w542, "State(s) at Back (\"\")"="Device Ini" ("State(s) at Back (\"\")")) -> ("States Out"=w541:string)  [unwired: 13 in]
              }
              event "Img to avg": Value Change {
                n356 = event-data() -> ()  [unwired: 1 in, 6 out]
                n357 = property on="Img to avg" class="DigNum (strict)"() -> ("Value"=w545:i32)  [unwired: 2 in, 2 out]
                n358 = Number To Decimal String(number=w545) -> (decimal integer string=w544:string)  [unwired: 1 in]
                n359 = call <vilib>:"Build State String with Arguments__jki_lib_state_machine.vi"("Arguments (\"\")"=w544, "State"="ImgToAvg" ("State(s) at Back (\"\")")) -> ("State with Arguments"=w543:string)  [unwired: 4 in]
                n360 = call <vilib>:"Add State(s) to Queue__jki_lib_state_machine.vi"("State(s) in (\"\")"=w550, "State(s) at Back (\"\")"=w543) -> ("States Out"=w549:string)  [unwired: 13 in]
              }
              event Panel Close? {
                # "Discard the event because we'll close the front panel ourselves in Macro: Exit"
                # "Close Panel button (pressed) Event\n(this executes Macro: Exit to terminate the VI)"
                n361 = event-data() -> ()  [unwired: 1 in, 1 out]
                n362 = call <vilib>:"Add State(s) to Queue__jki_lib_state_machine.vi"("State(s) in Front (\"\")"="Macro: Exit", "State(s) in (\"\")"=w556) -> ("States Out"=w555:string)  [unwired: 13 in]
                n363 = event-data("Discard?"=TRUE) -> ()  [unwired: 1 in, 1 out]
              }
            }
          }
          frame "---------- Core ----------" {
            # "Do not put any code in this frame.\n(it is a separator no-op)"
            n364 = call <vilib>:"Add State(s) to Queue__jki_lib_state_machine.vi"("State(s) in (\"\")"=w560) -> ("States Out"=w559:string)  [unwired: 14 in]
          }
          frame Default {
            w570 = 42 items=["No error", "Argument error", "Memory is full", "Out of zone", "End of file", "File already open", "Generic file I/O error", "File not found", "File permission error", "Disk is full", "Duplicate path", "Too many files open", "System feature not enabled", "Resource file not found", "Cannot add resource", "Resource not found", "Image not found", "Image memory error", "Pen does not exist", "Config type invalid", "Config token not found", "Config parse error", "Config memory error", "Bad external code format", "Bad external code offset", "External code not present", "Null window", "Destroy window error", "Null menu", "Print aborted", "Bad print record", "Print driver error", "Windows error during printing", "Memory error during printing", "Print dialog error", "Generic print error", "Invalid device refnum", "Device not found", "Device parameter error", "Device unit error", "Cannot open device", "Device call aborted", "Generic error", "Cancelled by user", "Object ID too low", "Object ID too high", "Object not in heap", "Unknown heap", "Unknown object (invalid DefProc)", "Unknown object (DefProc not in table)", "Message out of range", "Invalid (null) method", "Unknown message", "Manager call not supported", "Bad address", "Network operation in progress", "Network operation timed out", "Connection is busy", "Network attribute not supported", "Network error", "Address in use", "System out of memory", "Connection aborted", "Connection refused", "Not connected", "Already connected", "Connection closed", "Initialization error (interapplication manager)", "Bad occurrence", "Wait on unbound occurrence handler", "Occurrence queue overflow", "Datalog type conflict", "Unused", "Unrecognized type (interapplication manager)", "Memory corrupt", "Failed to make temporary DLL", "Old CIN version", "Drag socket not found", "Failed to load drop-object", "Failed to register OLE object", "Failed to release OLE object", "Format specifier type mismatch", "Unknown format specifier", "Too few format specifiers", "Too many format specifiers", "Scan failed", "Newer CIN version", "Error converting to variant", "Runtime menu error", "Password tampered", "Variant attribute not found", "Incompatible variant data type", "Event data is not available", "Event Store is not present", "Occurrence is not found", "Event Queue is not created", "Event info is not available", "Refnum passed is NULL", "Error retrieving Class GUID", "Error retrieving CoClass GUID", "Error retrieving TypeLib GUID.", "Bad built application magic bytes.", "Specific driver is different from the specific driver associated with the Logical Name.", "There is no session opened to the class driver.", "Max Error", "MAX - Error with config objects", "MAX - Error loading configuration", "MAX - Group not supported"]
            # "Current State"
            # "Do not delete, rename, or modify this frame.\n(this is used to capture unhandled states and typos)"
            # "Handle mistyped state name (developer tool)"
            n365 = Format Into String(format string="Software Exception: Unhandled State \"%s\"." ("message"), error in=w566, w561) -> (resulting string=w569:string, error out=w568:errorcluster)  [unwired: 1 in]
            n366 = call <vilib>:"Error Cluster From Error Code.vi"("show call chain? (False)"=TRUE, "error in (no error)"=w568, "error message (\"\")"=w569, "error code (0)"=w570) -> ("error out"=w567:errorcluster)  [unwired: 5 in]
            n367 = call <vilib>:"Add State(s) to Queue__jki_lib_state_machine.vi"("State(s) in (\"\")"=w565) -> ("States Out"=w564:string)  [unwired: 14 in]
          }
          frame "Initialize Core Data" {
            # "Do not delete, rename, or modify this frame.\n(this is used to determine panel behavior on exit)"
            # "originally closed?"
            # "exe?"
            # "If panel starts closed or is an EXE, then close it when we exit"
            n368 = property class="VI"() -> ("Front Panel.Open"=w580:bool)  [unwired: 2 in, 2 out]
            n369 = property class="App"() -> ("App.Kind"=w579:T16)  [unwired: 2 in, 2 out]
            n370 = control-ref of="Current VI Reference"() -> (w574:refnum<vi>)
            n371 = Not(x=w580) -> (.not. x?=w577:bool)
            n372 = Equal?(x=w579, y=T16."Run Time System" ("Application:Kind")) -> (x = y?=w576:bool)
            n373 = Or(x=w577, y=w576) -> (x .or. y?=w575:bool)
            n374 = Bundle By Name(cluster=w573, "Core.Current VI Reference"=w574, "Core.Close Panel on Exit?"=w575) -> (w572:T36)
            n375 = call <vilib>:"Add State(s) to Queue__jki_lib_state_machine.vi"("State(s) in (\"\")"=w583) -> ("States Out"=w582:string)  [unwired: 14 in]
          }
          frame "Error Handler" {
            w584 = T37 0 items=["no dialog", "OK message", "continue or stop message", "OK message + warnings", "continue/stop + warnings"] ("type of dialog (OK msg:1)")
            # "Unhandled Error -- Display it"
            # "Handle any errors here.\nYou can also output any states to clean-up after errors occur"
            # "Clear error"
            n376 = call <vilib>:"General Error Handler.vi"("type of dialog (OK msg:1)"=w584, "error in (no error)"=w586) -> ()  [unwired: 9 in, 5 out]
            n377 = call <vilib>:"Add State(s) to Queue__jki_lib_state_machine.vi"("State(s) in Front (\"\")"="/* Post Error States", "State(s) in (\"\")"=w590) -> ("States Out"=w589:string)  [unwired: 13 in]
          }
          frame "Exit" {
            # "Do not put any code in this frame.\n(No errors that occur here will be handled.)"
            n378 = call <vilib>:"Add State(s) to Queue__jki_lib_state_machine.vi"("State(s) in (\"\")"=w595) -> ("States Out"=w594:string)  [unwired: 14 in]
          }
          frame "---------- Data ----------" {
            # "Do not put any code in this frame.\n(It is a separator no-op. You can make a copy of this frame to create a new Data frame)"
            n379 = call <vilib>:"Add State(s) to Queue__jki_lib_state_machine.vi"("State(s) in (\"\")"=w599) -> ("States Out"=w598:string)  [unwired: 14 in]
          }
          frame "Data: Initialize" {
            w611 = bool[] [FALSE, FALSE, FALSE, FALSE, FALSE, FALSE, FALSE, FALSE, FALSE, FALSE, FALSE, TRUE]  # speedmode Y
            w612 = bool[] [FALSE, FALSE, FALSE, FALSE, FALSE, FALSE, FALSE, FALSE, FALSE, FALSE, FALSE, TRUE]  # speedmode X
            w613 = bool[] [FALSE, FALSE, FALSE, FALSE, TRUE, TRUE, TRUE, FALSE, FALSE, FALSE, FALSE, FALSE]  # detected
            w615 = cluster{"Lower value":sgl, "Upper value":sgl}[] [{"Lower value"=93.0, "Upper value"=255.0}, {"Lower value"=105.0, "Upper value"=255.0}, {"Lower value"=0.0, "Upper value"=255.0}, {"Lower value"=127.0, "Upper value"=255.0}, {"Lower value"=0.0, "Upper value"=255.0}, {"Lower value"=0.0, "Upper value"=255.0}, {"Lower value"=0.0, "Upper value"=255.0}, {"Lower value"=0.0, "Upper value"=255.0}, {"Lower value"=0.0, "Upper value"=255.0}, {"Lower value"=0.0, "Upper value"=255.0}, {"Lower value"=0.0, "Upper value"=255.0}, {"Lower value"=0.0, "Upper value"=255.0}]  # thresholds
            w626 = FALSE  # Feedback global
            w628 = 0  # active ccd
            w600 = 2  # img to avg
            w639 = T38 {"Current VI Reference"=refnum, "Close Panel on Exit?"=FALSE}  # Core
            # "Initialize the shift-register data, here.\n(data names are defined by what you wire into the bundle function)"
            n380 = TDMS Open(6:FALSE ("disable buffering (T)"), 7:enum16{"1.0", "2.0"}."2.0" ("file format version (2.0)"), 8:w616, 10:T17."create or replace" ("operation"), 11:w614) -> (0:w610:errorcluster, 3:w608:refnum<k34>)  [unwired: 2 in]
            n381 = call "TDMSbuffersize.vi"("error in (no error)"=w610, "group names"=w607, "Data Value Reference in"=w608) -> ("error out"=w609:errorcluster, "Data Value Reference out"=w606:refnum<k34>)  [unwired: 7 in]
            n382 = call <vilib>:"Add State(s) to Queue__jki_lib_state_machine.vi"("State(s) in (\"\")"=w641) -> ("States Out"=w640:string)  [unwired: 14 in]
            n383 = Bundle("Core"=w639, "detection para"="detection para", "thresholds"=w615, "Centroid X"="Centroid X", "Centroid Y"="Centroid Y", "img to avg"=w600, "Mean Centroid X"="Mean Centroid X", "Mean Centroid Y"="Mean Centroid Y", "Offset X"="Offset X", "Offset Y"="Offset Y", "Offset X stats"="Offset X stats", "Offset Y stats"="Offset Y stats", "Size"="Size", "Mean Size"="Mean Size", "Time"="Time", "move properties"="move properties", "active axis refs 2"="active axis refs 2", "active ccd"=w628, "Feedback global"=w626, "Motor X"="Motor X", "Motor Y"="Motor Y", "active cams"="active cams", "Data Value Reference out"=w606, "detected"=w613, "speedmode X"=w612, "speedmode Y"=w611) -> (w602:T36)  [unwired: 1 in]
            n384 = Initialize Array(0.0 ("element"), 12 ("dimension size"), w600) -> (w603:dbl[][])
            n385 = Bundle By Name(cluster=w602, "Centroid X"=w603, "Centroid Y"=w603, "Size"=w603) -> (w601:T36)
          }
          frame "Data: Cleanup" {
            # "Cleanup any data and references, here.\n(this is called automatically, by the Macro: Exit)"
            n386 = Unbundle By Name(w645) -> ("Core.Current VI Reference"=w646:refnum<vi>)
            n387 = Close Reference(reference=w646, error in (no error)=w647) -> (error out=w643:errorcluster)
            n388 = Unbundle By Name(w645) -> ("Data Value Reference out"=w644:refnum<k34>)
            n389 = TDMS Close(8:w643, 11:w644) -> (0:w642:errorcluster)  [unwired: 1 out]
            n390 = call <vilib>:"Add State(s) to Queue__jki_lib_state_machine.vi"("State(s) in (\"\")"=w649) -> ("States Out"=w648:string)  [unwired: 14 in]
          }
          frame "---------- UI ----------" {
            # "Do not put any code in this frame.\n(It is a separator no-op. You can make a copy of this frame to create a new UI frame)"
            n391 = call <vilib>:"Add State(s) to Queue__jki_lib_state_machine.vi"("State(s) in (\"\")"=w653) -> ("States Out"=w652:string)  [unwired: 14 in]
          }
          frame "UI: Initialize" {
            # "Initialize the User Interface, here.\n(this is called automatically, by the Macro: Init)"
            n392 = call <vilib>:"Add State(s) to Queue__jki_lib_state_machine.vi"("State(s) in (\"\")"=w657) -> ("States Out"=w656:string)  [unwired: 14 in]
          }
          frame "UI: Cursor Set" {
            # "Argument"
            # "Set and Unset Cursor Busy.\n(Usage: \"UI: Cursor Set >> Busy|Idle\")"
            n393 = case shown="\"Idle\", Default" w658 {
              tunnel: w660 -> [w665 w667]
              tunnel: [w664 w666] -> w659
              frame "Idle", Default {
                n394 = call <vilib>:"Unset Busy.vi"("error in (no error)"=w665) -> ("error out"=w664:errorcluster)  [unwired: 10 in]
              }
              frame "Busy" {
                n395 = call <vilib>:"Set Busy.vi"("error in (no error)"=w667) -> ("error out"=w666:errorcluster)  [unwired: 9 in, 1 out]
              }
            }
            n396 = call <vilib>:"Add State(s) to Queue__jki_lib_state_machine.vi"("State(s) in (\"\")"=w663) -> ("States Out"=w662:string)  [unwired: 14 in]
          }
          frame "UI: Front Panel State" {
            # "Argument"
            # "Set Front Panel Open or Closed\n(Usage: \"UI: Front Panel State >> Open|Close\")"
            n397 = Unbundle By Name(w668) -> ("Core.Current VI Reference"=w670:refnum<vi>)
            n398 = case shown="\"Open\", Default" w669 {
              tunnel: w672 -> [w678 w689]
              tunnel: [w679 w690] -> w671
              tunnel: w670 -> [_ _]
              frame "Open", Default {
                n399 = property class="VI"(error in=w678) -> (reference out=w676:refnum<vi>, error out=w677:errorcluster, "Front Panel.Open"=w675:bool)  [unwired: 1 in]
                n400 = case shown="False" w675 {
                  tunnel: [w682 w685] -> w679
                  tunnel: w677 -> [w681 w685]
                  tunnel: w676 -> [w680 _]
                  frame False {
                    n401 = invoke class="VI" method="FP.Open"(reference=w680, error in=w681, "Activate"=TRUE, "State"=T18."Standard") -> (error out=w682:errorcluster)  [unwired: 1 in, 4 out]
                  }
                  frame True {
                  }
                }
              }
              frame "Close" {
                n402 = property class="VI"(error in=w689) -> (reference out=w687:refnum<vi>, error out=w688:errorcluster, "Front Panel.Open"=w686:bool)  [unwired: 1 in]
                n403 = case shown="True" w686 {
                  tunnel: [w691 w694] -> w690
                  tunnel: w688 -> [w691 w693]
                  tunnel: w687 -> [_ w692]
                  frame False {
                  }
                  frame True {
                    n404 = invoke class="VI" method="FP.Close"(reference=w692, error in=w693) -> (error out=w694:errorcluster)  [unwired: 1 in, 2 out]
                  }
                }
              }
            }
            n405 = call <vilib>:"Add State(s) to Queue__jki_lib_state_machine.vi"("State(s) in (\"\")"=w674) -> ("States Out"=w673:string)  [unwired: 14 in]
          }
          frame "---------- Macro ----------" {
            # "Do not put any code in this frame.\n(It is a separator no-op. You can make a copy of this frame to create a new Macro frame)"
            n406 = call <vilib>:"Add State(s) to Queue__jki_lib_state_machine.vi"("State(s) in (\"\")"=w698) -> ("States Out"=w697:string)  [unwired: 14 in]
          }
          frame "Macro: Initialize" {
            w705 = "Data: Initialize\nInitialize Core Data\nUI: Initialize\nUI: Front Panel State >> Open\nDevice Ini >> 3000"  # Data: Initialize Initialize Core Data UI: Initialize UI: Front Panel State >> Open Device Ini >> 3000
            # "Initialization Macro\n(This is called once, when the VI starts)"
            n407 = property on="Img to avg" class="DigNum (strict)"() -> ("Value"=w703:i32)  [unwired: 2 in, 2 out]
            n408 = call <vilib>:"Add State(s) to Queue__jki_lib_state_machine.vi"("State(s) in Front (\"\")"=w705, "State(s) in (\"\")"=w708) -> ("States Out"=w700:string)  [unwired: 13 in]
            n409 = Number To Decimal String(number=w703) -> (decimal integer string=w702:string)  [unwired: 1 in]
            n410 = call <vilib>:"Build State String with Arguments__jki_lib_state_machine.vi"("Arguments (\"\")"=w702, "State"="ImgToAvg") -> ("State with Arguments"=w701:string)  [unwired: 4 in]
            n411 = call <vilib>:"Add State(s) to Queue__jki_lib_state_machine.vi"("State(s) in (\"\")"=w700, "State(s) at Back (\"\")"=w701) -> ("States Out"=w699:string)  [unwired: 13 in]
          }
          frame "Macro: Exit" {
            # "Exit Macro\n(This is called once, when the VI exits)"
            n412 = Unbundle By Name(w710) -> ("Core.Close Panel on Exit?"=w709:bool)
            n413 = Select(t="UI: Front Panel State >> Close", s=w709, f="") -> (s? t:f=w713:string)
            n414 = call <vilib>:"Add State(s) to Queue__jki_lib_state_machine.vi"("State(s) in (\"\")"=w713, "State(s) at Back (\"\")"="Data: Cleanup\nExit") -> ("States Out"=w711:string)  [unwired: 13 in]
            n415 = call <vilib>:"Add State(s) to Queue__jki_lib_state_machine.vi"("State(s) in Front (\"\")"=w711, "State(s) in (\"\")"=w718) -> ("States Out"=w717:string)  [unwired: 13 in]
          }
          frame "---------- Ini and Configure ----------" {
            # "Template Separator\n(You can make a copy of, or modify, this frame)"
            n416 = call <vilib>:"Add State(s) to Queue__jki_lib_state_machine.vi"("State(s) in (\"\")"=w722) -> ("States Out"=w721:string)  [unwired: 14 in]
          }
          frame "Device Ini" {
            # "Your code here.\n(You can make a copy of, or modify, this frame)"
            n417 = Empty String/Path?(string/path=w739) -> (empty?=w737:bool)
            n418 = case shown="False" w737 {
              tunnel: w739 -> [w776 _]
              tunnel: [w775 0] -> w738
              frame False {
                n419 = Decimal String To Number(string=w776) -> (number=w775:i32)  [unwired: 2 in, 1 out]
              }
              frame True {
              }
            }
            n420 = flat-sequence {
              tunnel: w743 -> [w779]
              tunnel: [w779] -> w742
              tunnel: w738 -> [w778]
              tunnel: w742 -> [w782]
              tunnel: [w780] -> w728
              frame #0 {
                n421 = Wait (ms)(milliseconds to wait=w778) -> ()  [unwired: 1 out]
              }
              frame #1 {
                n422 = for {
                  tunnel: w782 -> [w784] mode=indexing
                  shift-right: [w785] -> w780
                  shift-left: string[] [] -> [w786]
                  n423 = Empty String/Path?(string/path=w784) -> (empty?=w783:bool)
                  n424 = case shown="False" w783 {
                    tunnel: w786 -> [w789 w795]
                    tunnel: [w788 w795] -> w785
                    tunnel: w784 -> [w787 _]
                    frame False {
                      n425 = call "send command.vi"("Device Name"=w787) -> ("status"=w790:bool)  [unwired: 4 in]
                      n426 = case shown="True" w790 {
                        tunnel: w789 -> [w791 w794]
                        tunnel: [w791 w793] -> w788
                        tunnel: w787 -> [_ w792]
                        frame False {
                        }
                        frame True {
                          n427 = Build Array (concatenate)(w794, w792) -> (w793:string[])
                        }
                      }
                    }
                    frame True {
                    }
                  }
                }
              }
            }
            n428 = Unbundle By Name(w736) -> ("active cams"=w729:string[])
            n429 = call <vilib>:"Add State(s) to Queue__jki_lib_state_machine.vi"("State(s) in (\"\")"=w744) -> ("States Out"=w731:string)  [unwired: 14 in]
            n430 = Empty Array?(array=w729) -> (empty?=w733:bool)
            n431 = Equal?(x=w729, y=w728) -> (x = y?=w734:bool[])
            n432 = Not(x=w733) -> (.not. x?=w732:bool)
            n433 = Build Array (concatenate)(w734, w732) -> (w735:bool[])
            n434 = Array Size(array=w728) -> (size(s)=w726:i32)
            n435 = Array Size(array=w729) -> (size(s)=w727:i32)
            n436 = Equal?(x=w727, y=w726) -> (x = y?=w725:bool)
            n437 = And Array Elements(Boolean array=w735) -> (logical AND=w724:bool)
            n438 = And(x=w725, y=w724) -> (x .and. y?=w723:bool)
            n439 = case shown="False" w723 {
              tunnel: [w761 w774] -> w741
              tunnel: w736 -> [w746 w774]
              tunnel: w728 -> [w747 _]
              tunnel: w731 -> [w756 w773]
              tunnel: [w754 w773] -> w730
              frame False {
                n440 = Bundle By Name(cluster=w746, "active cams"=w747) -> (w762:T36)
                n441 = property on="active CCDs" class="LstBox (strict)"("Item Names"=w747) -> ()  [unwired: 2 in, 2 out]
                n442 = Array Size(array=w747) -> (size(s)=w765:i32)
                n443 = for {
                  N: 1 -> [_]
                  shift-right: [w767] -> w760
                  shift-left: timestamp[][] [] ("Time") -> [w769]
                  n444 = for {
                    N: 12 -> [_]
                    tunnel: w769 -> [w772] mode=indexing
                    tunnel: [w770] -> w767 mode=indexing
                    n445 = Get Date/Time In Seconds() -> (seconds since 1Jan1904=w771:timestamp)
                    n446 = Build Array (concatenate)(w772, w771) -> (w770:timestamp[])
                  }
                }
                n447 = Unbundle By Name(w746) -> ("img to avg"=w745:i32)
                n448 = Initialize Array(0.0 ("element"), w765, 0 ("dimension size")) -> (w763:dbl[][])
                n449 = Initialize Array(0.0 ("element"), 12 ("dimension size"), w745) -> (w748:dbl[][])
                n450 = Bundle By Name(cluster=w762, "Offset X stats"=w763, "Offset Y stats"=w763, "Centroid X"=w748, "Centroid Y"=w748, "Mean Centroid X"=w763, "Mean Centroid Y"=w763, "Offset X"=w763, "Offset Y"=w763, "Size"=w748, "Mean Size"=w763, "Motor X"=w763, "Motor Y"=w763) -> (w761:T36)
                n451 = property on="Time" class="Arr (strict)"("Value"=w760) -> ()  [unwired: 2 in, 2 out]
                n452 = property on="config path" class="Str"() -> ("Value"=w753:string)  [unwired: 2 in, 2 out]
                n453 = call <vilib>:"Add State(s) to Queue__jki_lib_state_machine.vi"("State(s) in Front (\"\")"="newtdms\nMove Config\nDetection Config\nactive\nCenter" ("State(s) in Front (\"\")"), "State(s) in (\"\")"=w756) -> ("States Out"=w755:string)  [unwired: 13 in]
                n454 = call <vilib>:"Build State String with Arguments__jki_lib_state_machine.vi"("Arguments (\"\")"=w753, "State"="Load Config" ("State(s) in Front (\"\")")) -> ("State with Arguments"=w751:string)  [unwired: 4 in]
                n455 = call <vilib>:"Add State(s) to Queue__jki_lib_state_machine.vi"("State(s) in Front (\"\")"=w751, "State(s) in (\"\")"=w755) -> ("States Out"=w754:string)  [unwired: 13 in]
                "name array" <- w747
              }
              frame True {
              }
            }
          }
          frame "Load Config" {
            # "Your code here.\n(You can make a copy of, or modify, this frame)"
            n456 = Unbundle By Name(w798) -> ("detection para"=w841:T3[], "move properties"=w838:T2[], "thresholds"=w833:cluster{"Lower value":sgl, "Upper value":sgl}[])
            n457 = Empty String/Path?(string/path=w797) -> (empty?=w796:bool)
            n458 = property on="Load Config" class="Bool (strict)"("Value"=FALSE ("Load Config")) -> ()  [unwired: 2 in, 2 out]
            n459 = case shown="False" w796 {
              tunnel: [w852 T5 {"CCDs"=[], "move properties"=[], "detection para"=[], "thresholds"=[], "Value"={"Motor CCD 1"=0, "Motor CCD 2"=0, "Motor CCD 3"=0, "Motor CCD 4"=0, "Motor CCD 5"=0, "Motor CCD 6"=0, "Motor CCD 7"=0, "Motor CCD 8"=0, "Motor CCD 9"=0, "Motor CCD 10"=0, "Motor CCD 11"=0, "Motor CCD 12"=0}} ("output cluster 2")] -> w843
              tunnel: [w850 w859] -> w803
              tunnel: w797 -> [w849 _]
              tunnel: w800 -> [w847 w859]
              tunnel: w798 -> [_ _]
              frame False {
                n460 = String To Path(string=w849) -> (path=w848:path)
                n461 = Open/Create/Replace File(file path (use dialog)=w848, error in=w847, operation (0:open)=T19."open or create") -> (refnum out=w854:refnum<file>, error out=w855:errorcluster)  [unwired: 3 in, 1 out]
                n462 = Read from Binary File(5:"output cluster 2", 8:w855, 11:w854) -> (0:w856:errorcluster, 2:w852:T5, 3:w857:refnum<file>)  [unwired: 3 in, 1 out]
                n463 = Close File(refnum=w857, error in=w856) -> (error out=w850:errorcluster)  [unwired: 1 out]
              }
              frame True {
              }
            }
            n464 = Unbundle By Name(w843) -> ("Value"=w830:T7, "CCDs"=w842:string[], "detection para"=w840:T3[], "move properties"=w839:T2[], "thresholds"=w834:cluster{"Lower value":sgl, "Upper value":sgl}[])
            n465 = Cluster To Array(cluster=w830) -> (array=w831:u16[])
            n466 = call <vilib>:"Add State(s) to Queue__jki_lib_state_machine.vi"("State(s) in (\"\")"=w846, "State(s) at Back (\"\")"="Motor Config" ("State(s) at Back (\"\")")) -> ("States Out"=w845:string)  [unwired: 13 in]
            n467 = for {
              tunnel: w842 -> [w875]
              tunnel: w840 -> [w877]
              tunnel: w839 -> [w876]
              shift-right: [w869] -> w837
              shift-left: w841 -> [w874]
              shift-right: [w867] -> w836
              shift-left: w838 -> [w873]
              tunnel: w799 -> [w872] mode=indexing
              tunnel: w834 -> [w868]
              shift-right: [w864] -> w832
              shift-left: w833 -> [w866]
              tunnel: w831 -> [w863]
              tunnel: [w860] -> w829 mode=indexing
              i -> [w861]
              n468 = call-poly <userlib>:"Filter 1D Array__ogtk.vi"("items to filter"=w872, "array"=w875) -> ("filtered item indices"=w878:i32[])  [unwired: 4 in, 1 out]
              n469 = Index Array(array=w878) -> (element=w862:i32)  [unwired: 1 in]
              n470 = Index Array(array=w863, index=w862) -> (element=w860:u16)
              n471 = Index Array(array=w877, index=w862) -> (element=w871:T3)
              n472 = Index Array(array=w876, index=w862) -> (element=w870:T2)
              n473 = Index Array(array=w868, index=w862) -> (element=w865:cluster{"Lower value":sgl, "Upper value":sgl})
              n474 = Replace Array Subset(array=w874, new element=w871, index=w861) -> (w869:T3[])
              n475 = Replace Array Subset(array=w873, new element=w870, index=w861) -> (w867:T2[])
              n476 = Replace Array Subset(array=w866, new element=w865, index=w861) -> (w864:cluster{"Lower value":sgl, "Upper value":sgl}[])
            }
            n477 = Index Array(array=w829, index #1=0 ("index (row)"), index #2=1 ("index (row)"), index #3=2 ("index (row)"), index #4=3 ("index (row)"), index #5=4 ("index (row)"), index #6=5 ("index (row)"), index #7=6 ("index (row)"), index #8=7 ("index (row)"), index #9=8 ("index (row)"), index #10=9 ("index (row)"), index #11=10 ("index (row)"), index #12=11 ("index (row)")) -> (element #1=w816:u16, element #2=w815:u16, element #3=w814:u16, element #4=w813:u16, element #5=w812:u16, element #6=w811:u16, element #7=w810:u16, element #8=w809:u16, element #9=w808:u16, element #10=w807:u16, element #11=w806:u16, element #12=w805:u16)
            n478 = Bundle By Name(cluster=w830, "Motor CCD 1"=w816, "Motor CCD 2"=w815, "Motor CCD 3"=w814, "Motor CCD 4"=w813, "Motor CCD 5"=w812, "Motor CCD 6"=w811, "Motor CCD 7"=w810, "Motor CCD 8"=w809, "Motor CCD 9"=w808, "Motor CCD 10"=w807, "Motor CCD 11"=w806, "Motor CCD 12"=w805) -> (w804:T7)
            n479 = Bundle By Name(cluster=w798, "detection para"=w837, "move properties"=w836, "thresholds"=w832) -> (w835:T36)
            n480 = property on="associated motors" class="Clust (strict)"(error in=w803, "Val(Sgnl)"=w804) -> (error out=w802:errorcluster)  [unwired: 1 in, 1 out]
          }
          frame "Save Config" {
            # "Your code here.\n(You can make a copy of, or modify, this frame)"
            n481 = Unbundle By Name(w897) -> ("move properties"=w884:T2[], "detection para"=w892:T3[], "thresholds"=w881:cluster{"Lower value":sgl, "Upper value":sgl}[])
            n482 = property on="associated motors" class="Clust (strict)"() -> ("Value"=w891:T7)  [unwired: 2 in, 2 out]
            n483 = property on="Save Config" class="Bool (strict)"("Value"=FALSE ("Save Config")) -> ()  [unwired: 2 in, 2 out]
            n484 = local read "CCDs"() -> (w882:string[])
            n485 = call "File Dialog"("error in"=w880, "pattern (all files)"="*.cfg", "pattern label"="config") -> ("selected path"=w886:path, "error out"=w879:errorcluster)  [unwired: 9 in, 2 out]
            n486 = Bundle("CCDs"=w882, "move properties"=w884, "detection para"=w892, "thresholds"=w881, "Value"=w891) -> (w885:T5)  [unwired: 1 in]
            n487 = Open/Create/Replace File(file path (use dialog)=w886, error in=w879, operation (0:open)=T19."replace or create with confirmation") -> (refnum out=w893:refnum<file>, error out=w894:errorcluster)  [unwired: 3 in, 1 out]
            n488 = Write to Binary File(file (use dialog)=w893, data=w885, error in=w894) -> (refnum out=w896:refnum<file>, error out=w895:errorcluster)  [unwired: 3 in, 1 out]
            n489 = Close File(refnum=w896, error in=w895) -> (error out=w889:errorcluster)  [unwired: 1 out]
            n490 = call <vilib>:"Add State(s) to Queue__jki_lib_state_machine.vi"("State(s) in (\"\")"=w899) -> ("States Out"=w898:string)  [unwired: 14 in]
          }
          frame "active" {
            # "Your code here.\n(You can make a copy of, or modify, this frame)"
            n491 = call-poly <userlib>:"Filter 1D Array__ogtk.vi"("items to filter"=w909, "array"=w905) -> ("filtered item indices"=w908:i32[])  [unwired: 4 in, 1 out]
            n492 = Unbundle By Name(w904) -> ("move properties"=w907:T2[], "detection para"=w902:T3[])  [unwired: 1 out]
            n493 = Index Array(array=w908) -> (element=w900:i32)  [unwired: 1 in]
            n494 = Index Array(array=w907, index=w900) -> (element=w906:T2)
            n495 = Index Array(array=w902, index=w900) -> (element=w901:T3)
            n496 = property on="move config" class="Clust (strict)"("Value"=w906) -> ()  [unwired: 2 in, 2 out]
            n497 = property on="beam detection para" class="Clust (strict)"("Value"=w901) -> ()  [unwired: 2 in, 2 out]
            n498 = Bundle By Name(cluster=w904, "active ccd"=w900) -> (w903:T36)
            n499 = call <vilib>:"Add State(s) to Queue__jki_lib_state_machine.vi"("State(s) in (\"\")"=w912) -> ("States Out"=w911:string)  [unwired: 14 in]
          }
          frame "Detection Config" {
            # "Your code here.\n(You can make a copy of, or modify, this frame)"
            n500 = Unbundle By Name(w917) -> ("detection para"=w913:T3[], "active ccd"=w918:i32)
            n501 = Replace Array Subset(array=w913, new element="beam detection para", index=w918) -> (w914:T3[])
            n502 = Bundle By Name(cluster=w917, "detection para"=w914) -> (w916:T36)
            n503 = call <vilib>:"Add State(s) to Queue__jki_lib_state_machine.vi"("State(s) in (\"\")"=w921) -> ("States Out"=w920:string)  [unwired: 14 in]
          }
          frame "Motor Config" {
            # "Your code here.\n(You can make a copy of, or modify, this frame)"
            n504 = Unbundle By Name("associated motors") -> ("Motor CCD 1"=w943:u16, "Motor CCD 2"=w944:u16, "Motor CCD 3"=w945:u16, "Motor CCD 4"=w938:u16, "Motor CCD 5"=w937:u16, "Motor CCD 6"=w936:u16, "Motor CCD 7"=w935:u16, "Motor CCD 8"=w934:u16, "Motor CCD 9"=w933:u16, "Motor CCD 10"=w932:u16, "Motor CCD 11"=w931:u16, "Motor CCD 12"=w930:u16)
            n505 = local read "motor refs"() -> (w941:refnum<vi>[])
            n506 = property on="ActiveMotor" class="Ring (strict)"() -> ("Value"=w924:u16)  [unwired: 2 in, 2 out]
            n507 = property on="ActiveMotor" class="Ring (strict)"() -> ("Strings []"=w926:string[])  [unwired: 2 in, 2 out]
            n508 = Build Array(w943, w944, w945, w938, w937, w936, w935, w934, w933, w932, w931, w930) -> (w929:u16[])
            n509 = Increment(x=w929) -> (x+1=w928:u16[])
            n510 = Index Array(array=w926, index=w924) -> (element=w925:string)
            n511 = for {
              tunnel: w928 -> [w960] mode=indexing
              tunnel: w941 -> [w955]
              tunnel: [w951] -> w927 mode=indexing
              tunnel: [w950] -> w923 mode=indexing
              tunnel: [w949] -> w922 mode=indexing
              n512 = Multiply(x=w960, y=u16 3) -> (x*y=w956:u16)
              n513 = Subtract(x=w956, y=u16 3) -> (x-y=w950:u16)
              n514 = Subtract(x=w956, y=u16 2) -> (x-y=w949:u16)
              n515 = Index Array(array=w955, index=w950) -> (element=w954:refnum<vi>)
              n516 = Index Array(array=w955, index=w949) -> (element=w953:refnum<vi>)
              n517 = Bundle By Name(cluster="active Axis ref", "Ref X"=w954, "Ref Y"=w953) -> (w951:cluster{"Ref X":refnum<vi>, "Ref Y":refnum<vi>})
            }
            "Array" <- w923
            "Array 2" <- w922
            n518 = property on="ActiveMotorName::99" class="Str"("Val(Sgnl)"=w925) -> ()  [unwired: 2 in, 2 out]
            n519 = call <vilib>:"Add State(s) to Queue__jki_lib_state_machine.vi"("State(s) in (\"\")"=w948) -> ("States Out"=w947:string)  [unwired: 14 in]
            n520 = Bundle By Name(cluster=w940, "active axis refs 2"=w927) -> (w939:T36)
          }
          frame "Move Config" {
            # "Your code here.\n(You can make a copy of, or modify, this frame)"
            n521 = Unbundle By Name(w962) -> ("move properties"=w966:T2[], "active ccd"=w965:i32)
            n522 = Replace Array Subset(array=w966, new element="move config", index=w965) -> (w963:T2[])
            n523 = Bundle By Name(cluster=w962, "move properties"=w963) -> (w961:T36)
            n524 = call <vilib>:"Add State(s) to Queue__jki_lib_state_machine.vi"("State(s) in (\"\")"=w969) -> ("States Out"=w968:string)  [unwired: 14 in]
          }
          frame "----------Centroid & Move----------" {
            # "Template Separator\n(You can make a copy of, or modify, this frame)"
            n525 = call <vilib>:"Add State(s) to Queue__jki_lib_state_machine.vi"("State(s) in (\"\")"=w973) -> ("States Out"=w972:string)  [unwired: 14 in]
          }
          frame "detected" {
            n526 = Unbundle By Name(w976) -> ("Offset X"=w1018:dbl[][], "Offset Y"=w1017:dbl[][], "Size"=w1016:dbl[][], "Mean Size"=w1015:dbl[][], "Time"=w1012:timestamp[][], "Motor X"=w990:dbl[][], "active axis refs 2"=w989:T12, "Motor Y"=w988:dbl[][])
            n527 = Spreadsheet String To Array(format string="%s", spreadsheet string=w994, array type (2D Dbl)=string[] []) -> (array=w983:string[])  [unwired: 1 in]
            n528 = call-poly <userlib>:"Filter 1D Array__ogtk.vi"("items to filter"=w983, "array"=w984) -> ("filtered item indices"=w981:i32[])  [unwired: 4 in, 1 out]
            n529 = for {
              tunnel: w984 -> [w1035] mode=indexing
              tunnel: w983 -> [w1034]
              tunnel: [w1032] -> w985 mode=indexing
              n530 = for {
                tunnel: w1035 -> [w1038]
                tunnel: [w1037] -> w1033 mode=indexing
                tunnel: w1034 -> [w1036] mode=indexing
                n531 = Equal?(x=w1038, y=w1036) -> (x = y?=w1037:bool)
              }
              n532 = Or Array Elements(Boolean array=w1033) -> (logical OR=w1032:bool)
            }
            n533 = for {
              N: 12 -> [_]
              tunnel: w981 -> [w1031]
              tunnel: [w1028] -> w980 mode=indexing
              i -> [w1030]
              n534 = Equal?(x=w1031, y=w1030) -> (x = y?=w1029:bool[])
              n535 = Or Array Elements(Boolean array=w1029) -> (logical OR=w1028:bool)
            }
            "Array 3" <- w980
            n536 = call <vilib>:"Build State String with Arguments__jki_lib_state_machine.vi"("Arguments (\"\")"=w994, "State"="stats") -> ("State with Arguments"=w993:string)  [unwired: 4 in]
            n537 = Unbundle By Name(w976) -> ("Mean Centroid X"=w1023:dbl[][], "Mean Centroid Y"=w1022:dbl[][], "Centroid X"=w1025:dbl[][], "Centroid Y"=w1024:dbl[][])
            n538 = call <vilib>:"Add State(s) to Queue__jki_lib_state_machine.vi"("State(s) in (\"\")"=w992, "State(s) at Back (\"\")"=w993) -> ("States Out"=w991:string)  [unwired: 13 in]
            n539 = for {
              tunnel: w1025 -> [w1088]
              tunnel: w1024 -> [w1087]
              tunnel: w1023 -> [w1086]
              tunnel: w1022 -> [w1085]
              tunnel: [w1084] -> w1009 mode=indexing
              tunnel: [w1083] -> w1020 mode=indexing
              tunnel: w1019 -> [w1056] mode=indexing
              tunnel: w1018 -> [w1082]
              tunnel: w1017 -> [w1081]
              tunnel: [w1080] -> w997 mode=indexing
              tunnel: [w1079] -> w1010 mode=indexing
              tunnel: w1016 -> [w1078]
              tunnel: w1015 -> [w1077]
              tunnel: [w1076] -> w1014 mode=indexing
              tunnel: w1012 -> [w1075]
              tunnel: [w1074] -> w1011 mode=indexing
              tunnel: w990 -> [w1048]
              tunnel: w989 -> [w1047]
              tunnel: w988 -> [w1046]
              tunnel: [w1045] -> w987 mode=indexing
              tunnel: [w1044] -> w986 mode=indexing
              tunnel: w985 -> [w1043]
              i -> [w1042]
              n540 = Unbundle By Name(w1056) -> ("Target.X::12"=w1059:refnum<vi>, "Target.Y::12"=w1058:refnum<vi>)
              n541 = Index Array(array=w1048, index (row)=w1042) -> (element=w1051:dbl[])  [unwired: 1 in]
              n542 = Index Array(array=w1047, index=w1042) -> (element=w1050:cluster{"Ref X":refnum<vi>, "Ref Y":refnum<vi>})
              n543 = Index Array(array=w1046, index (row)=w1042) -> (element=w1055:dbl[])  [unwired: 1 in]
              n544 = Index Array(array=w1086, index (row)=w1042) -> (element=w1070:dbl[])  [unwired: 1 in]
              n545 = Index Array(array=w1085, index (row)=w1042) -> (element=w1071:dbl[])  [unwired: 1 in]
              n546 = Index Array(array=w1088, index (row)=w1042) -> (element=w1073:dbl[])  [unwired: 1 in]
              n547 = Index Array(array=w1087, index (row)=w1042) -> (element=w1072:dbl[])  [unwired: 1 in]
              n548 = Index Array(array=w1082, index (row)=w1042) -> (element=w1067:dbl[])  [unwired: 1 in]
              n549 = Index Array(array=w1081, index (row)=w1042) -> (element=w1066:dbl[])  [unwired: 1 in]
              n550 = Index Array(array=w1078, index (row)=w1042) -> (element=w1064:dbl[])  [unwired: 1 in]
              n551 = Index Array(array=w1077, index (row)=w1042) -> (element=w1063:dbl[])  [unwired: 1 in]
              n552 = Index Array(array=w1075, index (row)=w1042) -> (element=w1060:timestamp[])  [unwired: 1 in]
              n553 = Index Array(array=w1043, index=w1042) -> (element=w1041:bool)
              n554 = Unbundle By Name(w1050) -> ("Ref X"=w1049:refnum<vi>, "Ref Y"=w1053:refnum<vi>)
              n555 = property class="DigNum (strict)"(reference=w1059) -> ("Value"=w1040:dbl)  [unwired: 1 in, 2 out]
              n556 = property class="DigNum (strict)"(reference=w1058) -> ("Value"=w1057:dbl)  [unwired: 1 in, 2 out]
              n557 = call <vilib>:"Std Deviation and Variance.vi"("X"=w1073) -> ("mean"=w1039:dbl)  [unwired: 1 in, 2 out]
              n558 = call <vilib>:"Std Deviation and Variance.vi"("X"=w1072) -> ("mean"=w1069:dbl)  [unwired: 1 in, 2 out]
              n559 = call <vilib>:"Std Deviation and Variance.vi"("X"=w1064) -> ("mean"=w1062:dbl)  [unwired: 1 in, 2 out]
              n560 = Get Date/Time In Seconds() -> (seconds since 1Jan1904=w1061:timestamp)
              n561 = property class="DigNum (strict)"(reference=w1049) -> ("Value"=w1052:dbl)  [unwired: 1 in, 2 out]
              n562 = property class="DigNum (strict)"(reference=w1053) -> ("Value"=w1054:dbl)  [unwired: 1 in, 2 out]
              n563 = Subtract(x=w1040, y=w1039) -> (x-y=w1068:dbl)
              n564 = Subtract(x=w1057, y=w1069) -> (x-y=w1065:dbl)
              n565 = case shown="True" w1041 {
                tunnel: [w1106 w1120] -> w1084
                tunnel: [w1105 w1119] -> w1083
                tunnel: [w1104 w1118] -> w1080
                tunnel: [w1103 w1117] -> w1079
                tunnel: [w1102 w1116] -> w1076
                tunnel: [w1101 w1115] -> w1074
                tunnel: w1071 -> [w1100 w1114]
                tunnel: w1070 -> [w1099 w1113]
                tunnel: w1039 -> [w1098 _]
                tunnel: w1069 -> [w1097 _]
                tunnel: w1068 -> [w1096 _]
                tunnel: w1067 -> [w1095 w1112]
                tunnel: w1066 -> [w1094 w1111]
                tunnel: w1065 -> [w1093 _]
                tunnel: w1063 -> [w1092 w1110]
                tunnel: w1062 -> [w1091 _]
                tunnel: w1061 -> [w1090 w1109]
                tunnel: w1060 -> [w1089 w1108]
                frame True {
                  n566 = Build Array (concatenate)(w1099, w1098) -> (w1106:dbl[])
                  n567 = Build Array (concatenate)(w1100, w1097) -> (w1105:dbl[])
                  n568 = Build Array (concatenate)(w1095, w1096) -> (w1104:dbl[])
                  n569 = Build Array (concatenate)(w1094, w1093) -> (w1103:dbl[])
                  n570 = Build Array (concatenate)(w1092, w1091) -> (w1102:dbl[])
                  n571 = Build Array (concatenate)(w1089, w1090) -> (w1101:timestamp[])
                }
                frame False {
                  w1107 = 0.0
                  n572 = Build Array (concatenate)(w1113, w1107) -> (w1120:dbl[])
                  n573 = Build Array (concatenate)(w1114, w1107) -> (w1119:dbl[])
                  n574 = Build Array (concatenate)(w1112, w1107) -> (w1118:dbl[])
                  n575 = Build Array (concatenate)(w1111, w1107) -> (w1117:dbl[])
                  n576 = Build Array (concatenate)(w1110, w1107) -> (w1116:dbl[])
                  n577 = Build Array (concatenate)(w1108, w1109) -> (w1115:timestamp[])
                }
              }
              n578 = Build Array (concatenate)(w1055, w1054) -> (w1044:dbl[])
              n579 = Build Array (concatenate)(w1051, w1052) -> (w1045:dbl[])
            }
            n580 = local write "Numeric"(0.0 ("Numeric")) -> ()
            n581 = Array Size(array=w997) -> (size(s)=w1008:i32[])
            n582 = Index Array(array=w1008, index=1) -> (element=w1006:i32)
            "History index" <- w1006
            n583 = call <vilib>:"Add State(s) to Queue__jki_lib_state_machine.vi"("State(s) in (\"\")"=w991, "State(s) at Back (\"\")"="Check Move\ntdms" ("State(s) at Back (\"\")")) -> ("States Out"=w1000:string)  [unwired: 13 in]
            n584 = Unbundle By Name(w976) -> ("img to avg"=w975:i32)
            n585 = Decrement(x=w975) -> (x-1=w974:i32)
            n586 = Initialize Array(0.0 ("element"), 12 ("dimension size"), w974) -> (w977:dbl[][])
            n587 = Greater?(x=w1006, y="History Size") -> (0:w1004:bool)
            n588 = Bundle By Name(cluster=w976, "Centroid X"=w977, "Centroid Y"=w977, "Mean Centroid X"=w1009, "Mean Centroid Y"=w1020, "Offset X"=w997, "Offset Y"=w1010, "Mean Size"=w1014, "Size"=w977, "Time"=w1011, "Motor X"=w987, "Motor Y"=w986) -> (w1021:T36)
            n589 = Select(t="history" ("State(s) at Back (\"\")"), s=w1004, f="") -> (s? t:f=w1001:string)
            n590 = call <vilib>:"Add State(s) to Queue__jki_lib_state_machine.vi"("State(s) in (\"\")"=w1000, "State(s) at Back (\"\")"=w1001) -> ("States Out"=w999:string)  [unwired: 13 in]
          }
          frame "Check Move" {
            (unwired) "Device Ini" ("State(s) in Front (\"\")")
            # "Your code here.\n(You can make a copy of, or modify, this frame)"
            n591 = Unbundle By Name(w1125) -> ("move properties"=w1128:T2[], "Mean Size"=w1151:dbl[][], "move properties"=w1154:T2[], "Offset X"=w1153:dbl[][], "Offset Y"=w1152:dbl[][], "active cams"=w1132:string[])
            n592 = for {
              tunnel: w1154 -> [w1219]
              tunnel: w1153 -> [w1218]
              tunnel: w1152 -> [w1217]
              tunnel: w1151 -> [w1220]
              tunnel: [w1236] -> w1150 mode=indexing
              tunnel: [w1232] -> w1149 mode=indexing
              tunnel: w1132 -> [w1222] mode=indexing
              tunnel: [w1254] -> w1148 mode=indexing
              tunnel: [w1253] -> w1147 mode=indexing
              tunnel: w1128 -> [w1212]
              tunnel: [w1230] -> w1126 mode=indexing
              tunnel: [w1225] -> w1122 mode=indexing
              tunnel: "Speedmode @" -> [w1224]
              tunnel: w1121 -> [w1223]
              n593 = call-poly <userlib>:"Filter 1D Array__ogtk.vi"("items to filter"=w1222, "array"=w1223) -> ("filtered item indices"=w1221:i32[])  [unwired: 4 in, 1 out]
              n594 = Index Array(array=w1221) -> (element=w1211:i32)  [unwired: 1 in]
              n595 = Index Array(array=w1220, index (row)=w1211) -> (element=w1216:dbl[])  [unwired: 1 in]
              n596 = Index Array(array=w1219, index=w1211) -> (element=w1215:T2)
              n597 = Index Array(array=w1218, index (row)=w1211) -> (element=w1214:dbl[])  [unwired: 1 in]
              n598 = Index Array(array=w1212, index=w1211) -> (element=w1210:T2)
              n599 = Index Array(array=w1217, index (row)=w1211) -> (element=w1213:dbl[])  [unwired: 1 in]
              n600 = Unbundle By Name(w1215) -> ("Tolerance [%]"=w1247:dbl)
              n601 = Reverse 1D Array(array=w1214) -> (reversed array=w1252:dbl[])
              n602 = Reverse 1D Array(array=w1213) -> (reversed array=w1251:dbl[])
              n603 = Reverse 1D Array(array=w1216) -> (reversed array=w1246:dbl[])
              n604 = Unbundle By Name(w1210) -> ("enable feedback"=w1235:bool)
              n605 = Index Array(array=w1252) -> (element=w1250:dbl)  [unwired: 1 in]
              n606 = Index Array(array=w1251) -> (element=w1249:dbl)  [unwired: 1 in]
              n607 = Index Array(array=w1246) -> (element=w1245:dbl)  [unwired: 1 in]
              n608 = Absolute Value(x=w1250) -> (abs(x)=w1231:dbl)
              n609 = Absolute Value(x=w1249) -> (abs(x)=w1228:dbl)
              n610 = Square Root(x=w1245) -> (sqrt(x)=w1244:dbl)
              n611 = Divide(x=w1247, y=100.0) -> (x/y=w1243:dbl)
              n612 = Multiply(x=w1244, y=w1243) -> (x*y=w1227:dbl)
              n613 = Not Equal To 0?(x=w1228) -> (x != 0?=w1233:bool)
              n614 = Not Equal To 0?(x=w1231) -> (x != 0?=w1238:bool)
              n615 = Greater Or Equal?(x=w1231, y=w1227) -> (x >= y?=w1237:bool)
              n616 = Greater Or Equal?(x=w1228, y=w1227) -> (x >= y?=w1234:bool)
              n617 = Divide(x=w1231, y=w1227) -> (x/y=w1229:dbl)
              n618 = Divide(x=w1228, y=w1227) -> (x/y=w1226:dbl)
              n619 = Compound Arithmetic op=AND(w1235, w1238, w1237) -> (w1236:bool)
              n620 = Compound Arithmetic op=AND(w1235, w1234, w1233) -> (w1232:bool)
              n621 = Boolean To (0,1)(Boolean=w1232) -> (0, 1=w1239:i16)
              n622 = Greater?(x=w1229, y=w1224) -> (0:w1230:bool)
              n623 = Greater?(x=w1226, y=w1224) -> (0:w1225:bool)
              n624 = Multiply(x=w1239, y=w1228) -> (x*y=w1240:dbl)
              n625 = Boolean To (0,1)(Boolean=w1236) -> (0, 1=w1242:i16)
              n626 = Multiply(x=w1242, y=w1231) -> (x*y=w1241:dbl)
              n627 = Bundle(w1240, "GUIdevice 8"=w1222) -> (w1253:cluster{dbl, "GUIdevice 8":string})  [unwired: 1 in]
              n628 = Bundle(w1241, "GUIdevice 8"=w1222) -> (w1254:cluster{dbl, "GUIdevice 8":string})  [unwired: 1 in]
            }
            "required X" <- w1150
            "required Y" <- w1149
            "speedmode X" <- w1126
            "speedmode Y" <- w1122
            n629 = case shown="True" "Align" {
              tunnel: w1148 -> [w1162 w1167]
              tunnel: w1147 -> [w1161 w1164]
              tunnel: [w1160 w1166] -> w1144
              tunnel: [w1159 w1163] -> w1138
              frame False {
                n630 = Sort 1D Array(array=w1161) -> (sorted array=w1158:cluster{dbl, "GUIdevice 8":string}[])
                n631 = Sort 1D Array(array=w1162) -> (sorted array=w1157:cluster{dbl, "GUIdevice 8":string}[])
                n632 = Reverse 1D Array(array=w1158) -> (reversed array=w1159:cluster{dbl, "GUIdevice 8":string}[])
                n633 = Reverse 1D Array(array=w1157) -> (reversed array=w1160:cluster{dbl, "GUIdevice 8":string}[])
              }
              frame True {
                w1165 = cluster{dbl, "GUIdevice 8":string}[] [] ("Array")
                n634 = for {
                  shift-right: [w1177] -> w1166
                  shift-left: w1165 -> [w1179]
                  tunnel: w1167 -> [w1178] mode=indexing
                  n635 = Unbundle(w1178) -> (w1181:dbl)  [unwired: 1 out]
                  n636 = Not Equal To 0?(x=w1181) -> (x != 0?=w1180:bool)
                  n637 = case shown="True" w1180 {
                    tunnel: w1179 -> [w1182 w1185]
                    tunnel: w1178 -> [_ w1184]
                    tunnel: [w1182 w1183] -> w1177
                    frame False {
                    }
                    frame True {
                      n638 = Build Array (concatenate)(w1185, w1184) -> (w1183:cluster{dbl, "GUIdevice 8":string}[])
                    }
                  }
                }
                n639 = for {
                  shift-right: [w1168] -> w1163
                  shift-left: w1165 -> [w1170]
                  tunnel: w1164 -> [w1169] mode=indexing
                  n640 = Unbundle(w1169) -> (w1172:dbl)  [unwired: 1 out]
                  n641 = Not Equal To 0?(x=w1172) -> (x != 0?=w1171:bool)
                  n642 = case shown="True" w1171 {
                    tunnel: w1170 -> [w1173 w1176]
                    tunnel: w1169 -> [_ w1175]
                    tunnel: [w1173 w1174] -> w1168
                    frame False {
                    }
                    frame True {
                      n643 = Build Array (concatenate)(w1176, w1175) -> (w1174:cluster{dbl, "GUIdevice 8":string}[])
                    }
                  }
                }
              }
            }
            n644 = call <vilib>:"Add State(s) to Queue__jki_lib_state_machine.vi"("State(s) in (\"\")"=w1131) -> ("States Out"=w1130:string)  [unwired: 14 in]
            n645 = Bundle By Name(cluster=w1125, "speedmode X"=w1126, "speedmode Y"=w1122) -> (w1124:T36)
            n646 = Empty Array?(array=w1144) -> (empty?=w1141:bool)
            n647 = Empty Array?(array=w1138) -> (empty?=w1136:bool)
            n648 = Index Array(array=w1144) -> (element=w1134:cluster{dbl, "GUIdevice 8":string})  [unwired: 1 in]
            n649 = Index Array(array=w1138) -> (element=w1133:cluster{dbl, "GUIdevice 8":string})  [unwired: 1 in]
            n650 = Unbundle(w1134) -> (w1143:dbl)  [unwired: 1 out]
            n651 = Unbundle(w1133) -> (w1139:dbl)  [unwired: 1 out]
            n652 = Equal To 0?(x=w1143) -> (x = 0?=w1142:bool)
            n653 = Equal To 0?(x=w1139) -> (x = 0?=w1137:bool)
            n654 = property on="autodetect" class="Bool (strict)"("Value"=FALSE ("autodetect")) -> ()  [unwired: 2 in, 2 out]
            n655 = Unbundle By Name(w1124) -> ("Feedback global"=w1145:bool)
            n656 = Or(x=w1142, y=w1141) -> (x .or. y?=w1140:bool)
            n657 = Or(x=w1137, y=w1136) -> (x .or. y?=w1135:bool)
            n658 = case shown="True" w1145 {
              tunnel: w1140 -> [_ w1193]
              tunnel: w1144 -> [_ w1192]
              tunnel: w1135 -> [_ w1190]
              tunnel: w1138 -> [_ w1189]
              tunnel: w1130 -> [w1186 w1188]
              tunnel: [w1186 w1187] -> w1146
              frame False {
              }
              frame True {
                n659 = case shown="False" w1193 {
                  tunnel: w1192 -> [w1208 _]
                  tunnel: w1188 -> [w1204 w1209]
                  tunnel: [w1202 w1209] -> w1191
                  frame False {
                    n660 = Index Array(array=w1208) -> (element=w1207:cluster{dbl, "GUIdevice 8":string})  [unwired: 1 in]
                    n661 = Unbundle By Name(w1207) -> ("GUIdevice 8"=w1206:string)
                    n662 = call <vilib>:"Build State String with Arguments__jki_lib_state_machine.vi"("Arguments (\"\")"=w1206, "State"="Move X") -> ("State with Arguments"=w1203:string)  [unwired: 4 in]
                    n663 = call <vilib>:"Add State(s) to Queue__jki_lib_state_machine.vi"("State(s) in (\"\")"=w1204, "State(s) at Back (\"\")"=w1203) -> ("States Out"=w1202:string)  [unwired: 13 in]
                  }
                  frame True {
                  }
                }
                n664 = case shown="False" w1190 {
                  tunnel: w1189 -> [w1200 _]
                  tunnel: w1191 -> [w1196 w1201]
                  tunnel: [w1194 w1201] -> w1187
                  frame False {
                    n665 = Index Array(array=w1200) -> (element=w1199:cluster{dbl, "GUIdevice 8":string})  [unwired: 1 in]
                    n666 = Unbundle By Name(w1199) -> ("GUIdevice 8"=w1198:string)
                    n667 = call <vilib>:"Build State String with Arguments__jki_lib_state_machine.vi"("Arguments (\"\")"=w1198, "State"="Move Y") -> ("State with Arguments"=w1195:string)  [unwired: 4 in]
                    n668 = call <vilib>:"Add State(s) to Queue__jki_lib_state_machine.vi"("State(s) in (\"\")"=w1196, "State(s) at Back (\"\")"=w1195) -> ("States Out"=w1194:string)  [unwired: 13 in]
                  }
                  frame True {
                  }
                }
              }
            }
            n669 = call <vilib>:"Add State(s) to Queue__jki_lib_state_machine.vi"("State(s) in (\"\")"=w1130, "State(s) at Back (\"\")"=w1146) -> ("States Out"=w1156:string)  [unwired: 13 in]
          }
          frame "Move X" {
            # "Your code here.\n(You can make a copy of, or modify, this frame)"
            n670 = Unbundle By Name(w1278) -> ("Offset X"=w1255:dbl[][])
            n671 = call-poly <userlib>:"Filter 1D Array__ogtk.vi"("items to filter"=w1263, "array"=w1282) -> ("filtered item indices"=w1267:i32[])  [unwired: 4 in, 1 out]
            n672 = Unbundle By Name(w1278) -> ("speedmode X"=w1262:bool[], "active axis refs 2"=w1281:T12, "move properties"=w1266:T2[])
            n673 = for {
              tunnel: w1267 -> [w1287] mode=indexing
              tunnel: w1266 -> [w1291]
              shift-right: [w1286] -> w1264
              shift-left: i32[] [] ("filtered item indices") -> [w1289]
              n674 = Index Array(array=w1291, index=w1287) -> (element=w1290:T2)
              n675 = Unbundle By Name(w1290) -> ("enable feedback"=w1288:bool)
              n676 = case shown="True" w1288 {
                tunnel: w1289 -> [w1292 w1295]
                tunnel: w1287 -> [_ w1294]
                tunnel: [w1292 w1293] -> w1286
                frame False {
                }
                frame True {
                  n677 = Build Array (concatenate)(w1295, w1294) -> (w1293:i32[])
                }
              }
            }
            n678 = Index Array(array=w1264) -> (element=w1261:i32)  [unwired: 1 in]
            n679 = Index Array(array=w1255, index (row)=w1261) -> (element=w1277:dbl[])  [unwired: 1 in]
            n680 = Reverse 1D Array(array=w1277) -> (reversed array=w1276:dbl[])
            n681 = Index Array(array=w1281, index=w1261) -> (element=w1280:cluster{"Ref X":refnum<vi>, "Ref Y":refnum<vi>})
            n682 = Index Array(array=w1276) -> (element=w1274:dbl)  [unwired: 1 in]
            n683 = Index Array(array=w1266, index=w1261) -> (element=w1279:T2)
            n684 = Unbundle By Name(w1280) -> ("Ref X"=w1271:refnum<vi>, "Ref Y"=w1270:refnum<vi>)
            n685 = Index Array(array=w1262, index=w1261) -> (element=w1260:bool)
            n686 = Unbundle By Name(w1279) -> ("Invert Direction X"=w1272:bool, "Invert Axis"=w1275:bool, "Stepsize"=w1258:dbl, "enable feedback"=w1269:bool)
            n687 = Greater Or Equal To 0?(x=w1274) -> (x >= 0?=w1273:bool)
            n688 = call <vilib>:"Add State(s) to Queue__jki_lib_state_machine.vi"("State(s) in Front (\"\")"="Wait" ("State(s) in Front (\"\")"), "State(s) in (\"\")"=w1285) -> ("States Out"=w1284:string)  [unwired: 13 in]
            n689 = property on="Speedmode @" class="DigNum (strict)"() -> ("Value"=w1257:dbl)  [unwired: 2 in, 2 out]
            n690 = Multiply(x=w1257, y=w1258) -> (x*y=w1259:dbl)
            n691 = Select(t=w1259, s=w1260, f=w1258) -> (s? t:f=w1256:dbl)
            n692 = case shown="True" w1269 {
              tunnel: w1275 -> [_ w1301]
              tunnel: w1273 -> [_ w1300]
              tunnel: w1256 -> [_ w1299]
              tunnel: w1272 -> [_ w1298]
              tunnel: w1271 -> [_ w1297]
              tunnel: w1270 -> [_ w1296]
              frame False {
              }
              frame True {
                n693 = case shown="False" w1300 {
                  tunnel: w1298 -> [w1309 w1331]
                  tunnel: w1299 -> [w1307 w1329]
                  tunnel: w1301 -> [w1306 w1328]
                  tunnel: w1301 -> [w1305 w1327]
                  tunnel: w1297 -> [w1303 w1325]
                  tunnel: w1296 -> [w1302 w1324]
                  frame True {
                    n694 = case shown="False" w1306 {
                      tunnel: [w1320 w1322] -> w1308
                      tunnel: w1303 -> [w1321 _]
                      tunnel: w1302 -> [_ w1323]
                      frame False {
                        n695 = property class="DigNum (strict)"(reference=w1321) -> ("Value"=w1320:dbl)  [unwired: 1 in, 2 out]
                      }
                      frame True {
                        n696 = property class="DigNum (strict)"(reference=w1323) -> ("Value"=w1322:dbl)  [unwired: 1 in, 2 out]
                      }
                    }
                    n697 = case shown="False" w1309 {
                      tunnel: w1308 -> [w1316 w1319]
                      tunnel: w1307 -> [w1315 w1318]
                      tunnel: [w1314 w1317] -> w1304
                      frame False {
                        n698 = Add(x=w1316, y=w1315) -> (x+y=w1314:dbl)
                      }
                      frame True {
                        n699 = Subtract(x=w1319, y=w1318) -> (x-y=w1317:dbl)
                      }
                    }
                    n700 = case shown="False" w1305 {
                      tunnel: w1304 -> [w1310 w1312]
                      tunnel: w1303 -> [w1311 _]
                      tunnel: w1302 -> [_ w1313]
                      frame False {
                        n701 = property class="DigNum (strict)"(reference=w1311, "Val(Sgnl)"=w1310) -> ()  [unwired: 1 in, 2 out]
                      }
                      frame True {
                        n702 = property class="DigNum (strict)"(reference=w1313, "Val(Sgnl)"=w1312) -> ()  [unwired: 1 in, 2 out]
                      }
                    }
                  }
                  frame False {
                    n703 = case shown="False" w1328 {
                      tunnel: [w1342 w1344] -> w1330
                      tunnel: w1325 -> [w1343 _]
                      tunnel: w1324 -> [_ w1345]
                      frame False {
                        n704 = property class="DigNum (strict)"(reference=w1343) -> ("Value"=w1342:dbl)  [unwired: 1 in, 2 out]
                      }
                      frame True {
                        n705 = property class="DigNum (strict)"(reference=w1345) -> ("Value"=w1344:dbl)  [unwired: 1 in, 2 out]
                      }
                    }
                    n706 = case shown="False" w1331 {
                      tunnel: w1330 -> [w1338 w1341]
                      tunnel: w1329 -> [w1337 w1340]
                      tunnel: [w1336 w1339] -> w1326
                      frame False {
                        n707 = Subtract(x=w1338, y=w1337) -> (x-y=w1336:dbl)
                      }
                      frame True {
                        n708 = Add(x=w1341, y=w1340) -> (x+y=w1339:dbl)
                      }
                    }
                    n709 = case shown="False" w1327 {
                      tunnel: w1326 -> [w1332 w1334]
                      tunnel: w1325 -> [w1333 _]
                      tunnel: w1324 -> [_ w1335]
                      frame False {
                        n710 = property class="DigNum (strict)"(reference=w1333, "Val(Sgnl)"=w1332) -> ()  [unwired: 1 in, 2 out]
                      }
                      frame True {
                        n711 = property class="DigNum (strict)"(reference=w1335, "Val(Sgnl)"=w1334) -> ()  [unwired: 1 in, 2 out]
                      }
                    }
                  }
                }
              }
            }
            "Arguments X" <- w1263
            "Moving X" <- w1263
          }
          frame "Move Y" {
            # "Your code here.\n(You can make a copy of, or modify, this frame)"
            n712 = Unbundle By Name(w1369) -> ("Offset Y"=w1368:dbl[][])
            n713 = call-poly <userlib>:"Filter 1D Array__ogtk.vi"("items to filter"=w1353, "array"=w1373) -> ("filtered item indices"=w1358:i32[])  [unwired: 4 in, 1 out]
            n714 = Unbundle By Name(w1369) -> ("speedmode Y"=w1352:bool[], "active axis refs 2"=w1372:T12, "move properties"=w1356:T2[])
            n715 = for {
              tunnel: w1358 -> [w1378] mode=indexing
              tunnel: w1356 -> [w1382]
              shift-right: [w1377] -> w1357
              shift-left: i32[] [] ("filtered item indices") -> [w1380]
              n716 = Index Array(array=w1382, index=w1378) -> (element=w1381:T2)
              n717 = Unbundle By Name(w1381) -> ("enable feedback"=w1379:bool)
              n718 = case shown="True" w1379 {
                tunnel: w1380 -> [w1383 w1386]
                tunnel: w1378 -> [_ w1385]
                tunnel: [w1383 w1384] -> w1377
                frame False {
                }
                frame True {
                  n719 = Build Array (concatenate)(w1386, w1385) -> (w1384:i32[])
                }
              }
            }
            n720 = Index Array(array=w1357) -> (element=w1351:i32)  [unwired: 1 in]
            n721 = Index Array(array=w1368, index (row)=w1351) -> (element=w1367:dbl[])  [unwired: 1 in]
            n722 = Reverse 1D Array(array=w1367) -> (reversed array=w1366:dbl[])
            n723 = Index Array(array=w1372, index=w1351) -> (element=w1371:cluster{"Ref X":refnum<vi>, "Ref Y":refnum<vi>})
            n724 = Index Array(array=w1366) -> (element=w1364:dbl)  [unwired: 1 in]
            n725 = Index Array(array=w1356, index=w1351) -> (element=w1370:T2)
            n726 = Index Array(array=w1352, index=w1351) -> (element=w1350:bool)
            n727 = Unbundle By Name(w1371) -> ("Ref Y"=w1361:refnum<vi>, "Ref X"=w1360:refnum<vi>)
            n728 = Unbundle By Name(w1370) -> ("Invert Direction Y"=w1362:bool, "Invert Axis"=w1365:bool, "Stepsize"=w1348:dbl, "enable feedback"=w1359:bool)
            n729 = Greater Or Equal To 0?(x=w1364) -> (x >= 0?=w1363:bool)
            n730 = call <vilib>:"Add State(s) to Queue__jki_lib_state_machine.vi"("State(s) in Front (\"\")"="Wait" ("State(s) in Front (\"\")"), "State(s) in (\"\")"=w1376) -> ("States Out"=w1375:string)  [unwired: 13 in]
            n731 = property on="Speedmode @" class="DigNum (strict)"() -> ("Value"=w1347:dbl)  [unwired: 2 in, 2 out]
            n732 = Multiply(x=w1347, y=w1348) -> (x*y=w1346:dbl)
            n733 = Select(t=w1346, s=w1350, f=w1348) -> (s? t:f=w1349:dbl)
            n734 = case shown="True" w1359 {
              tunnel: w1365 -> [_ w1392]
              tunnel: w1363 -> [_ w1391]
              tunnel: w1349 -> [_ w1390]
              tunnel: w1362 -> [_ w1389]
              tunnel: w1361 -> [_ w1388]
              tunnel: w1360 -> [_ w1387]
              frame False {
              }
              frame True {
                n735 = case shown="True" w1391 {
                  tunnel: w1389 -> [w1400 w1422]
                  tunnel: w1390 -> [w1398 w1420]
                  tunnel: w1392 -> [w1397 w1419]
                  tunnel: w1392 -> [w1396 w1418]
                  tunnel: w1388 -> [w1394 w1416]
                  tunnel: w1387 -> [w1393 w1415]
                  frame True {
                    n736 = case shown="False" w1397 {
                      tunnel: [w1411 w1413] -> w1399
                      tunnel: w1394 -> [w1412 _]
                      tunnel: w1393 -> [_ w1414]
                      frame False {
                        n737 = property class="DigNum (strict)"(reference=w1412) -> ("Value"=w1411:dbl)  [unwired: 1 in, 2 out]
                      }
                      frame True {
                        n738 = property class="DigNum (strict)"(reference=w1414) -> ("Value"=w1413:dbl)  [unwired: 1 in, 2 out]
                      }
                    }
                    n739 = case shown="False" w1400 {
                      tunnel: w1399 -> [w1407 w1410]
                      tunnel: w1398 -> [w1406 w1409]
                      tunnel: [w1405 w1408] -> w1395
                      frame False {
                        n740 = Add(x=w1407, y=w1406) -> (x+y=w1405:dbl)
                      }
                      frame True {
                        n741 = Subtract(x=w1410, y=w1409) -> (x-y=w1408:dbl)
                      }
                    }
                    n742 = case shown="False" w1396 {
                      tunnel: w1395 -> [w1401 w1403]
                      tunnel: w1394 -> [w1402 _]
                      tunnel: w1393 -> [_ w1404]
                      frame False {
                        n743 = property class="DigNum (strict)"(reference=w1402, "Val(Sgnl)"=w1401) -> ()  [unwired: 1 in, 2 out]
                      }
                      frame True {
                        n744 = property class="DigNum (strict)"(reference=w1404, "Val(Sgnl)"=w1403) -> ()  [unwired: 1 in, 2 out]
                      }
                    }
                  }
                  frame False {
                    n745 = case shown="False" w1419 {
                      tunnel: [w1433 w1435] -> w1421
                      tunnel: w1416 -> [w1434 _]
                      tunnel: w1415 -> [_ w1436]
                      frame False {
                        n746 = property class="DigNum (strict)"(reference=w1434) -> ("Value"=w1433:dbl)  [unwired: 1 in, 2 out]
                      }
                      frame True {
                        n747 = property class="DigNum (strict)"(reference=w1436) -> ("Value"=w1435:dbl)  [unwired: 1 in, 2 out]
                      }
                    }
                    n748 = case shown="False" w1422 {
                      tunnel: w1421 -> [w1429 w1432]
                      tunnel: w1420 -> [w1428 w1431]
                      tunnel: [w1427 w1430] -> w1417
                      frame False {
                        n749 = Subtract(x=w1429, y=w1428) -> (x-y=w1427:dbl)
                      }
                      frame True {
                        n750 = Add(x=w1432, y=w1431) -> (x+y=w1430:dbl)
                      }
                    }
                    n751 = case shown="False" w1418 {
                      tunnel: w1417 -> [w1423 w1425]
                      tunnel: w1416 -> [w1424 _]
                      tunnel: w1415 -> [_ w1426]
                      frame False {
                        n752 = property class="DigNum (strict)"(reference=w1424, "Val(Sgnl)"=w1423) -> ()  [unwired: 1 in, 2 out]
                      }
                      frame True {
                        n753 = property class="DigNum (strict)"(reference=w1426, "Val(Sgnl)"=w1425) -> ()  [unwired: 1 in, 2 out]
                      }
                    }
                  }
                }
              }
            }
            "Arguments Y" <- w1353
            "Moving Y" <- w1353
          }
          frame "Wait" {
            # "Your code here.\n(You can make a copy of, or modify, this frame)"
            n754 = flat-sequence {
              frame #0 {
                n755 = Wait (ms)(milliseconds to wait=u32 300) -> ()  [unwired: 1 out]
              }
              frame #1 {
                n756 = property on="Moving Y" class="Str"("Value"="") -> ()  [unwired: 2 in, 2 out]
                n757 = property on="Moving X" class="Str"("Value"="") -> ()  [unwired: 2 in, 2 out]
              }
            }
            n758 = call <vilib>:"Add State(s) to Queue__jki_lib_state_machine.vi"("State(s) in (\"\")"=w1442) -> ("States Out"=w1441:string)  [unwired: 14 in]
            n759 = local read "Mean Centroid X"() -> (w1437:dbl[][])
            n760 = Bundle By Name(cluster=w1439, "Mean Centroid X"=w1437, "Mean Centroid Y"=w1437) -> (w1438:T36)
          }
          frame "stats" {
            # "Your code here.\n(You can make a copy of, or modify, this frame)"
            n761 = Unbundle By Name(w1451) -> ("Offset X"=w1450:dbl[][], "Offset Y"=w1449:dbl[][], "Time"=w1448:timestamp[][], "Motor X"=w1447:dbl[][], "Motor Y"=w1446:dbl[][])
            n762 = for {
              tunnel: w1449 -> [w1489]
              tunnel: w1448 -> [w1490]
              tunnel: w1450 -> [w1491]
              tunnel: [w1494] -> w1477 mode=indexing
              tunnel: w1447 -> [w1488]
              tunnel: w1446 -> [w1487]
              tunnel: w1452 -> [_] mode=indexing
              i -> [w1481]
              n763 = Index Array(array=w1489, index (row)=w1481) -> (element=w1485:dbl[])  [unwired: 1 in]
              n764 = Index Array(array=w1488, index (row)=w1481) -> (element=w1483:dbl[])  [unwired: 1 in]
              n765 = Index Array(array=w1487, index (row)=w1481) -> (element=w1482:dbl[])  [unwired: 1 in]
              n766 = Index Array(array=w1491, index (row)=w1481) -> (element=w1486:dbl[])  [unwired: 1 in]
              n767 = Index Array(array=w1490, index (row)=w1481) -> (element=w1484:timestamp[])  [unwired: 1 in]
              n768 = Bundle("Time"=w1484, "Motor X"=w1483) -> (w1493:cluster{"Time":timestamp[], "Motor X":dbl[]})  [unwired: 1 in]
              n769 = Bundle("Time"=w1484, "Motor Y"=w1482) -> (w1492:cluster{"Time":timestamp[], "Motor Y":dbl[]})  [unwired: 1 in]
              n770 = Bundle("Time"=w1484, "Offset X"=w1486) -> (w1495:cluster{"Time":timestamp[], "Offset X":dbl[]})  [unwired: 1 in]
              n771 = Bundle("Time"=w1484, "Offset Y"=w1485) -> (w1496:cluster{"Time":timestamp[], "Offset Y":dbl[]})  [unwired: 1 in]
              n772 = Build Array(w1496, w1495, w1493, w1492) -> (w1494:cluster{"Time":timestamp[], "Motor Y":dbl[]}[])
            }
            n773 = call <vilib>:"Add State(s) to Queue__jki_lib_state_machine.vi"("State(s) in (\"\")"=w1480) -> ("States Out"=w1479:string)  [unwired: 14 in]
            n774 = Index Array(array=w1477, index (row) #1=0 ("index (row)"), index (row) #2=1 ("index (row)"), index (row) #3=2 ("index (row)"), index (row) #4=3 ("index (row)"), index (row) #5=4 ("index (row)"), index (row) #6=5 ("index (row)"), index (row) #7=6 ("index (row)"), index (row) #8=7 ("index (row)"), index (row) #9=8 ("index (row)"), index (row) #10=9 ("index (row)"), index (row) #11=10 ("index (row)"), index (row) #12=11 ("index (row)")) -> (element #1=→"CCD 1":cluster{"Time":timestamp[], "Motor Y":dbl[]}[], element #2=→"CCD 2":cluster{"Time":timestamp[], "Motor Y":dbl[]}[], element #3=→"CCD 3":cluster{"Time":timestamp[], "Motor Y":dbl[]}[], element #4=→"CCD 4":cluster{"Time":timestamp[], "Motor Y":dbl[]}[], element #5=→"CCD 5":cluster{"Time":timestamp[], "Motor Y":dbl[]}[], element #6=→"CCD 6":cluster{"Time":timestamp[], "Motor Y":dbl[]}[], element #7=→"CCD 7":cluster{"Time":timestamp[], "Motor Y":dbl[]}[], element #8=→"CCD 8":cluster{"Time":timestamp[], "Motor Y":dbl[]}[], element #9=→"CCD 9":cluster{"Time":timestamp[], "Motor Y":dbl[]}[], element #10=→"CCD 10":cluster{"Time":timestamp[], "Motor Y":dbl[]}[], element #11=→"CCD 11":cluster{"Time":timestamp[], "Motor Y":dbl[]}[], element #12=→"CCD 12":cluster{"Time":timestamp[], "Motor Y":dbl[]}[])  [unwired: 12 in]
          }
          frame "---------------Statistics--------------" {
            # "Template Separator\n(You can make a copy of, or modify, this frame)"
            n775 = call <vilib>:"Add State(s) to Queue__jki_lib_state_machine.vi"("State(s) in (\"\")"=w1500) -> ("States Out"=w1499:string)  [unwired: 14 in]
          }
          frame "Save Stats" {
            # "Your code here.\n(You can make a copy of, or modify, this frame)"
            n776 = property on="CCD 1" class="XYGraph (strict)"() -> ("Value"=w1510:cluster{timestamp[], dbl[]}[])  [unwired: 2 in, 2 out]
            n777 = property on="CCD 2" class="XYGraph (strict)"() -> ("Value"=w1509:cluster{timestamp[], dbl[]}[])  [unwired: 2 in, 2 out]
            n778 = property on="CCD 3" class="XYGraph (strict)"() -> ("Value"=w1508:cluster{timestamp[], dbl[]}[])  [unwired: 2 in, 2 out]
            n779 = property on="CCD 4" class="XYGraph (strict)"() -> ("Value"=w1507:cluster{timestamp[], dbl[]}[])  [unwired: 2 in, 2 out]
            n780 = property on="CCD 5" class="XYGraph (strict)"() -> ("Value"=w1506:cluster{timestamp[], dbl[]}[])  [unwired: 2 in, 2 out]
            n781 = property on="CCD 6" class="XYGraph (strict)"() -> ("Value"=w1505:cluster{timestamp[], dbl[]}[])  [unwired: 2 in, 2 out]
            n782 = property on="CCD 7" class="XYGraph (strict)"() -> ("Value"=w1504:cluster{timestamp[], dbl[]}[])  [unwired: 2 in, 2 out]
            n783 = property on="CCD 8" class="XYGraph (strict)"() -> ("Value"=w1503:cluster{timestamp[], dbl[]}[])  [unwired: 2 in, 2 out]
            n784 = Build Array(w1510, w1509, w1508, w1507, w1506, w1505, w1504, w1503) -> (w1502:cluster{timestamp[], dbl[]}[][])
            n785 = for {
              tunnel: w1502 -> [w1518] mode=indexing
              tunnel: w1501 -> [w1517] mode=indexing
              n786 = Empty String/Path?(string/path=w1517) -> (empty?=w1516:bool)
              n787 = case shown="False" w1516 {
                tunnel: w1518 -> [w1524 _]
                tunnel: w1517 -> [w1522 _]
                frame False {
                  n788 = Index Array(array=w1524, index #1=0 ("index"), index #2=1 ("index"), index #3=2 ("index"), index #4=3 ("index")) -> (element #1=w1559:cluster{timestamp[], dbl[]}, element #2=w1553:cluster{timestamp[], dbl[]}, element #3=w1552:cluster{timestamp[], dbl[]}, element #4=w1551:cluster{timestamp[], dbl[]})  [unwired: 1 in, 1 out]
                  n789 = Concatenate Strings(w1522, ".dat" ("string")) -> (w1520:string)
                  n790 = Unbundle(w1559) -> (w1558:timestamp[], w1536:dbl[])
                  n791 = Unbundle(w1553) -> (w1527:dbl[])  [unwired: 1 out]
                  n792 = Unbundle(w1552) -> (w1526:dbl[])  [unwired: 1 out]
                  n793 = Unbundle(w1551) -> (w1525:dbl[])  [unwired: 1 out]
                  n794 = Build Path(base path="save path", name or relative path=w1520) -> (appended path=w1519:path)
                  n795 = for {
                    tunnel: w1558 -> [w1561] mode=indexing
                    tunnel: [w1560] -> w1534 mode=indexing
                    n796 = Format Date/Time String(time format string (%c)="%Y%m%d%H%M%S", seconds (now)=w1561) -> (date/time string=w1560:string)  [unwired: 1 in]
                  }
                  n797 = Array Size(array=w1536) -> (size(s)=w1537:i32)
                  n798 = Number To Fractional String(number=w1536) -> (F-format string=w1533:string[])  [unwired: 3 in]
                  n799 = Number To Fractional String(number=w1527) -> (F-format string=w1530:string[])  [unwired: 3 in]
                  n800 = Number To Fractional String(number=w1526) -> (F-format string=w1529:string[])  [unwired: 3 in]
                  n801 = Number To Fractional String(number=w1525) -> (F-format string=w1528:string[])  [unwired: 3 in]
                  n802 = Initialize Array("", w1537, 5 ("dimension size")) -> (w1535:string[][])
                  n803 = Insert Into Array(array=w1535, index (col)=0 ("disabled index (col)"), new element=w1534) -> (w1545:string[][])  [unwired: 1 in]
                  n804 = Insert Into Array(array=w1545, index (col)=1 ("disabled index (col)"), new element=w1533) -> (w1544:string[][])  [unwired: 1 in]
                  n805 = Insert Into Array(array=w1544, index (col)=2 ("disabled index (col)"), new element=w1530) -> (w1548:string[][])  [unwired: 1 in]
                  n806 = Insert Into Array(array=w1548, index (col)=3 ("disabled index (col)"), new element=w1529) -> (w1549:string[][])  [unwired: 1 in]
                  n807 = Insert Into Array(array=w1549, index (col)=4 ("disabled index (col)"), new element=w1528) -> (w1550:string[][])  [unwired: 1 in]
                  n808 = Insert Into Array(array=w1550, index (row)=0, new element=string[] ["time", "Centroid X", "Centroid Y", "Motor Axis 1", "Motor Axis 2"] ("new element/subarray 2")) -> (w1532:string[][])  [unwired: 1 in]
                  n809 = call-poly <vilib>:"Write To Spreadsheet File.vi"("2D data"=w1532, "file path (dialog if empty)"=w1519) -> ()  [unwired: 6 in, 1 out]
                }
                frame True {
                }
              }
            }
            n810 = call <vilib>:"Add State(s) to Queue__jki_lib_state_machine.vi"("State(s) in (\"\")"=w1515) -> ("States Out"=w1514:string)  [unwired: 14 in]
            n811 = property on="Save Stats" class="Bool (strict)"("Value"=FALSE ("Save Stats")) -> ()  [unwired: 2 in, 2 out]
          }
          frame "tdms" {
            w1588 = 21600.0 ("new tdms")
            # "Your code here.\n(You can make a copy of, or modify, this frame)"
            n812 = Unbundle By Name(w1578) -> ("Data Value Reference out"=w1601:refnum<k34>, "Offset X"=w1603:dbl[][], "Offset Y"=w1598:dbl[][], "active axis refs 2"=w1600:T12)
            n813 = for {
              tunnel: w1603 -> [w1647]
              tunnel: w1598 -> [w1646]
              tunnel: w1602 -> [w1610] mode=indexing
              tunnel: w1601 -> [w1611]
              tunnel: w1600 -> [w1632]
              tunnel: w1599 -> [w1616]
              tunnel: [w1614] -> w1597
              i -> [w1633]
              n814 = Index Array(array=w1647, index (row)=w1633) -> (element=w1645:dbl[])  [unwired: 1 in]
              n815 = Index Array(array=w1646, index (row)=w1633) -> (element=w1644:dbl[])  [unwired: 1 in]
              n816 = Index Array(array=w1632, index=w1633) -> (element=w1631:cluster{"Ref X":refnum<vi>, "Ref Y":refnum<vi>})
              n817 = Reverse 1D Array(array=w1644) -> (reversed array=w1642:dbl[])
              n818 = Reverse 1D Array(array=w1645) -> (reversed array=w1643:dbl[])
              n819 = Unbundle By Name(w1631) -> ("Ref X"=w1630:refnum<vi>, "Ref Y"=w1629:refnum<vi>)
              n820 = Index Array(array=w1643) -> (element=w1641:dbl)  [unwired: 1 in]
              n821 = Index Array(array=w1642) -> (element=w1640:dbl)  [unwired: 1 in]
              n822 = property class="DigNum (strict)"(reference=w1630, error in=w1616) -> (error out=w1615:errorcluster, "Value"=w1624:dbl)  [unwired: 1 out]
              n823 = Build Array(w1641) -> (w1613:dbl[])
              n824 = Build Array(w1640) -> (w1635:dbl[])
              n825 = Get Date/Time In Seconds() -> (seconds since 1Jan1904=w1612:timestamp)
              n826 = Build Array(w1612) -> (w1608:timestamp[])
              n827 = property class="DigNum (strict)"(reference=w1629, error in=w1615) -> (error out=w1606:errorcluster, "Value"=w1618:dbl)  [unwired: 1 out]
              n828 = Build Array(w1624) -> (w1623:dbl[])
              n829 = TDMS Write(0:w1611, 5:w1610, 7:"time", 9:w1608, 11:w1606) -> (4:w1607:refnum<k34>, 15:w1605:errorcluster)  [unwired: 1 in, 2 out]
              n830 = Build Array(w1618) -> (w1617:dbl[])
              n831 = TDMS Write(0:w1607, 5:w1610, 7:"centroid X", 9:w1613, 11:w1605) -> (4:w1638:refnum<k34>, 6:w1637:string, 15:w1636:errorcluster)  [unwired: 1 in, 1 out]
              n832 = TDMS Write(0:w1638, 5:w1637, 7:"centroid Y", 9:w1635, 11:w1636) -> (4:w1627:refnum<k34>, 6:w1626:string, 15:w1628:errorcluster)  [unwired: 1 in, 1 out]
              n833 = TDMS Write(0:w1627, 5:w1626, 7:"Motor Axis 1", 9:w1623, 11:w1628) -> (4:w1622:refnum<k34>, 6:w1621:string, 15:w1619:errorcluster)  [unwired: 1 in, 1 out]
              n834 = TDMS Write(0:w1622, 5:w1621, 7:"Motor Axis 2", 9:w1617, 11:w1619) -> (15:w1614:errorcluster)  [unwired: 1 in, 3 out]
            }
            n835 = Unbundle By Name(w1578) -> ("img to avg"=w1576:i32)
            n836 = property on="millisecond timer value" class="DigNum (strict)"() -> ("Value"=w1565:u32)  [unwired: 2 in, 2 out]
            n837 = local read "millisecond timer 2"() -> (w1594:u32)
            n838 = Tick Count (ms)() -> (millisecond timer value=w1579:u32)
            n839 = call <userlib>:"Tick Count (ms)__ogtk.vi"("error in (no error)"=w1597) -> ("error out"=w1564:errorcluster, "millisecond timer value"=w1596:u32)  [unwired: 9 in]
            n840 = Subtract(x=w1579, y=w1565) -> (x-y=w1593:u32)
            n841 = Subtract(x=w1579, y=w1565) -> (x-y=w1580:u32)
            n842 = Subtract(x=w1596, y=w1594) -> (x-y=→"Waveform Chart":u32)
            n843 = Multiply(x=5.0 ("new tdms"), y=w1576) -> (x*y=w1574:dbl)
            n844 = Divide(x=w1593, y=u32 1000) -> (x/y=w1591:dbl)
            n845 = Divide(x=w1580, y=u32 1000) -> (x/y=w1582:dbl)
            n846 = Quotient & Remainder(x=w1591, y=w1588) -> (x-y*floor(x/y)=w1590:dbl)  [unwired: 1 out]
            n847 = Quotient & Remainder(x=w1582, y=w1574) -> (x-y*floor(x/y)=w1575:dbl)  [unwired: 1 out]
            "x-y*floor(x/y)" <- w1575
            n848 = Subtract(x=w1574, y=2.0) -> (x-y=w1572:dbl)
            n849 = Greater?(x=w1575, y=w1572) -> (0:w1571:bool)
            n850 = call <vilib>:"Clear Errors.vi"("error in (no error)"=w1564) -> ("error out"=w1563:errorcluster)  [unwired: 6 in]
            n851 = Subtract(x=w1588, y=20.0) -> (x-y=w1586:dbl)
            n852 = Greater?(x=w1590, y=w1586) -> (0:w1589:bool)
            n853 = Select(t="Device Ini", s=w1571, f="") -> (s? t:f=w1568:string)
            n854 = Select(t="newtdms", s=w1589, f="") -> (s? t:f=w1583:string)
            n855 = call <vilib>:"Add State(s) to Queue__jki_lib_state_machine.vi"("State(s) in (\"\")"=w1604, "State(s) at Back (\"\")"=w1583) -> ("States Out"=w1567:string)  [unwired: 13 in]
            n856 = call <vilib>:"Add State(s) to Queue__jki_lib_state_machine.vi"("State(s) in Front (\"\")"=w1568, "State(s) in (\"\")"=w1567) -> ("States Out"=w1566:string)  [unwired: 13 in]
          }
          frame "Reset History" {
            # "Your code here.\n(You can make a copy of, or modify, this frame)"
            n857 = for {
              N: 1 -> [_]
              shift-right: [w1657] -> w1649
              shift-left: timestamp[][] [] ("Time") -> [w1659]
              n858 = for {
                N: 12 -> [_]
                tunnel: w1659 -> [w1662] mode=indexing
                tunnel: [w1660] -> w1657 mode=indexing
                n859 = Get Date/Time In Seconds() -> (seconds since 1Jan1904=w1661:timestamp)
                n860 = Build Array (concatenate)(w1662, w1661) -> (w1660:timestamp[])
              }
            }
            n861 = local read "Offset X"() -> (w1648:dbl[][])
            n862 = Bundle By Name(cluster=w1653, "Offset X"=w1648, "Offset Y"=w1648, "Time"=w1649, "Motor X"=w1648) -> (w1652:T36)
            n863 = call <vilib>:"Add State(s) to Queue__jki_lib_state_machine.vi"("State(s) in (\"\")"=w1656) -> ("States Out"=w1655:string)  [unwired: 14 in]
          }
          frame "New Category: 2" {
            # "Your code here.\n(You can make a copy of, or modify, this frame)"
            n864 = call <vilib>:"Add State(s) to Queue__jki_lib_state_machine.vi"("State(s) in (\"\")"=w1666) -> ("States Out"=w1665:string)  [unwired: 14 in]
          }
          frame "ImgToAvg" {
            # "Your code here.\n(You can make a copy of, or modify, this frame)"
            n865 = Decimal String To Number(string=w1670) -> (number=w1667:i32)  [unwired: 2 in, 1 out]
            n866 = Bundle By Name(cluster=w1669, "img to avg"=w1667) -> (w1668:T36)
            n867 = call <vilib>:"Add State(s) to Queue__jki_lib_state_machine.vi"("State(s) in (\"\")"=w1673) -> ("States Out"=w1672:string)  [unwired: 14 in]
          }
          frame "newtdms" {
            # "Your code here.\n(You can make a copy of, or modify, this frame)"
            n868 = Unbundle By Name(w1693) -> ("Data Value Reference out"=w1692:refnum<k34>, "active cams"=w1687:string[])
            n869 = Get Date/Time In Seconds() -> (seconds since 1Jan1904=w1685:timestamp)
            n870 = Format Date/Time String(time format string (%c)="%Y%m%d", seconds (now)=w1685) -> (date/time string=w1683:string)  [unwired: 1 in]
            n871 = TDMS Close(8:w1691, 11:w1692) -> (0:w1678:errorcluster)  [unwired: 1 out]
            n872 = Format Date/Time String(time format string (%c)="%Y%m%d%H%M", seconds (now)=w1685) -> (date/time string=w1695:string)  [unwired: 1 in]
            n873 = Concatenate Strings(w1695, "Beampointing_Pico.tdms" ("string")) -> (w1701:string)
            n874 = String To Path(string=w1701) -> (path=w1702:path)
            n875 = Build Path(base path=w1684, name or relative path=w1683) -> (appended path=w1682:path)
            n876 = call <vilib>:"Check if File or Folder Exists.vi"("error in (no error)"=w1678, "path"=w1682) -> ("error out"=w1677:errorcluster, "file or folder exists?"=w1681:bool, "dup path"=w1680:path)  [unwired: 7 in]
            n877 = case shown="True" w1681 {
              tunnel: w1680 -> [w1709 w1711]
              tunnel: [w1708 w1711] -> w1679
              tunnel: w1677 -> [w1707 w1710]
              tunnel: [w1706 w1710] -> w1676
              frame False {
                n878 = Create Folder(path (use dialog)=w1709, error in=w1707) -> (created path=w1708:path, error out=w1706:errorcluster)  [unwired: 1 in, 1 out]
              }
              frame True {
              }
            }
            n879 = call <vilib>:"Add State(s) to Queue__jki_lib_state_machine.vi"("State(s) in (\"\")"=w1705) -> ("States Out"=w1704:string)  [unwired: 14 in]
            n880 = Build Path(base path=w1679, name or relative path=w1702) -> (appended path=w1696:path)
            n881 = TDMS Open(6:FALSE ("disable buffering (T)"), 7:enum16{"1.0", "2.0"}."2.0" ("file format version (2.0)"), 8:w1676, 10:T17."create or replace" ("operation"), 11:w1696) -> (0:w1688:errorcluster, 3:w1690:refnum<k34>)  [unwired: 2 in]
            n882 = call "TDMSbuffersize.vi"("error in (no error)"=w1688, "group names"=w1687, "Data Value Reference in"=w1690) -> ("error out"=w1675:errorcluster, "Data Value Reference out"=w1689:refnum<k34>)  [unwired: 7 in]
            n883 = Bundle By Name(cluster=w1693, "Data Value Reference out"=w1689) -> (w1694:T36)
            n884 = call <vilib>:"Clear Errors.vi"("error in (no error)"=w1675) -> ("error out"=w1674:errorcluster)  [unwired: 6 in]
          }
          frame "Center" {
            # "Your code here.\n(You can make a copy of, or modify, this frame)"
            n885 = property on="Center" class="Bool (strict)"("Value"=FALSE ("Center")) -> ()  [unwired: 2 in, 2 out]
            n886 = control-ref of="image::1"() -> (w1726:refnum<vi>)
            n887 = control-ref of="image::2"() -> (w1725:refnum<vi>)
            n888 = control-ref of="image::3"() -> (w1724:refnum<vi>)
            n889 = control-ref of="image::4"() -> (w1723:refnum<vi>)
            n890 = control-ref of="image::5"() -> (w1722:refnum<vi>)
            n891 = control-ref of="image::6"() -> (w1721:refnum<vi>)
            n892 = control-ref of="image::7"() -> (w1720:refnum<vi>)
            n893 = control-ref of="image::8"() -> (w1719:refnum<vi>)
            n894 = control-ref of="image::9"() -> (w1718:refnum<vi>)
            n895 = control-ref of="image::10"() -> (w1717:refnum<vi>)
            n896 = control-ref of="image::11"() -> (w1716:refnum<vi>)
            n897 = control-ref of="image::12"() -> (w1715:refnum<vi>)
            n898 = for {
              tunnel: w1712 -> [w1739] mode=indexing
              tunnel: [w1734] -> w1727 mode=indexing
              n899 = Unbundle By Name(w1739) -> ("Target.X::12"=w1738:refnum<vi>, "Target.Y::12"=w1737:refnum<vi>)
              n900 = property class="DigNum (strict)"(reference=w1738) -> ("Value"=w1736:dbl)  [unwired: 1 in, 2 out]
              n901 = property class="DigNum (strict)"(reference=w1737) -> ("Value"=w1735:dbl)  [unwired: 1 in, 2 out]
              n902 = Bundle("Value"=w1736, "Value"=w1735) -> (w1734:cluster{"Value":dbl, "Value":dbl})  [unwired: 1 in]
            }
            n903 = call <vilib>:"Add State(s) to Queue__jki_lib_state_machine.vi"("State(s) in (\"\")"=w1731) -> ("States Out"=w1730:string)  [unwired: 14 in]
            n904 = Build Array(w1726, w1725, w1724, w1723, w1722, w1721, w1720, w1719, w1718, w1717, w1716, w1715) -> (w1714:refnum<vi>[])
            n905 = for {
              tunnel: w1714 -> [w1733] mode=indexing
              tunnel: w1727 -> [w1732] mode=indexing
              n906 = property class="ImageControl"(reference=w1733, "Image Center Position"=w1732) -> ()  [unwired: 1 in, 2 out]
            }
          }
          frame "history" {
            # "Your code here.\n(You can make a copy of, or modify, this frame)"
            n907 = Unbundle By Name(w1749) -> ("Offset X"=w1755:dbl[][], "Offset Y"=w1754:dbl[][], "Mean Centroid X"=w1753:dbl[][], "Mean Centroid Y"=w1752:dbl[][], "Motor X"=w1751:dbl[][], "Motor Y"=w1750:dbl[][], "Time"=w1741:timestamp[][])
            n908 = for {
              tunnel: w1755 -> [w1773] mode=indexing
              tunnel: w1754 -> [w1771] mode=indexing
              tunnel: w1753 -> [w1770] mode=indexing
              tunnel: w1752 -> [w1769] mode=indexing
              tunnel: w1751 -> [w1768] mode=indexing
              tunnel: w1750 -> [w1767] mode=indexing
              tunnel: [w1772] -> w1747 mode=indexing
              tunnel: [w1766] -> w1746 mode=indexing
              tunnel: [w1762] -> w1745 mode=indexing
              tunnel: [w1765] -> w1744 mode=indexing
              tunnel: [w1764] -> w1743 mode=indexing
              tunnel: [w1763] -> w1742 mode=indexing
              tunnel: w1741 -> [w1761] mode=indexing
              tunnel: [w1759] -> w1740 mode=indexing
              w1760 = 0
              n909 = Delete From Array(array=w1768, index=w1760) -> (array with subset deleted=w1764:dbl[])  [unwired: 1 in, 1 out]
              n910 = Delete From Array(array=w1767, index=w1760) -> (array with subset deleted=w1763:dbl[])  [unwired: 1 in, 1 out]
              n911 = Delete From Array(array=w1761, index=w1760) -> (array with subset deleted=w1759:timestamp[])  [unwired: 1 in, 1 out]
              n912 = Delete From Array(array=w1770, index=w1760) -> (array with subset deleted=w1762:dbl[])  [unwired: 1 in, 1 out]
              n913 = Delete From Array(array=w1769, index=w1760) -> (array with subset deleted=w1765:dbl[])  [unwired: 1 in, 1 out]
              n914 = Delete From Array(array=w1771, index=w1760) -> (array with subset deleted=w1766:dbl[])  [unwired: 1 in, 1 out]
              n915 = Delete From Array(array=w1773, index=w1760) -> (array with subset deleted=w1772:dbl[])  [unwired: 1 in, 1 out]
            }
            n916 = call <vilib>:"Add State(s) to Queue__jki_lib_state_machine.vi"("State(s) in (\"\")"=w1758) -> ("States Out"=w1757:string)  [unwired: 14 in]
            n917 = Bundle By Name(cluster=w1749, "Offset X"=w1747, "Offset Y"=w1746, "Mean Centroid X"=w1745, "Mean Centroid Y"=w1744, "Motor X"=w1743, "Motor Y"=w1742, "Time"=w1740) -> (w1748:T36)
          }
        }
        n918 = property on="Box" class="Arr (strict)"() -> ("Value"=w261:T6)  [unwired: 2 in, 2 out]
        n919 = for {
          tunnel: w263 -> [w288]
          tunnel: w262 -> [w289]
          tunnel: w254 -> [w281] mode=indexing
          tunnel: w261 -> [w282] mode=indexing
          n920 = call-poly <userlib>:"Filter 1D Array__ogtk.vi"("items to filter"=w281, "array"=w289) -> ("filtered item indices"=w290:i32[])  [unwired: 4 in, 1 out]
          n921 = Index Array(array=w290) -> (element=w284:i32)  [unwired: 1 in]
          n922 = Index Array(array=w288, index=w284) -> (element=w287:T30)
          n923 = Unbundle By Name(w287) -> ("Target.X::12"=w292:refnum<vi>, "Target.Y::12"=w291:refnum<vi>)
          n924 = property class="DigNum (strict)"(reference=w292) -> ("Value"=w286:dbl)  [unwired: 1 in, 2 out]
          n925 = property class="DigNum (strict)"(reference=w291) -> ("Value"=w285:dbl)  [unwired: 1 in, 2 out]
          n926 = call "draw crosshair imaq.vi"("Color"=u32 16774656, "Target.Y"=w285, "size"=cluster{"xhair size":dbl, "xhair size 2":dbl} {"xhair size"=25.0, "xhair size 2"=25.0}, "Target.X"=w286, "Bounding Rectangle"=T15 {"Left"=0, "Top"=0, "Right"=0, "Bottom"=0}, "image in"=w281) -> ("error out"=→"error out":errorcluster, "image out"=w280:T9)  [unwired: 4 in]
          n927 = call "draw box imaq.vi"("Color"=u32 1244928, "Rectangle"=w282, "image in"=w280) -> ()  [unwired: 8 in, 1 out]
        }
        n928 = property on="ActiveMotor" class="Ring (strict)"() -> ("Strings []"=w256:string[])  [unwired: 2 in, 2 out]
        n929 = Index Array(array=w256, index="ActiveMotor") -> (element=w257:string)
        n930 = Not Equal?(x="ActiveMotorName::99", y=w257) -> (x != y?=w258:bool)
        n931 = case shown="True" w258 {
          tunnel: w256 -> [_ w277]
          tunnel: "ActiveMotorName::99" -> [_ w276]
          frame False {
          }
          frame True {
            n932 = Search 1D Array(1D array=w277, element=w276) -> (index of element=w275:i32)  [unwired: 1 in]
            n933 = property on="ActiveMotor" class="Ring (strict)"("Value"=w275) -> ()  [unwired: 2 in, 2 out]
          }
        }
      }
      n934 = control-ref of="This Application"() -> (w243:refnum<vi>)
      n935 = control-ref of="This VI"() -> (w247:refnum<vi>)
      n936 = Current VI's Menubar() -> (w246:refnum<k9>)
      n937 = call "GUI_Master_subvi_reentrant_queues.vi"("This Application"=w243, "error in (no error)"=w244, "tcp data event"=w242, "Caller menu reference"=w246, "Caller VI ref"=w247) -> ("error out"=→"error IO 2":errorcluster)  [unwired: 6 in]
      n938 = Unbundle By Name(w132) -> ("Data Value Reference out"=w131:refnum<k34>)
      n939 = for {
        tunnel: w161 -> [w251] mode=indexing
        tunnel: w160 -> [w250]
        tunnel: [w249] -> w130
        n940 = call "IMAQ Dispose"("Image"=w251, "error in (no error)"=w250) -> ("error out"=w249:errorcluster)  [unwired: 4 in]
      }
      n941 = TDMS Close(8:w130, 11:w131) -> (0:→"error out 2":errorcluster)  [unwired: 1 out]
    }
  }
